vi "myRIO_BRig_RT_v0,62__PortC.vi"() -> ()   [LabVIEW 2014]
uses:
  myRIO_BRig_RT__Case_Exp_stateList.ctl
  myRIO_BRig_RT__Case_NonExp_stateList.ctl
  <vilib>/Platform/TimedLoop/XDataNode/timing_clust.ctl
  <vilib>/Platform/TimedLoop/XDataNode/nitl_modes.ctl
  <vilib>/Platform/TimedLoop/XDataNode/wakeup.ctl
  <vilib>/WebDAVClient/Advanced/SessionHandle.ctl
  <vilib>/myRIO/Common/Instrument Driver Framework/myRIO v1.0/UART/vis/myRIO v1.0 Close UART.vi
  <vilib>/FPGAPlugInAG/myRIO-1900/niLvFpga_Open_myRIO-1900.vi
  <vilib>/rvi/interface/common/dynamic/niFpgaDynamicAddResources.vi
  <vilib>/Utility/error.llb/Error Cluster From Error Code.vi
  <vilib>/rvi/errors/niLvFpgaAdjustHostInterfaceError.vi
  <vilib>/FPGAPlugInAG/Dynamic/niLvFpga_Close_Dynamic.vi
  <vilib>/myRIO/Common/Instrument Driver Framework/Utilities/vis/FPGA Ref Manager.vi
  <vilib>/myRIO/Common/Instrument Driver Framework/myRIO v1.0/myRIO v1.0 Reset FPGA.vi
  <vilib>/myRIO/Common/Instrument Driver Framework/myRIO v1.0/IRQ/vis/myRIO v1.0 IRQ Info FGV.vi
  <vilib>/myRIO/Common/Instrument Driver Framework/myRIO v1.0/IRQ/vis/myRIO v1.0 Timer IRQ Info FGV.vi
  <vilib>/myRIO/Common/Instrument Driver Framework/myRIO v1.0/IRQ/vis/myRIO v1.0 ISR Agent.vi
  <vilib>/rvi/interface/nirviOpenFPGA/nirviOpenFPGA.xnode
  myRIO_BRig_FPGA_v3,52__PortC__build.lvbitx
  myRIO_BRig_FPGA_v3,52__PortC.vi
  <vilib>/rvi/interface/nirviReadWriteControl/nirviReadWriteControl.xnode
  <vilib>/Platform/TimedLoop/XDataNode/XDataNode.xnode
  <vilib>/rvi/interface/nirviCloseFPGA/nirviCloseFPGA.xnode
  <vilib>/Platform/TimedLoop/XDataNode/XDNodeRunTimeDep.lvlib
  <vilib>/rvi/interface/Simulation/niFpgaSimulationCallBeginRW.vi
  <vilib>/myRIO/Instrument Drivers/Utilities/Utilities.lvlib
  <vilib>/WebDAVClient/NI_WebDAV.lvlib
  NiFpgaLv.dll
panel:
  out "error out 5":errorcluster
  in  "get_countPerMS":bool
  in  "count_warmup_R_reset":bool
  in  "count_warmup_L_reset":bool
  out "count_warmup_R":u16
  out "count_warmup_L":u16
  out "SolenoidReward":bool
  in  "SolenoidProbability_L":u16=50 caption="Reward Time [ms]" min=1 max=1000 step=1
  in  "SolenoidProbability_R":u16=50 caption="Reward Time [ms]" min=1 max=1000 step=1
  out "output_PortA":dbl
  out "error out 4":errorcluster
  in  "laser_power_step":dbl
  in  "laser_power_max":dbl
  in  "Recording_p2":bool
  in  "Recording":bool
  out "error out 3":errorcluster
  out "error out 2":errorcluster
  in  "laser_power_min":dbl
  in  "f_millisec2count":dbl=159.0
  in  "laser_Tshutter":dbl=2.0
  in  "laser_Freq":dbl=10.0
  in  "laser_Tpeak":dbl=2.0
  in  "laser_duration":u16
  out "error out":errorcluster
  in  "LC_Cue1_All_Count":u16
  in  "LC_Cue1_First_Count":u16
  in  "LC_Cue1_All_delayOpt":bool
  in  "LC_ENL1_All_delayOpt":bool
  in  "LC_ENL1_All_Count":u16
  in  "LC_ENL1_First_Count":u16
  in  "LC_Cue1_First_delayOpt":bool
  in  "LC_ENL1_First_delayOpt":bool
  in  "Tcycle_Cue_max":u16=1000 caption="Max" min=5 max=5000 step=5
  in  "Tcycle_Cue_min":u16=1000 caption="Min" min=5 max=5000 step=5
  in  "SendData":bool
  out "cSpout":enum16{"Left", "Right"}(ring) caption="Left or Right Spout"
  out "A4":u32 caption="LickCounter_Right"
  out "A2":u32 caption="LickCounter_Left"
  in  "laserResponse_wrong_LED":bool
  out "error_initTrial":errorcluster
  out "error_Selection_pre":errorcluster
  out "error_Selection":errorcluster
  out "SelectWrong":bool
  out "SelectReward":bool
  in  "Left(F)_or_Right(T)":bool
  in  "ignoreWrong":bool
  in  "SelectionState":bool
  in  "laserResponse_wrong":bool
  in  "laserResponse_reward":bool
  in  "laserResponse_reward_LED":bool
  out "nRewards_Right":u16 caption="# Rewards Total (Right)"
  out "nRewards_Left":u16 caption="# Rewards Total (Left)"
  out "nRewards_cur":u16 caption="# Rewards in Current Block"
  out "TpB_target":u16 caption="Target Trials Per Block"
  out "cState_NonExp":T1 caption="WarmUp State"
  out "iBlock":u16 caption="Current Block"
  out "cState":T2 caption="Experimental State"
  out "iTrial":u16 caption="Current Trial"
  in  "warmupType":u8(slide) max=2 step=1 scale=0.0..2.0
  in  "TestConnection":bool
  in  "warmup":bool caption="WarmUp"
  in  "Data Set Prefix":string="Exp1_TM2"
  out "Connected To Host?":bool
  in  "Host Password":string="sabalab"
  in  "Host UserName":string="Test2"
  in  "sp_RightSpout":u16(slide)=2 max=2 step=1 scale=0.0..2.0
  in  "sp_LeftSpout":u16(slide)=2 max=2 step=1 scale=0.0..2.0
  in  "BUR_max":u16 caption="Count Reward Structure  (0 = off)"
  in  "LC_Wrong_Probability":u16
  in  "LC_Wrong_Trial":u16(slide) max=2 step=1 scale=0.0..2.0
  in  "LC_Wrong_Block":u16(slide) max=2 step=1 scale=0.0..2.0
  in  "LC_Wrong_OnOff":bool
  in  "LC_Reward_Probability":u16
  in  "LC_Reward_Trial":u16(slide) max=2 step=1 scale=0.0..2.0
  in  "LC_Reward_Block":u16(slide) max=2 step=1 scale=0.0..2.0
  in  "LC_Reward_OnOff":bool
  in  "LC_Cue1_All_Probability":u16
  in  "LC_Cue1_All_Block":u16(slide) max=2 step=1 scale=0.0..2.0
  in  "LC_Cue1_All_OnOff":bool
  in  "LC_Cue1_First_Probability":u16
  in  "LC_Cue1_First_Block":u16(slide) max=2 step=1 scale=0.0..2.0
  in  "LC_Cue1_First_OnOff":bool
  in  "LC_ENL1_All_Probability":u16 max=100 step=1
  in  "LC_ENL1_All_Block":u16(slide) max=2 step=1 scale=0.0..2.0
  in  "LC_ENL1_All_OnOff":bool
  in  "LC_ENL1_First_Probability":u16 max=100 step=1
  in  "LC_ENL1_First_Block":u16(slide) max=2 step=1 scale=0.0..2.0
  in  "Tcycle_Timeout":u16=1000 caption="Timeout Time [ms]" min=10 max=10000 step=1
  in  "Tcycle_Wrong":u16=1000 caption="Wrong Time [ms]" min=10 max=10000 step=1
  in  "Tcycle_Selection":u16=1000 caption="Answer Time [ms]" min=1 max=10000 step=1
  in  "Tcycle_RewardPost":u16=1000 caption="Consumption Time [ms]" min=250 max=10000 step=250
  in  "Tcycle_Reward_L":u16=500 caption="Reward Time [ms]" min=1 max=1000 step=1
  in  "Tcycle_Reward_R":u16=500 caption="Reward Time [ms]" min=1 max=1000 step=1
  in  "TpB_Max_R":u16=4 caption="Max TrialsPerBlock" min=1 max=12 step=1
  in  "TpB_Min_R":u16=4 caption="Min TrialsPerBlock" min=1 max=12 step=1
  in  "TpB_Max_L":u16=4 caption="Max TrialsPerBlock" min=1 max=12 step=1
  in  "TpB_Min_L":u16=4 caption="Min TrialsPerBlock" min=1 max=12 step=1
  in  "BUR_min":u16 caption="Count Reward Structure  (0 = off)"
  in  "TrialUntilReward":bool caption="Ignore Wrong Selection"
  in  "CueCycles":u16=1 caption="Cue Structure" min=1 max=1 step=1
  in  "MTrig_Laser_Tcycle":u16=10 caption="Time [ms]"
  in  "MTrig_Laser_trig":bool
  in  "MTrig_Audio_trig__R":bool caption="Trigger Audio"
  in  "MTrig_Audio_trig__L":bool caption="Trigger Audio"
  in  "RewCalib_Trig_R":bool caption="Calibrate_R"
  in  "RewCalib_Trig_L":bool caption="Calibrate_L"
  in  "MTrig_Solenoid_Tcycle__R":u16=300 caption="Time [ms]"
  in  "MTrig_Solenoid_Tcycle__L":u16=300 caption="Time [ms]"
  in  "MTrig_Solenoid_trig__R":bool caption="Solenoid"
  in  "MTrig_Solenoid_trig__L":bool caption="Solenoid"
  in  "STOP_abort":bool caption="Stop LabView\n(Stops myRio and FPGA)"
  in  "STOP_endBlock":bool caption="Stop Experiment\n@ End of Block"
  in  "STOP_endTrial":bool caption="Stop Experiment\n@ End of Trial"
  in  "START":bool caption="Start Experiment"
  in  "Tcycle_CuePenalty":u16=1000 caption="Penalty" min=1 max=10000 step=1
  in  "Audio_Amp__R":u16=100 caption="Amp"
  in  "Audio_Freq__R":u8=5 caption="Freq [kHz]" max=14 step=1
  in  "Audio_Amp__L":u16=100 caption="Amp"
  in  "Audio_Freq__L":u8=5 caption="Freq [kHz]" max=14 step=1
  in  "LC_Wrong_Tdelay":u16
  in  "LC_Cue1_All_Tdelay":u16
  in  "LC_ENL1_All_Tdelay":u16
  in  "LC_Reward_Tdelay":u16
  in  "LC_Cue1_First_Tdelay":u16
  in  "LC_ENL1_First_Tdelay":u16
  in  "LC_ENL1_First_OnOff":bool
  in  "Tcycle_ENLPenalty":u16=100 caption="Penalty" min=10 max=10000 step=10
  in  "Tcycle_ENL_max":u16=1000 caption="Max" min=250 max=10000 step=250
  in  "Tcycle_ENL_min":u16=1000 caption="Min" min=250 max=10000 step=250
  # "Communication (Host PC)"
  # "WarmUp"
  # "Experimental Run"
  # "Current State"
  # "Laser Control\n\n                               On/Off      Block        Probability [%]   Delay [ms]                              Count"
  # "Cue then reward (no lick)\n \nLeft                    Right"
  # "Recording Rig"
  # "FPGA Conv."
  # "Enforced\nNonLick\n      1"
  # "from end"
  # "Switch\nTrial"
  # "FPGA count per ms"
  # "from start"
  # "from end"
  # "NonSwitch\nTrials"
  # "from start"
  # "Manual Control"
  # "Cue 1"
  # "Solenoid\n \nLeft                    Right"
  # "Speaker\n \nLeft                    Right"
  # "Laser"
  # "from end"
  # "Switch\nTrial"
  # "from start"
  # "from end"
  # "NonSwitch\nTrials"
  # "from start"
  # "Time = Cue Min"
  # "Selection Reward"
  # "Power = Min"
  # "Task Timing [ms]"
  # "Speaker Settings"
  # "Laser Settings"
  # "Selection Wrong"
  # "Left                  Right"
  # "Enforced NonLick"
  # "Frequency\n[kHz]"
  # "Duration         Frequency       Peak Width           Shutter\n    [ms]                   [Hz]                    [ms]                    [ms]"
  # "Task Structure"
  # "Spout Selection Control"
  # "Amp\n(0 - 32,000)"
  # "Master Structure"
  # "Cue"
  # "Answer Time\n         [ms]\n\n  \nWrong Choice Penalty\n         [ms]\n \n \nChoice Timeout Penalty\n         [ms]"
  # "Min\n \n  \nMax"
  # "Laser Power [V]\n      Min                   Max                   Step                 Current"
  # "Speaker\nPattern\nDuring Cue"
  # "(1) = Switching\n(2) = Two Choice"
  # "Reward Control\n                 Left              Right"
  # "Min"
  # "Max"
  # "Trial Per Block Structure\n       Left                    Right"
  # "Reward Time\n         [ms]\n\nWater Prob"
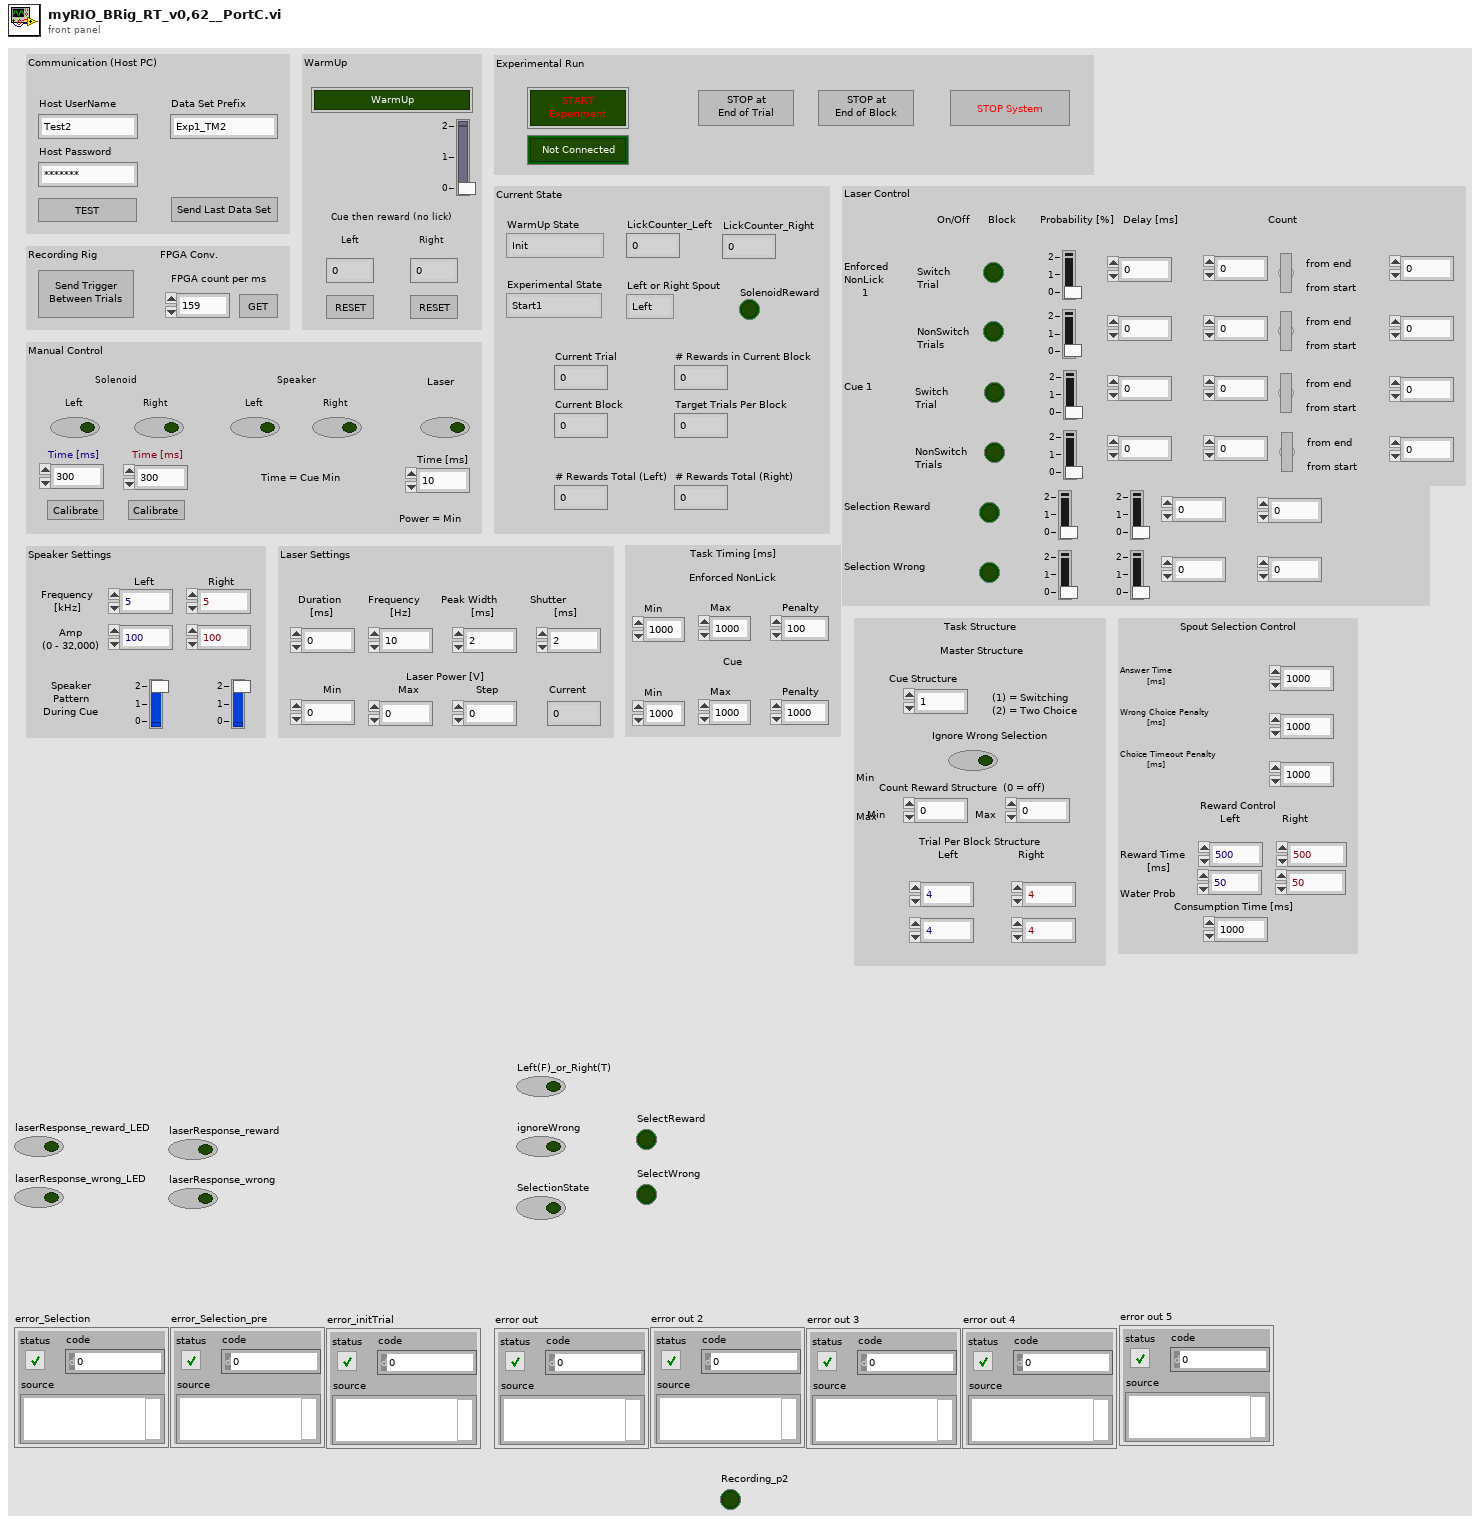
[diagram p1: front panel]
types:
  T1 = typedef "myRIO_BRig_RT__Case_NonExp_stateList.ctl" = enum16{"Init", "UploadSettings_pre", "UploadSettings_Read_dataExp", "UploadSettings_dataExp_1", "UploadSettings_Read_dataLC", "UploadSettings_dataLC_1", "UploadSettings_dataLC_2", "UploadSettings_Read_dataMTrig", "UploadSettings_dataMTrig_1", "UploadSettings_post", "Idle_pre", "IdleEmpty", "IdleEmpty2", "IdleEmpty3", "IdleEmpty4", "Idle", "Idle_2", "Idle_3", "Idle_4", "Idle_post", "Cue_pre__pre", "Cue_pre", "Cue", "Cue_post", "RewardCalibration_pre", "DispenseWater_pre__pre", "DispenseWater_pre", "DispenseWater", "DispenseWater_post", "TestConnection", "SendData", "Get_FPGA_count_per_ms", "End"}
  T2 = typedef "myRIO_BRig_RT__Case_Exp_stateList.ctl" = enum16{"Start1", "Start2", "Start3", "saveSettings1", "saveSettings2", "saveSettings3", "saveSettings4_LC_ENL", "saveSettings5_LC_Cue", "saveSettings6_LC_Other", "setSettings_Audio", "setSettings_Laser", "initBlock_pre", "initBlock", "initBlock2", "initBlock_post", "initTrial_pre", "initTrial", "initTrial2", "initTrial3", "initTrial4", "initTrial_LC_ENL1", "initTrial_LC_Cue1", "initTrial_post", "ENL1_pre", "ENL1", "ENL1_post", "ENL1Penalty_pre", "ENL1Penalty", "ENL2_pre", "ENL2", "ENL2Penalty_pre", "ENL2Penalty", "Cue1_pre", "Cue1", "Cue1_post", "Cue1Penalty_pre", "Cue1Penalty", "Cue2_pre", "Cue2", "Cue2Penalty_pre", "Cue2Penalty", "Selection_pre", "Selection", "Select_post", "SelectReward_pre", "SelectReward", "SelectRewardPost_pre", "SelectRewardPost", "SelectWrong_pre", "SelectWrong", "SelectWrong_post", "SelectTimeout_pre", "SelectTimeout", "SelectTimeout_post", "endTrial_pre", "endTrial1", "endTrial2", "endTrial3", "endTrial_post", "endBlock_pre", "endBlock", "endBlock_post", "endExp", "commConnect", "commUpload_pre", "commUpload_dataBlock", "commUpload_dataCurrent", "commUpload_dataExp", "commUpload_dataLC", "commUpload_dataTrial", "commUpload_post", "saveData_pre", "saveData_dataBlock", "saveData_dataCurrent", "saveData_dataExp", "saveData_dataLC", "saveData_dataTrial", "saveData_post", "empty_endBlock1", "empty_endBlock2", "empty_endTrial1", "empty_endTrial2", "empty_endTrial3", "empty_endTrial4", "empty_endTrial5"}
  T3 = typedef "XDNodeRunTimeDep.lvlib/timing_clust.ctl" = cluster{"Expected End [f-1]":u64, "Actual End [f-1]":u64, "Finished Late? [f-1]":bool, "Expected End [i-1]":u64, "Actual End [i-1]":u64, "Finished Late? [i-1]":bool, "Expected Start [i]":u64, "Actual Start [i]":u64, "Expected Start [f]":u64, "Actual Start [f]":u64, "Source Name":string, "Structure Name":string, "Period":i64, "Deadline":i64, "Offset":i64, "Start":i64, "Priority":i32, "Timeout":i32, "Mode":T4, "Wakeup Reason":T5, "Error":errorcluster, "Source Type":string, "Secondary Source Type":string, "Global End Time":u64, "Global Start Time":u64, "Frame Duration":u64, "Iteration Duration":u64, "Assigned CPU":i32, "I/O Scan Engine Mode":u32}
  T4 = typedef "XDNodeRunTimeDep.lvlib/nitl_modes.ctl" = enum32{"No Change", "Process missed periods, maintain original phase", "Discard missed periods, maintain original phase", "Process missed periods, ignore original phase", "Discard missed periods, ignore original phase"}
  T5 = typedef "XDNodeRunTimeDep.lvlib/wakeup.ctl" = enum32{"Normal", "Aborted", "Asynchronous wakeup", "Timing source error", "Timed loop error", "Timeout"}
  T6 = typedef "NI_WebDAV.lvlib/SessionHandle.ctl" = refnum<k1>
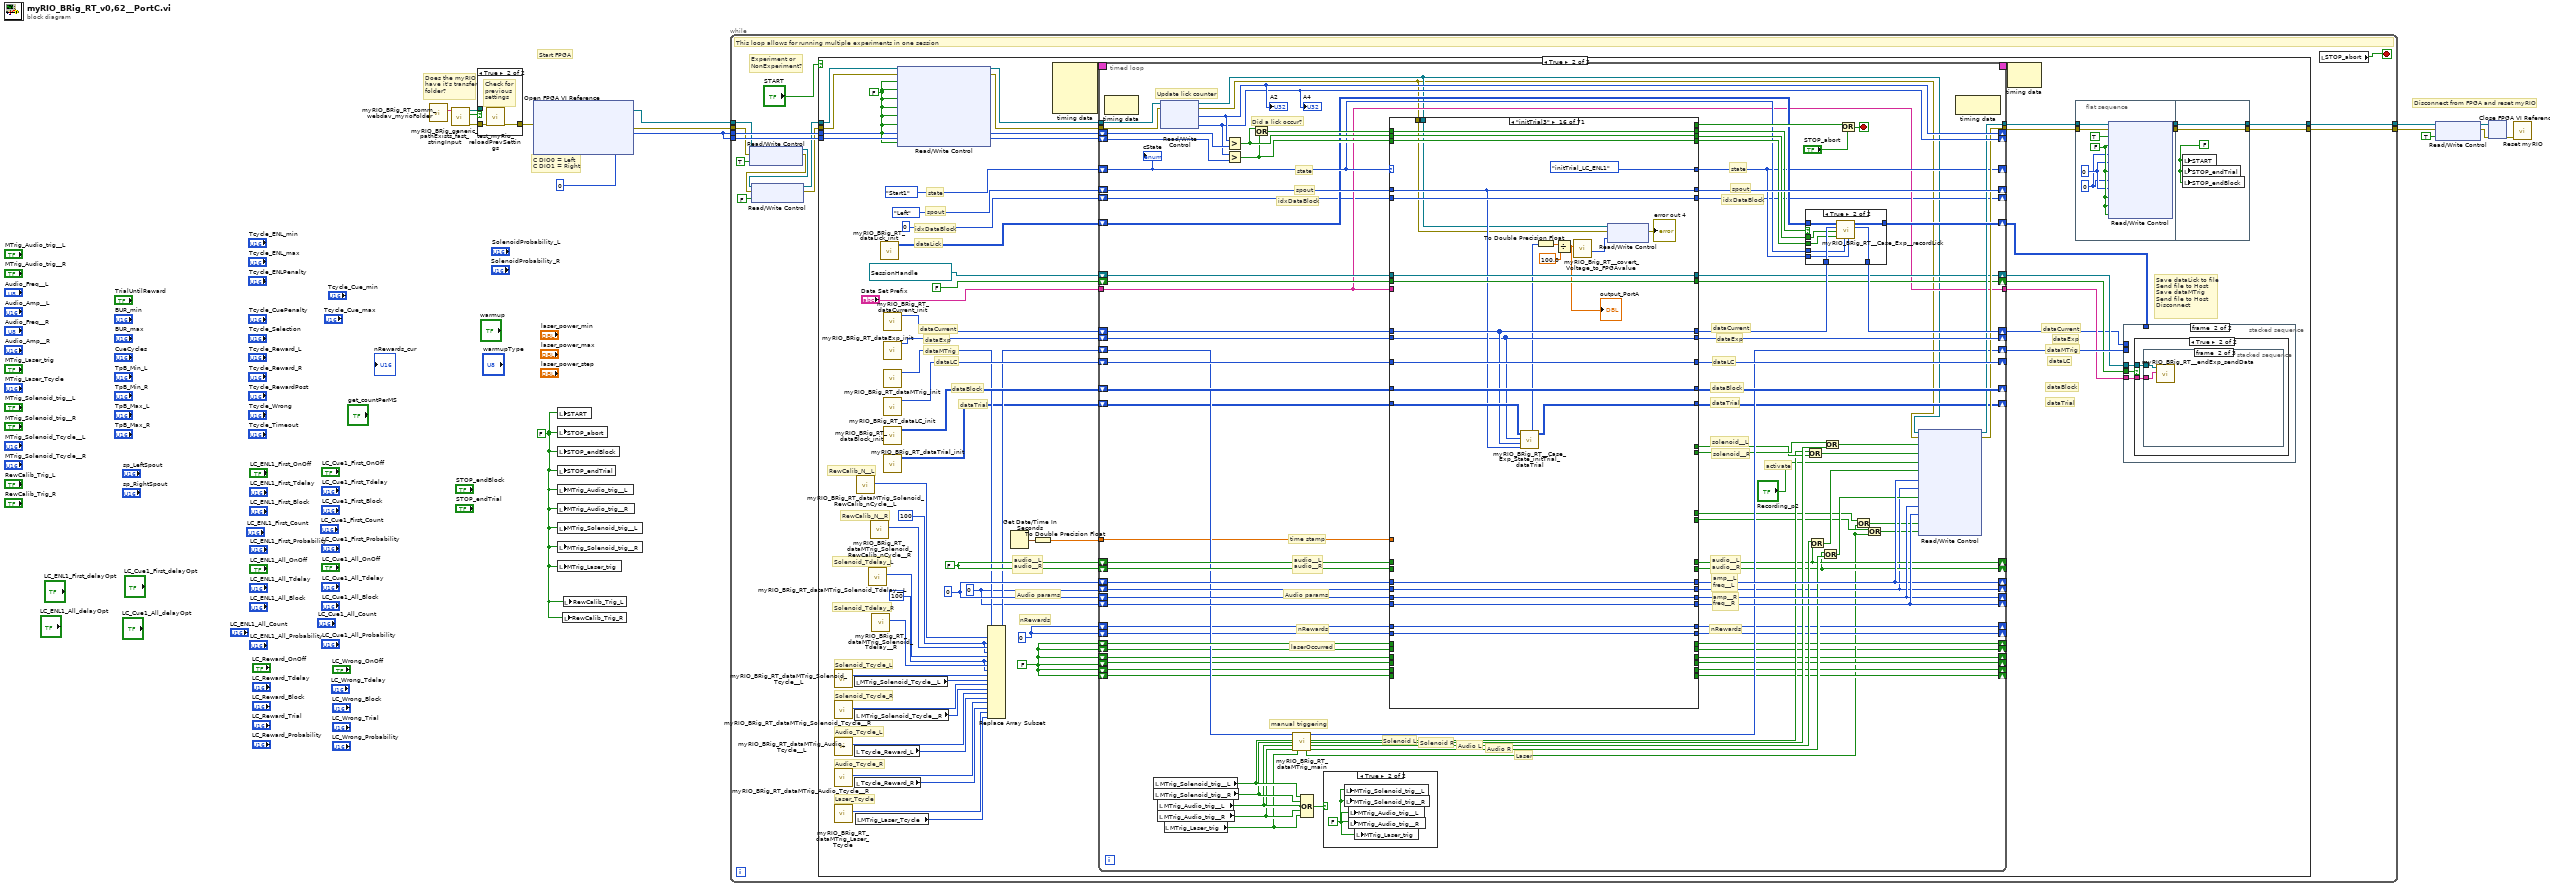
[diagram p0: block diagram]
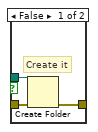
[diagram p2: hidden frame]
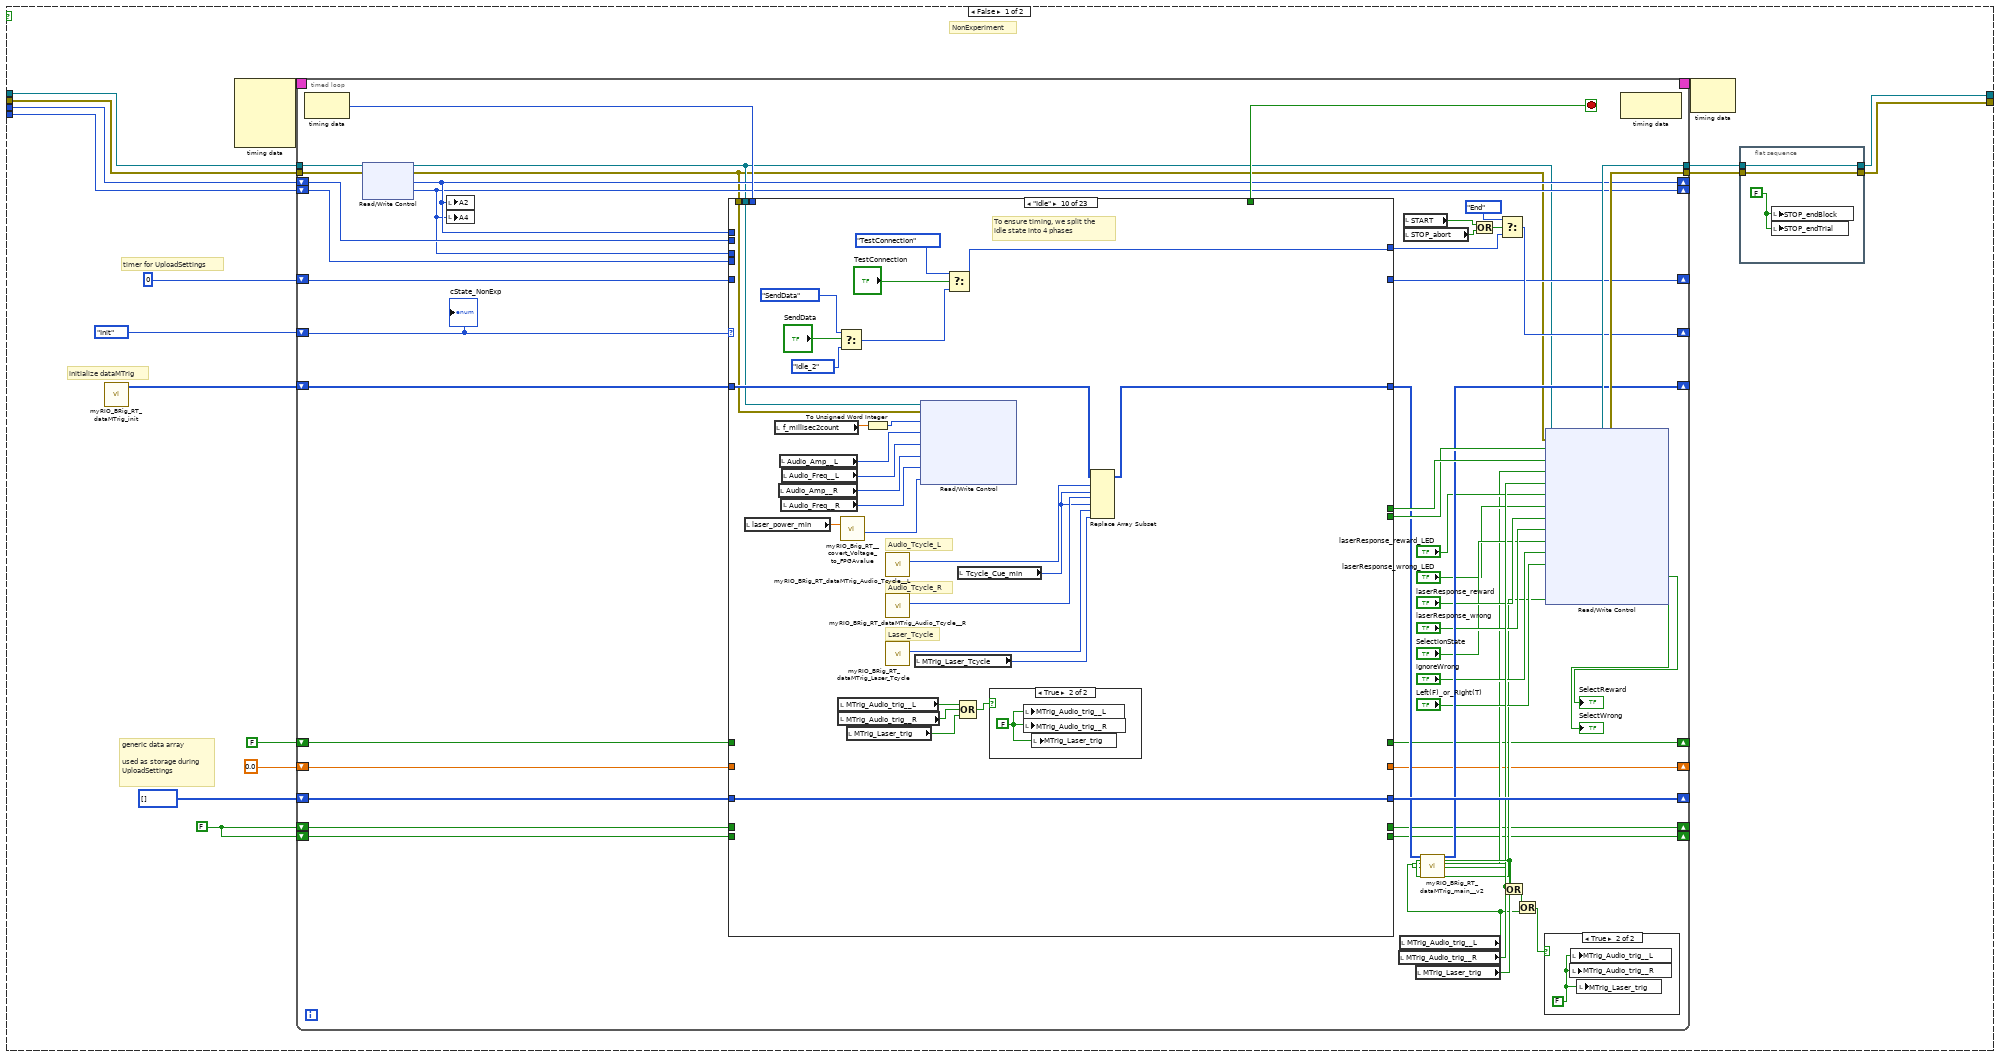
[diagram p3: hidden frame]
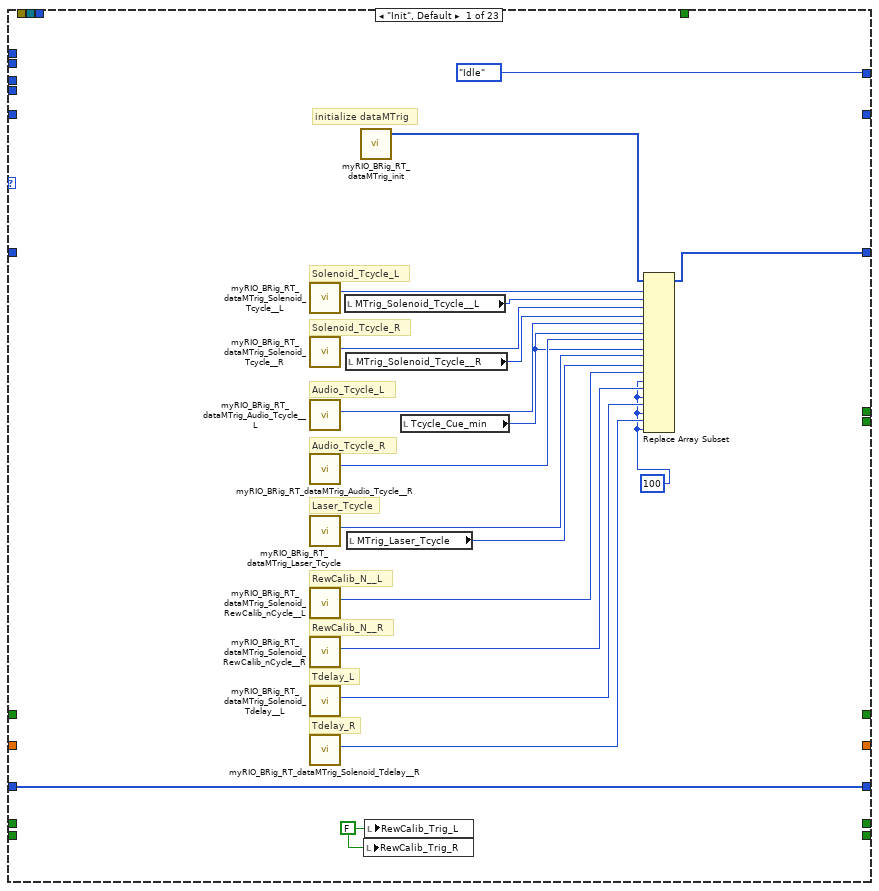
[diagram p5: hidden frame]
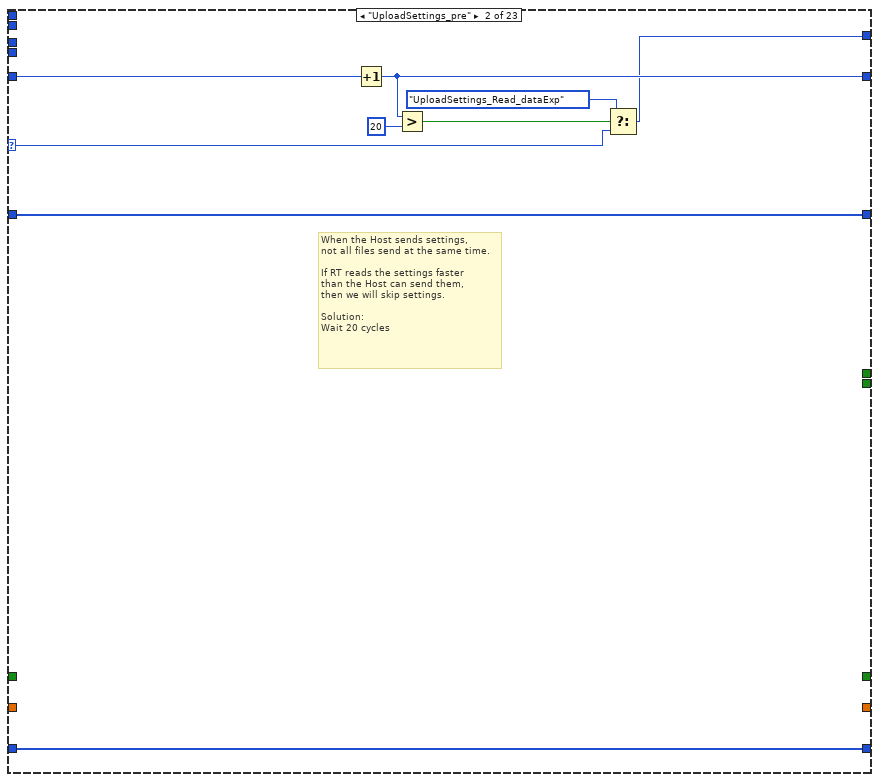
[diagram p6: hidden frame]
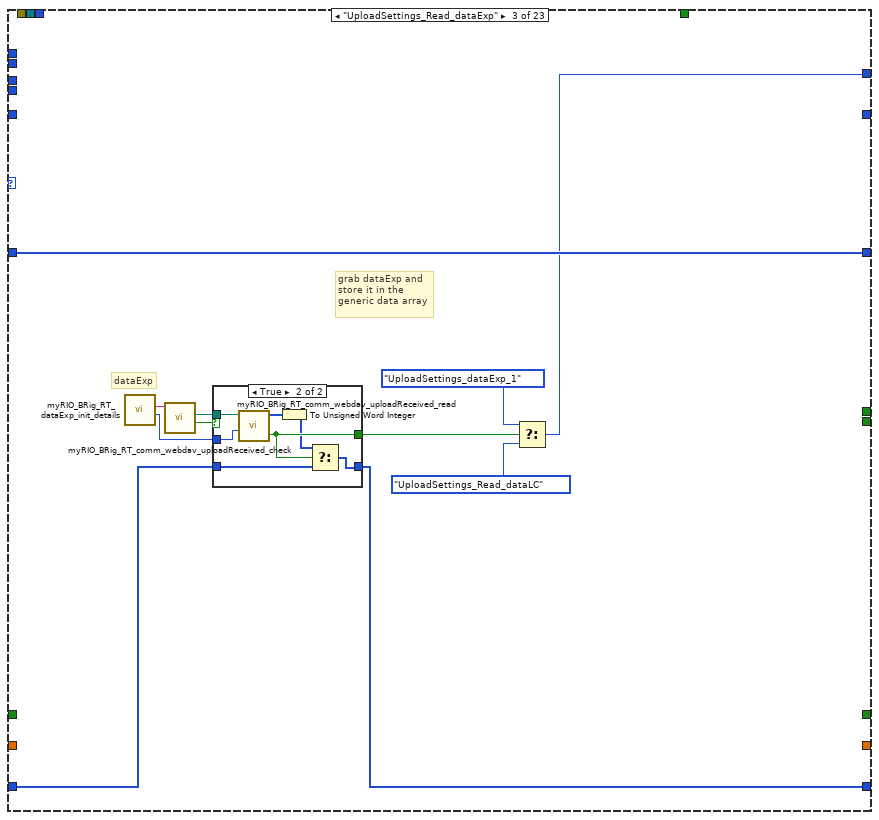
[diagram p7: hidden frame]
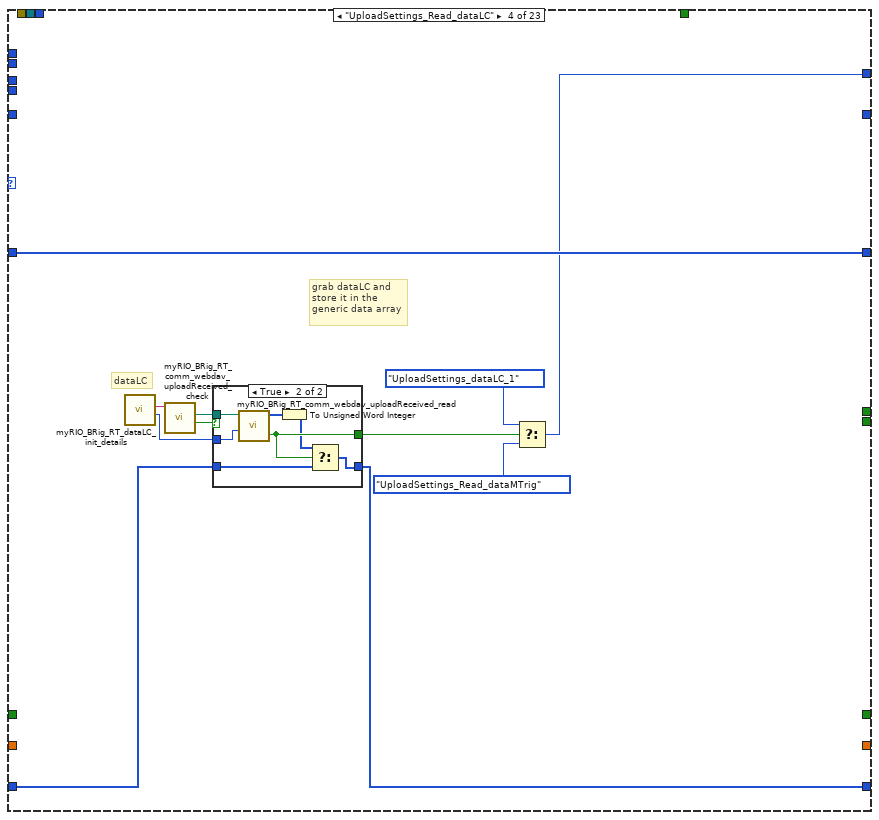
[diagram p9: hidden frame]
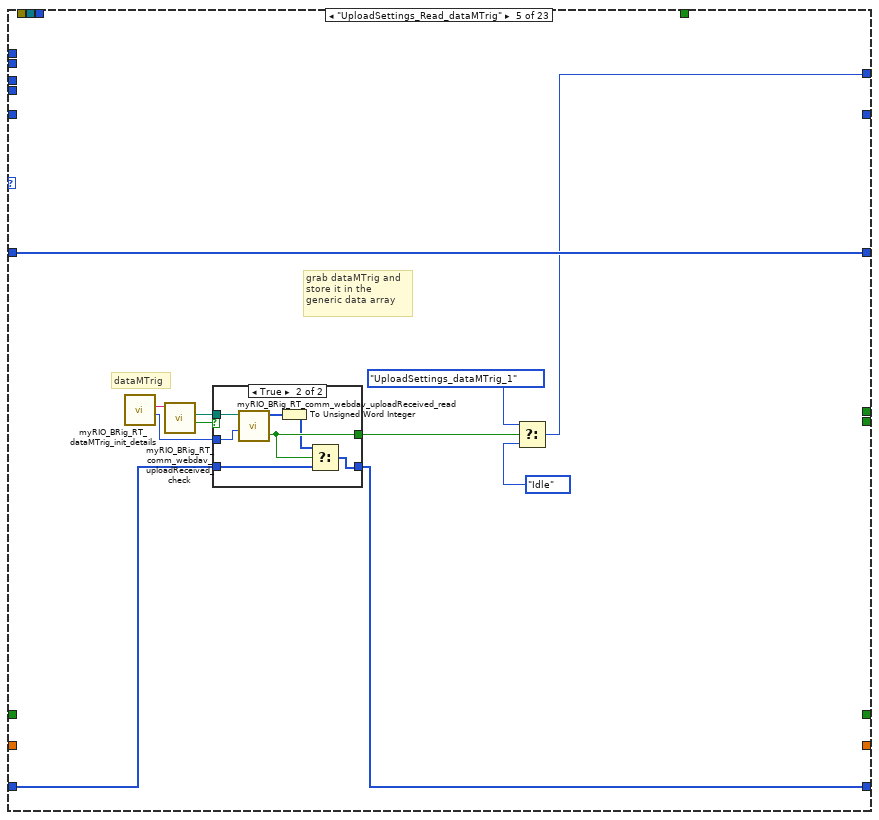
[diagram p11: hidden frame]
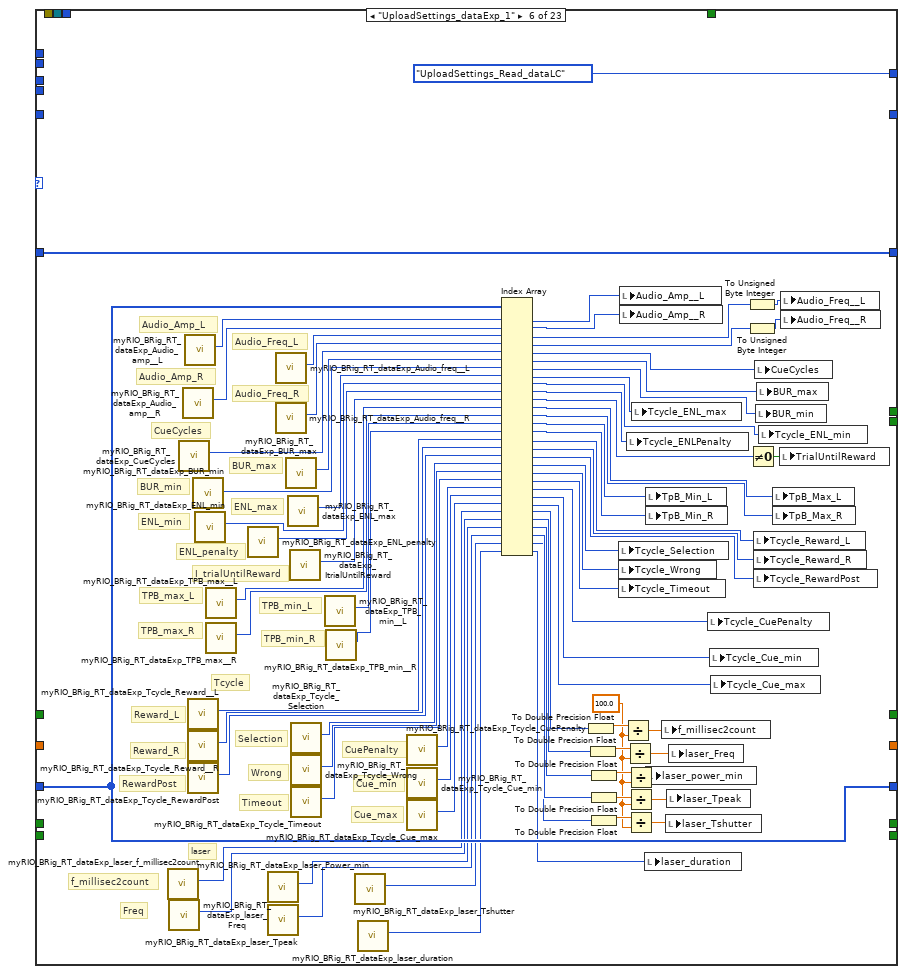
[diagram p13: hidden frame]
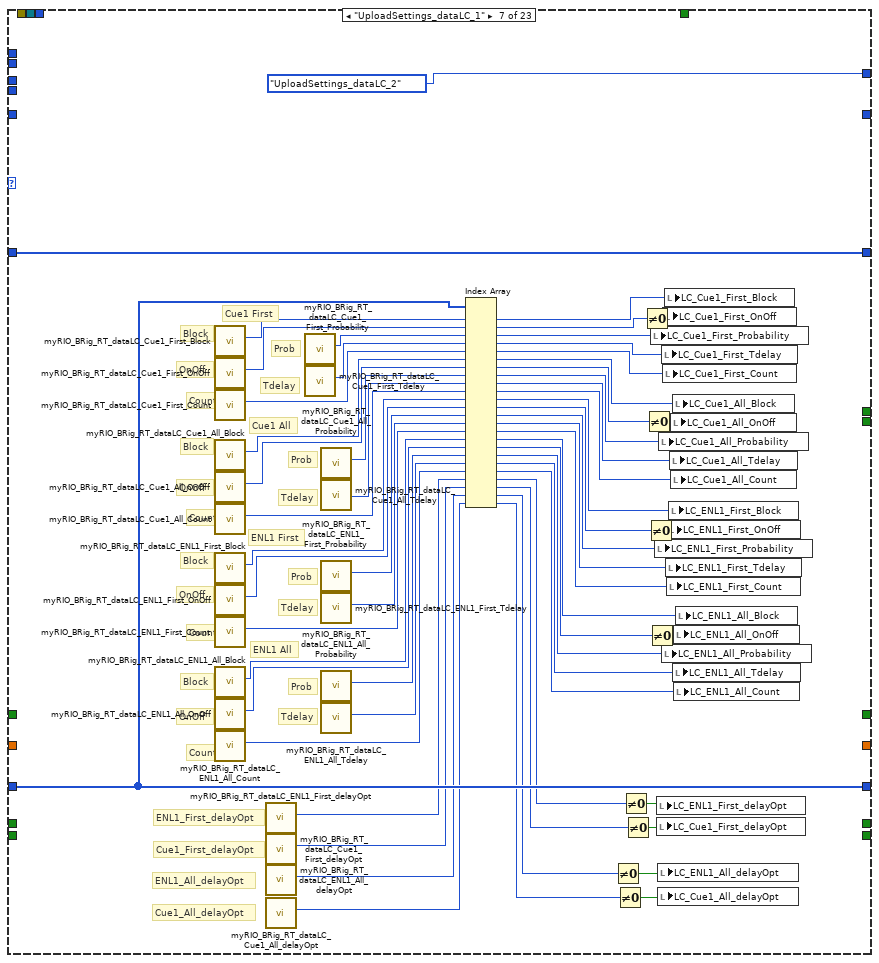
[diagram p14: hidden frame]
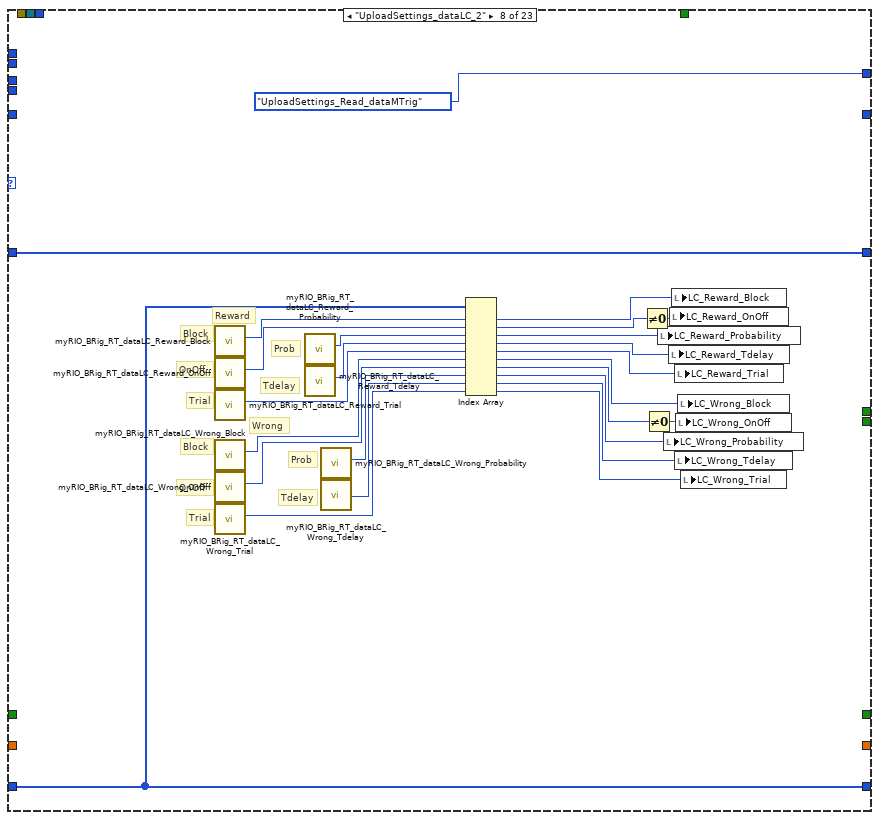
[diagram p15: hidden frame]
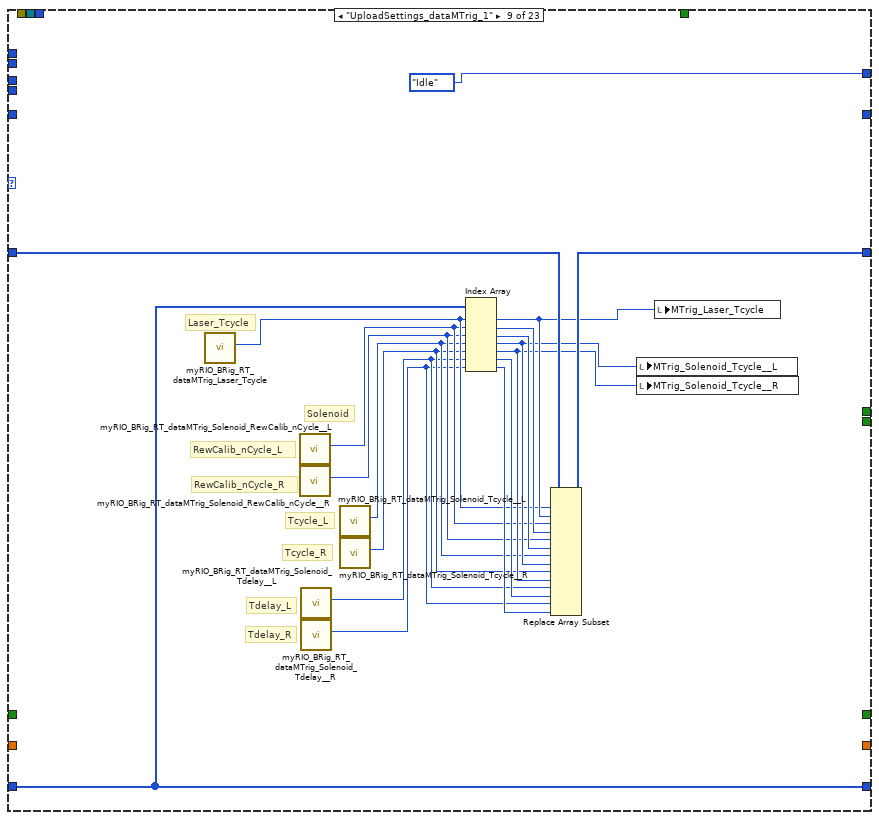
[diagram p16: hidden frame]
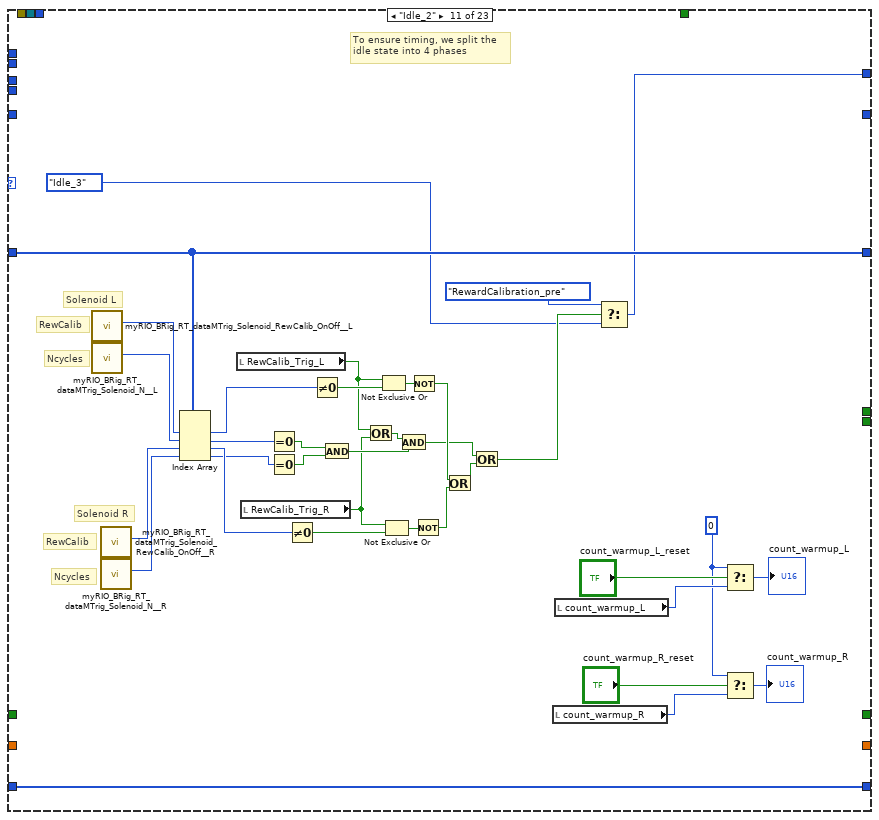
[diagram p18: hidden frame]
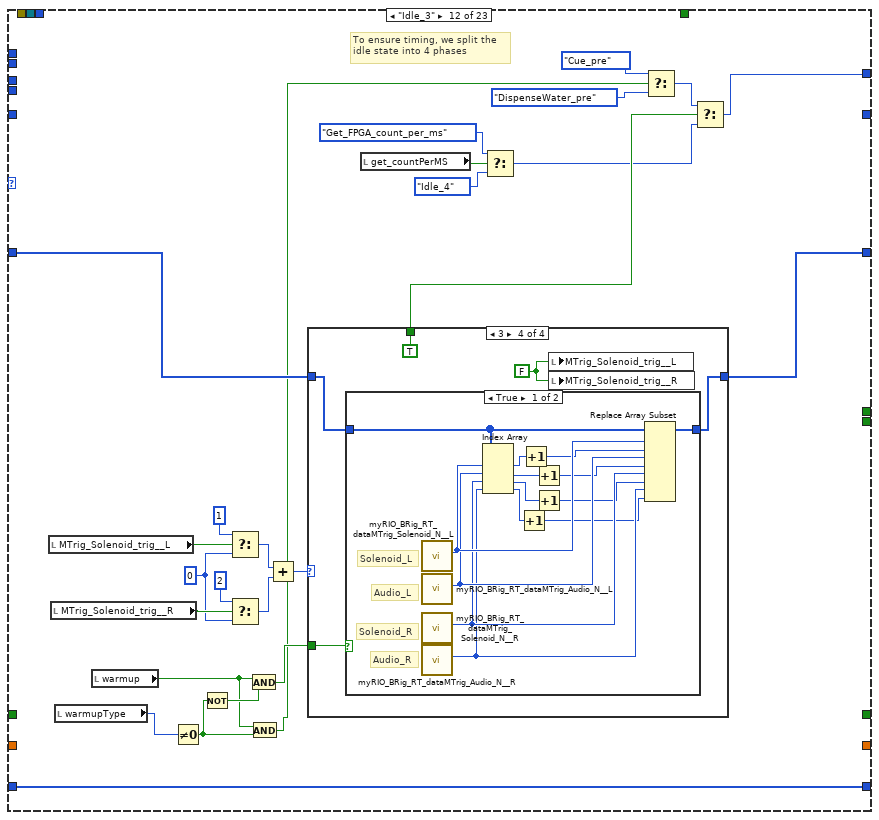
[diagram p19: hidden frame]
diagram:
  w9 = u32 0
  w6 = FALSE
  # "Does the myRIO\nhave it's transfer\nfolder?"
  # "C DIO0 = Left\nC DIO1 = Right"
  # "Start FPGA"
  # "Disconnect from FPGA and reset myRIO"
  n1 = call "myRIO_BRig_RT_comm_webdav_myrioFolder.vi"() -> ("output_myrioFolder"=w4:string)  [unwired: 11 in]
  n2 = call "myRIO_BRig_generic_pathExists_fast_stringInput.vi"("input_filePath"=w4) -> ("output_error"=w3:errorcluster, "output_Iexist"=w2:bool, "output_filePath"=w1:path)  [unwired: 8 in]
  n3 = case shown="True" w2 {
    tunnel: w1 -> [w18 _]
    tunnel: w3 -> [w17 w20]
    tunnel: [w16 w19] -> w5
    frame False {
      # "Create it"
      n4 = Create Folder(path (use dialog)=w18, error in=w17) -> (error out=w16:errorcluster)  [unwired: 1 in, 2 out]
    }
    frame True {
      # "Check for\nprevious\nsettings"
      n5 = call "test_myRio_reloadPrevSettings.vi"("input_error"=w20) -> ("output_error"=w19:errorcluster)  [unwired: 10 in]
    }
  }
  n6 = xnode "Open FPGA VI Reference"("error in"=w5) -> ("FPGA VI Reference Out"=w11:refnum<k20>, "error out"=w10:errorcluster)  [unwired: 1 in]
  n7 = local write "START"(w6) -> ()
  n8 = local write "STOP_abort"(w6) -> ()
  n9 = local write "STOP_endBlock"(w6) -> ()
  n10 = local write "STOP_endTrial"(w6) -> ()
  n11 = local write "MTrig_Audio_trig__L"(w6) -> ()
  n12 = local write "MTrig_Audio_trig__R"(w6) -> ()
  n13 = local write "MTrig_Solenoid_trig__L"(w6) -> ()
  n14 = local write "MTrig_Solenoid_trig__R"(w6) -> ()
  n15 = local write "MTrig_Laser_trig"(w6) -> ()
  n16 = local write "RewCalib_Trig_R"(w6) -> ()
  n17 = local write "RewCalib_Trig_L"(w6) -> ()
  n18 = while {
    tunnel: w11 -> [w24]
    tunnel: w10 -> [w29]
    tunnel: w9 -> [w32]
    tunnel: w9 -> [w31]
    tunnel: [w22] -> w8
    tunnel: [w21] -> w7
    stop <- w30 stop-if-true
    # "Experiment or\nNonExperiment?"
    # "This loop allows for running multiple experiments in one session"
    n19 = xnode "Read/Write Control"("FPGA VI Reference In"=w24, "error in"=w29, "Counts_Reset"=TRUE) -> ("FPGA VI Reference Out"=w26:refnum<k20>, "error out"=w27:errorcluster)
    n20 = xnode "Read/Write Control"("FPGA VI Reference In"=w26, "error in"=w27, "Counts_Reset"=FALSE) -> ("FPGA VI Reference Out"=w23:refnum<k20>, "error out"=w25:errorcluster)
    n21 = case shown="True" "START" {
      tunnel: w32 -> [w47 w950]
      tunnel: w31 -> [w46 w949]
      tunnel: w25 -> [w44 w900]
      tunnel: w23 -> [w45 w899]
      tunnel: [w42 w946] -> w22
      tunnel: [w40 w941] -> w21
      frame False {
        w37 = FALSE
        # "generic data array\n\nused as storage during\nUploadSettings"
        # "timer for UploadSettings"
        # "initialize dataMTrig"
        # "NonExperiment"
        n22 = call "myRIO_BRig_RT_dataMTrig_init.vi"() -> ("output_dataMTrig"=w48:u16[])  [unwired: 5 in]
        n23 = node-c288() -> (w51:T3)  [unwired: 4 in]
        n24 = timed-loop {
          timing: w51 -> [_]
          timing-out: [_] -> w50
          shift-right: [w94] -> _
          shift-left: w48 -> [w106]
          shift-right: [w83] -> _
          shift-left: myRIO_BRig_RT__Case_NonExp_stateList."Init" ("Enum") -> [w100]
          shift-right: [w67] -> _
          shift-left: w47 -> [w68]
          shift-right: [w65] -> _
          shift-left: w46 -> [w66]
          tunnel: [w102] -> w43
          tunnel: [w101] -> w41
          tunnel: w44 -> [w104]
          tunnel: w45 -> [w103]
          shift-right: [w99] -> _
          shift-left: u16[] [] ("output_data") -> [w98]
          shift-right: [w69] -> _
          shift-left: u16 0 ("Audio_Amp__L") -> [w70]
          shift-right: [w62] -> _
          shift-left: w37 -> [w64]
          shift-right: [w61] -> _
          shift-left: w37 -> [w63]
          shift-right: [w57] -> _
          shift-left: FALSE -> [w58]
          shift-right: [w55] -> _
          shift-left: 0.0 -> [w56]
          stop <- w107 stop-if-true
          n25 = node-c288() -> (w105:i64)  [unwired: 1 in]
          n26 = xnode "Read/Write Control"("FPGA VI Reference In"=w103, "error in"=w104) -> ("FPGA VI Reference Out"=w60:refnum<k20>, "error out"=w59:errorcluster, "A2_LickL"=w67:u32, "A4_LickR"=w65:u32)
          n27 = local write "A2"(w67) -> ()
          n28 = local write "A4"(w65) -> ()
          n29 = case shown="\"Idle\"" w100 {
            selector: w100 -> [_ w132 _ _ _ _ _ _ _ _ _ _ _ _ w563 _ _ w771 _ _ _ w846 w890]
            tunnel: [myRIO_BRig_RT__Case_NonExp_stateList."Idle" ("Enum") w130 w137 w156 w175 myRIO_BRig_RT__Case_NonExp_stateList."UploadSettings_Read_dataLC" ("Enum") myRIO_BRig_RT__Case_NonExp_stateList."UploadSettings_dataLC_2" ("Enum") myRIO_BRig_RT__Case_NonExp_stateList."UploadSettings_Read_dataMTrig" ("f") myRIO_BRig_RT__Case_NonExp_stateList."Idle" ("Enum") w394 w411 w450 w531 myRIO_BRig_RT__Case_NonExp_stateList."Cue" ("t") w558 myRIO_BRig_RT__Case_NonExp_stateList."DispenseWater_pre" ("Enum") w716 w769 w792 myRIO_BRig_RT__Case_NonExp_stateList."Idle" ("Enum") myRIO_BRig_RT__Case_NonExp_stateList."Idle" ("Enum") w845 w890] -> w84
            tunnel: [w119 w129 w147 w166 w185 w270 w329 w354 w370 w398 w426 w455 w529 w547 w564 w626 w753 w776 w803 w838 w844 w857 w888] -> w95
            tunnel: [_ _ _ _ _ _ _ _ _ _ _ _ _ _ _ _ _ _ _ _ _ _ TRUE] -> w107
            tunnel: w106 -> [_ w129 w147 w166 w185 w270 w329 w354 w371 w397 w426 w456 w529 w548 w565 w612 w749 w777 w804 w838 w844 w857 w888]
            tunnel: w105 -> [_ _ _ _ _ _ _ _ _ _ _ _ _ _ _ _ _ w781 _ _ _ _ _]
            tunnel: [w112 w128 w138 w157 w176 w219 w285 w330 w355 w389 w410 w444 w528 w537 w572 w607 w701 w754 w785 w830 w842 w856 w887] -> w99
            tunnel: w98 -> [w112 w128 w139 w158 w177 w219 w285 w330 w355 w389 w410 w444 w528 w537 w572 w607 w701 w754 w785 w830 w842 w856 w887]
            tunnel: [_ _ _ _ _ _ _ _ _ _ _ _ _ _ _ _ _ w778 _ _ _ _ _] -> w97
            tunnel: [_ _ _ _ _ _ _ _ _ _ _ _ _ _ _ _ _ w760 _ _ _ _ _] -> w96
            tunnel: w70 -> [_ w136 _ _ _ _ _ _ _ _ _ _ _ _ _ _ _ _ _ _ _ _ _]
            tunnel: [_ w135 _ _ _ _ _ _ _ _ _ _ _ _ _ _ _ _ _ _ _ _ _] -> w69
            tunnel: w68 -> [_ _ _ _ _ _ _ _ _ _ _ _ _ _ w569 _ _ _ _ _ _ _ _]
            tunnel: w67 -> [_ _ _ _ _ _ _ _ _ _ _ _ _ _ w570 _ _ _ _ _ _ _ _]
            tunnel: w66 -> [_ _ _ _ _ _ _ _ _ _ _ _ _ _ w567 _ _ _ _ _ _ _ _]
            tunnel: w65 -> [_ _ _ _ _ _ _ _ _ _ _ _ _ _ w568 _ _ _ _ _ _ _ _]
            tunnel: w64 -> [_ _ _ _ _ _ _ _ _ _ _ _ _ _ w555 _ _ _ _ _ _ _ _]
            tunnel: w63 -> [_ _ _ _ _ _ _ _ _ _ _ _ _ _ w554 _ _ _ _ _ _ _ _]
            tunnel: [_ _ _ _ _ _ _ _ _ _ _ _ _ w536 w555 _ _ _ _ _ _ _ _] -> w62
            tunnel: [_ _ _ _ _ _ _ _ _ _ _ _ _ w535 w554 _ _ _ _ _ _ _ _] -> w61
            tunnel: w60 -> [_ _ _ _ _ _ _ _ _ w380 _ _ _ _ _ _ _ _ _ _ _ w851 _]
            tunnel: w59 -> [_ _ _ _ _ _ _ _ _ w379 _ _ _ _ _ _ _ _ _ _ _ w850 _]
            tunnel: w58 -> [_ _ _ _ _ _ _ _ _ _ _ _ _ _ _ _ _ _ _ _ _ w855 _]
            tunnel: [_ _ _ _ _ _ _ _ _ _ _ _ _ _ _ _ _ _ _ _ _ TRUE _] -> w57
            tunnel: w56 -> [_ _ _ _ _ _ _ _ _ _ _ _ _ _ _ _ _ _ _ _ _ w853 _]
            tunnel: [_ _ _ _ _ _ _ _ _ _ _ _ _ _ _ _ _ _ _ _ _ w852 _] -> w55
            frame "Init", Default {
              w113 = FALSE ("RewCalib_Trig_L")
              w109 = u16 100 ("new element/subarray")
              # "Tdelay_R"
              # "Tdelay_L"
              # "RewCalib_N__R"
              # "RewCalib_N__L"
              # "Solenoid_Tcycle_R"
              # "Solenoid_Tcycle_L"
              # "Laser_Tcycle"
              # "Audio_Tcycle_R"
              # "Audio_Tcycle_L"
              # "initialize dataMTrig"
              n30 = call "myRIO_BRig_RT_dataMTrig_Solenoid_Tcycle__L.vi"() -> ("output_Solenoid_Tcycle__L"=w121:i32)  [unwired: 11 in]
              n31 = call "myRIO_BRig_RT_dataMTrig_Solenoid_Tcycle__R.vi"() -> ("output_Solenoid_Tcycle__R"=w122:i32)  [unwired: 11 in]
              n32 = call "myRIO_BRig_RT_dataMTrig_Audio_Tcycle__L.vi"() -> ("output_Audio_Tcycle__L"=w123:i32)  [unwired: 11 in]
              n33 = call "myRIO_BRig_RT_dataMTrig_Audio_Tcycle__R.vi"() -> ("output_Audio_Tcycle__R"=w124:i32)  [unwired: 11 in]
              n34 = call "myRIO_BRig_RT_dataMTrig_Laser_Tcycle.vi"() -> ("output_Laser_Tcycle"=w125:i32)  [unwired: 11 in]
              n35 = call "myRIO_BRig_RT_dataMTrig_Solenoid_RewCalib_nCycle__L.vi"() -> ("output_Solenoid_RewCalib_nCycle__L"=w117:i32)  [unwired: 11 in]
              n36 = call "myRIO_BRig_RT_dataMTrig_Solenoid_RewCalib_nCycle__R.vi"() -> ("output_Solenoid_RewCalib_nCycle__R"=w116:i32)  [unwired: 11 in]
              n37 = call "myRIO_BRig_RT_dataMTrig_Solenoid_Tdelay__L.vi"() -> ("output_Solenoid_Tdelay__L"=w115:i32)  [unwired: 11 in]
              n38 = call "myRIO_BRig_RT_dataMTrig_Solenoid_Tdelay__R.vi"() -> ("output_Solenoid_Tdelay__R"=w114:i32)  [unwired: 11 in]
              n39 = local read "MTrig_Solenoid_Tcycle__L"() -> (w126:u16)
              n40 = local read "MTrig_Solenoid_Tcycle__R"() -> (w127:u16)
              n41 = local read "MTrig_Laser_Tcycle"() -> (w110:u16)
              n42 = call "myRIO_BRig_RT_dataMTrig_init.vi"() -> ("output_dataMTrig"=w120:u16[])  [unwired: 5 in]
              n43 = local write "RewCalib_Trig_R"(w113) -> ()
              n44 = local write "RewCalib_Trig_L"(w113) -> ()
              n45 = local read "Tcycle_Cue_min"() -> (w111:u16)
              n46 = Replace Array Subset(array=w120, new element #1=w126, index #1=w121, new element #2=w127, index #2=w122, new element #3=w111, index #3=w123, new element #4=w111, index #4=w124, new element #5=w110, index #5=w125, new element #6=w109, index #6=w117, new element #7=w109, index #7=w116, new element #8=w109, index #8=w115, new element #9=w109, index #9=w114) -> (w119:u16[])
            }
            frame "UploadSettings_pre" {
              # "When the Host sends settings,\nnot all files send at the same time.\n\nIf RT reads the settings faster\nthan the Host can send them,\nthen we will skip settings.\n\nSolution:\nWait 20 cycles"
              n47 = Increment(x=w136) -> (x+1=w135:u16)
              n48 = Greater?(x=w135, y=u16 20) -> (0:w133:bool)
              n49 = Select(t=myRIO_BRig_RT__Case_NonExp_stateList."UploadSettings_Read_dataExp", s=w133, f=w132) -> (s? t:f=w130:T1)
            }
            frame "UploadSettings_Read_dataExp" {
              # "grab dataExp and\nstore it in the\ngeneric data array"
              # "dataExp"
              n50 = call "myRIO_BRig_RT_dataExp_init_details.vi"() -> ("output_dataSize"=w143:i32, "output_dataName"=w146:string)  [unwired: 10 in]
              n51 = call "myRIO_BRig_RT_comm_webdav_uploadReceived_check.vi"("input_dataName"=w146) -> ("output_Iexist"=w145:bool, "output_dataPath"=w144:path)  [unwired: 9 in]
              n52 = case shown="True" w145 {
                tunnel: w144 -> [_ w155]
                tunnel: w143 -> [_ w154]
                tunnel: [_ w153] -> w142
                tunnel: w139 -> [w148 w152]
                tunnel: [w148 w149] -> w138
                frame False {
                }
                frame True {
                  n53 = call "myRIO_BRig_RT_comm_webdav_uploadReceived_read.vi"("input_dataSize"=w154, "input_filePath"=w155) -> ("output_Ivalid"=w153:bool, "output_data"=w151:i64[])  [unwired: 8 in]
                  n54 = To Unsigned Word Integer(number=w151) -> (unsigned 16bit integer=w150:u16[])
                  n55 = Select(t=w150, s=w153, f=w152) -> (s? t:f=w149:u16[])
                }
              }
              n56 = Select(t=myRIO_BRig_RT__Case_NonExp_stateList."UploadSettings_dataExp_1", s=w142, f=myRIO_BRig_RT__Case_NonExp_stateList."UploadSettings_Read_dataLC" ("t")) -> (s? t:f=w137:T1)
            }
            frame "UploadSettings_Read_dataLC" {
              # "grab dataLC and\nstore it in the\ngeneric data array"
              # "dataLC"
              n57 = call "myRIO_BRig_RT_dataLC_init_details.vi"() -> ("output_dataSize"=w162:i32, "output_dataName"=w165:string)  [unwired: 10 in]
              n58 = call "myRIO_BRig_RT_comm_webdav_uploadReceived_check.vi"("input_dataName"=w165) -> ("output_Iexist"=w164:bool, "output_dataPath"=w163:path)  [unwired: 9 in]
              n59 = case shown="True" w164 {
                tunnel: w163 -> [_ w174]
                tunnel: w162 -> [_ w173]
                tunnel: [_ w172] -> w161
                tunnel: w158 -> [w167 w171]
                tunnel: [w167 w168] -> w157
                frame False {
                }
                frame True {
                  n60 = call "myRIO_BRig_RT_comm_webdav_uploadReceived_read.vi"("input_dataSize"=w173, "input_filePath"=w174) -> ("output_Ivalid"=w172:bool, "output_data"=w170:i64[])  [unwired: 8 in]
                  n61 = To Unsigned Word Integer(number=w170) -> (unsigned 16bit integer=w169:u16[])
                  n62 = Select(t=w169, s=w172, f=w171) -> (s? t:f=w168:u16[])
                }
              }
              n63 = Select(t=myRIO_BRig_RT__Case_NonExp_stateList."UploadSettings_dataLC_1", s=w161, f=myRIO_BRig_RT__Case_NonExp_stateList."UploadSettings_Read_dataMTrig" ("t")) -> (s? t:f=w156:T1)
            }
            frame "UploadSettings_Read_dataMTrig" {
              # "grab dataMTrig and\nstore it in the\ngeneric data array"
              # "dataMTrig"
              n64 = call "myRIO_BRig_RT_dataMTrig_init_details.vi"() -> ("output_dataSize"=w181:i32, "output_dataName"=w184:string)  [unwired: 10 in]
              n65 = call "myRIO_BRig_RT_comm_webdav_uploadReceived_check.vi"("input_dataName"=w184) -> ("output_Iexist"=w183:bool, "output_dataPath"=w182:path)  [unwired: 9 in]
              n66 = case shown="True" w183 {
                tunnel: w182 -> [_ w193]
                tunnel: w181 -> [_ w192]
                tunnel: [_ w191] -> w180
                tunnel: w177 -> [w186 w190]
                tunnel: [w186 w187] -> w176
                frame False {
                }
                frame True {
                  n67 = call "myRIO_BRig_RT_comm_webdav_uploadReceived_read.vi"("input_dataSize"=w192, "input_filePath"=w193) -> ("output_Ivalid"=w191:bool, "output_data"=w189:i64[])  [unwired: 8 in]
                  n68 = To Unsigned Word Integer(number=w189) -> (unsigned 16bit integer=w188:u16[])
                  n69 = Select(t=w188, s=w191, f=w190) -> (s? t:f=w187:u16[])
                }
              }
              n70 = Select(t=myRIO_BRig_RT__Case_NonExp_stateList."UploadSettings_dataMTrig_1", s=w180, f=myRIO_BRig_RT__Case_NonExp_stateList."Idle" ("t")) -> (s? t:f=w175:T1)
            }
            frame "UploadSettings_dataExp_1" {
              w202 = 100.0 ("y")
              # "Freq"
              # "f_millisec2count"
              # "laser"
              # "Cue_max"
              # "Cue_min"
              # "CuePenalty"
              # "Timeout"
              # "Wrong"
              # "Selection"
              # "RewardPost"
              # "Reward_R"
              # "Reward_L"
              # "Tcycle"
              # "TPB_min_R"
              # "TPB_min_L"
              # "TPB_max_R"
              # "TPB_max_L"
              # "I_trialUntilReward"
              # "ENL_penalty"
              # "ENL_min"
              # "ENL_max"
              # "BUR_max"
              # "BUR_min"
              # "CueCycles"
              # "Audio_Freq_R"
              # "Audio_Freq_L"
              # "Audio_Amp_R"
              # "Audio_Amp_L"
              n71 = call "myRIO_BRig_RT_dataExp_laser_f_millisec2count.vi"() -> ("output_laser_f_millisec2count"=w216:i32)  [unwired: 11 in]
              n72 = call "myRIO_BRig_RT_dataExp_laser_Freq.vi"() -> ("output_laser_Freq"=w215:i32)  [unwired: 11 in]
              n73 = call "myRIO_BRig_RT_dataExp_CueCycles.vi"() -> ("output_CueCycles"=w262:i32)  [unwired: 11 in]
              n74 = call "myRIO_BRig_RT_dataExp_Audio_amp__R.vi"() -> ("output_Audio_amp__R"=w266:i32)  [unwired: 11 in]
              n75 = call "myRIO_BRig_RT_dataExp_Audio_amp__L.vi"() -> ("output_Audio_amp__L"=w268:i32)  [unwired: 11 in]
              n76 = call "myRIO_BRig_RT_dataExp_Tcycle_Reward__L.vi"() -> ("output_Tcycle_Reward__L"=w239:i32)  [unwired: 11 in]
              n77 = call "myRIO_BRig_RT_dataExp_Tcycle_Reward__R.vi"() -> ("output_Tcycle_Reward__R"=w238:i32)  [unwired: 11 in]
              n78 = call "myRIO_BRig_RT_dataExp_Tcycle_RewardPost.vi"() -> ("output_Tcycle_RewardPost"=w237:i32)  [unwired: 11 in]
              n79 = call "myRIO_BRig_RT_dataExp_BUR_min.vi"() -> ("output_BUR_min"=w259:i32)  [unwired: 11 in]
              n80 = call "myRIO_BRig_RT_dataExp_ENL_min.vi"() -> ("output_ENL_min"=w255:i32)  [unwired: 11 in]
              n81 = call "myRIO_BRig_RT_dataExp_TPB_max__L.vi"() -> ("output_TPB_max__L"=w247:i32)  [unwired: 11 in]
              n82 = call "myRIO_BRig_RT_dataExp_TPB_max__R.vi"() -> ("output_TPB_max__R"=w246:i32)  [unwired: 11 in]
              n83 = call "myRIO_BRig_RT_dataExp_ENL_penalty.vi"() -> ("output_ENL_penalty"=w254:i32)  [unwired: 11 in]
              n84 = call "myRIO_BRig_RT_dataExp_laser_Power_min.vi"() -> ("output_laser_Power_min"=w214:i32)  [unwired: 11 in]
              n85 = call "myRIO_BRig_RT_dataExp_laser_Tpeak.vi"() -> ("output_laser_Tpeak"=w213:i32)  [unwired: 11 in]
              n86 = call "myRIO_BRig_RT_dataExp_Audio_freq__L.vi"() -> ("output_Audio_freq__L"=w264:i32)  [unwired: 11 in]
              n87 = call "myRIO_BRig_RT_dataExp_Audio_freq__R.vi"() -> ("output_Audio_freq__R"=w263:i32)  [unwired: 11 in]
              n88 = call "myRIO_BRig_RT_dataExp_BUR_max.vi"() -> ("output_BUR_max"=w260:i32)  [unwired: 11 in]
              n89 = call "myRIO_BRig_RT_dataExp_ENL_max.vi"() -> ("output_ENL_max"=w256:i32)  [unwired: 11 in]
              n90 = call "myRIO_BRig_RT_dataExp_ItrialUntilReward.vi"() -> ("output_I_trialUntilReward"=w250:i32)  [unwired: 11 in]
              n91 = call "myRIO_BRig_RT_dataExp_Tcycle_Selection.vi"() -> ("output_Tcycle_Selection"=w236:i32)  [unwired: 11 in]
              n92 = call "myRIO_BRig_RT_dataExp_Tcycle_Wrong.vi"() -> ("output_Tcycle_Wrong"=w235:i32)  [unwired: 11 in]
              n93 = call "myRIO_BRig_RT_dataExp_Tcycle_Timeout.vi"() -> ("output_Tcycle_Timeout"=w234:i32)  [unwired: 11 in]
              n94 = call "myRIO_BRig_RT_dataExp_TPB_min__L.vi"() -> ("output_TPB_min__L"=w245:i32)  [unwired: 11 in]
              n95 = call "myRIO_BRig_RT_dataExp_TPB_min__R.vi"() -> ("output_TPB_min__R"=w244:i32)  [unwired: 11 in]
              n96 = call "myRIO_BRig_RT_dataExp_laser_Tshutter.vi"() -> ("output_laser_Tshutter"=w212:i32)  [unwired: 11 in]
              n97 = call "myRIO_BRig_RT_dataExp_laser_duration.vi"() -> ("output_laser_duration"=w211:i32)  [unwired: 11 in]
              n98 = call "myRIO_BRig_RT_dataExp_Tcycle_CuePenalty.vi"() -> ("output_Tcycle_CuePenalty"=w227:i32)  [unwired: 11 in]
              n99 = call "myRIO_BRig_RT_dataExp_Tcycle_Cue_min.vi"() -> ("output_Tcycle_Cue_min"=w226:i32)  [unwired: 11 in]
              n100 = call "myRIO_BRig_RT_dataExp_Tcycle_Cue_max.vi"() -> ("output_Tcycle_Cue_max"=w225:i32)  [unwired: 11 in]
              n101 = Index Array(array=w219, index #1=w268, index #2=w266, index #3=w264, index #4=w263, index #5=w262, index #6=w260, index #7=w259, index #8=w256, index #9=w255, index #10=w254, index #11=w250, index #12=w247, index #13=w246, index #14=w245, index #15=w244, index #16=w239, index #17=w238, index #18=w237, index #19=w236, index #20=w235, index #21=w234, index #22=w227, index #23=w226, index #24=w225, index #25=w216, index #26=w215, index #27=w214, index #28=w213, index #29=w212, index #30=w211) -> (element #1=w267:u16, element #2=w265:u16, element #3=w222:u16, element #4=w221:u16, element #5=w261:u16, element #6=w258:u16, element #7=w257:u16, element #8=w253:u16, element #9=w252:u16, element #10=w251:u16, element #11=w248:u16, element #12=w243:u16, element #13=w242:u16, element #14=w241:u16, element #15=w240:u16, element #16=w233:u16, element #17=w232:u16, element #18=w231:u16, element #19=w230:u16, element #20=w229:u16, element #21=w228:u16, element #22=w224:u16, element #23=w218:u16, element #24=w217:u16, element #25=w210:u16, element #26=w201:u16, element #27=w200:u16, element #28=w199:u16, element #29=w198:u16, element #30=w194:u16)
              n102 = To Double Precision Float(number=w210) -> (double precision float=w209:dbl)
              n103 = To Double Precision Float(number=w201) -> (double precision float=w207:dbl)
              n104 = To Double Precision Float(number=w200) -> (double precision float=w205:dbl)
              n105 = To Double Precision Float(number=w199) -> (double precision float=w204:dbl)
              n106 = To Double Precision Float(number=w198) -> (double precision float=w203:dbl)
              n107 = local write "Tcycle_Selection"(w230) -> ()
              n108 = local write "Tcycle_Wrong"(w229) -> ()
              n109 = local write "Tcycle_Timeout"(w228) -> ()
              n110 = local write "Audio_Amp__L"(w267) -> ()
              n111 = local write "Audio_Amp__R"(w265) -> ()
              n112 = Divide(x=w209, y=w202) -> (x/y=w208:dbl)
              n113 = Divide(x=w207, y=w202) -> (x/y=w206:dbl)
              n114 = Divide(x=w205, y=w202) -> (x/y=w197:dbl)
              n115 = Divide(x=w204, y=w202) -> (x/y=w196:dbl)
              n116 = Divide(x=w203, y=w202) -> (x/y=w195:dbl)
              n117 = local write "Tcycle_ENLPenalty"(w251) -> ()
              n118 = local write "Tcycle_ENL_max"(w253) -> ()
              n119 = local write "laser_duration"(w194) -> ()
              n120 = local write "TpB_Min_L"(w241) -> ()
              n121 = local write "TpB_Min_R"(w240) -> ()
              n122 = local write "laser_power_min"(w197) -> ()
              n123 = local write "f_millisec2count"(w208) -> ()
              n124 = local write "laser_Tshutter"(w195) -> ()
              n125 = local write "laser_Tpeak"(w196) -> ()
              n126 = local write "laser_Freq"(w206) -> ()
              n127 = local write "Tcycle_CuePenalty"(w224) -> ()
              n128 = local write "Tcycle_Cue_min"(w218) -> ()
              n129 = local write "Tcycle_Cue_max"(w217) -> ()
              n130 = To Unsigned Byte Integer(number=w222) -> (unsigned 8bit integer=w223:u8)
              n131 = To Unsigned Byte Integer(number=w221) -> (unsigned 8bit integer=w220:u8)
              n132 = Not Equal To 0?(x=w248) -> (x != 0?=w249:bool)
              n133 = local write "Tcycle_Reward_L"(w233) -> ()
              n134 = local write "Tcycle_Reward_R"(w232) -> ()
              n135 = local write "Tcycle_RewardPost"(w231) -> ()
              n136 = local write "CueCycles"(w261) -> ()
              n137 = local write "BUR_min"(w257) -> ()
              n138 = local write "BUR_max"(w258) -> ()
              n139 = local write "Tcycle_ENL_min"(w252) -> ()
              n140 = local write "TpB_Max_L"(w243) -> ()
              n141 = local write "TpB_Max_R"(w242) -> ()
              n142 = local write "TrialUntilReward"(w249) -> ()
              n143 = local write "Audio_Freq__L"(w223) -> ()
              n144 = local write "Audio_Freq__R"(w220) -> ()
            }
            frame "UploadSettings_dataLC_1" {
              # "Cue1_All_delayOpt"
              # "ENL1_All_delayOpt"
              # "Cue1_First_delayOpt"
              # "ENL1_First_delayOpt"
              # "ENL1 First"
              # "Cue1 All"
              # "Cue1 First"
              # "Count"
              # "Tdelay"
              # "Prob"
              # "OnOff"
              # "Block"
              # "ENL1 All"
              # "Count"
              # "Tdelay"
              # "Prob"
              # "OnOff"
              # "Block"
              # "Count"
              # "Tdelay"
              # "Prob"
              # "Block"
              # "OnOff"
              # "Count"
              # "Tdelay"
              # "Prob"
              # "OnOff"
              # "Block"
              n145 = call "myRIO_BRig_RT_dataLC_Cue1_First_Block.vi"() -> ("output_Cue1_First_Block"=w327:i32)  [unwired: 11 in]
              n146 = call "myRIO_BRig_RT_dataLC_Cue1_First_OnOff.vi"() -> ("output_Cue1_First_OnOff"=w325:i32)  [unwired: 11 in]
              n147 = call "myRIO_BRig_RT_dataLC_Cue1_First_Count.vi"() -> ("output_Cue1_First_Count"=w322:i32)  [unwired: 11 in]
              n148 = call "myRIO_BRig_RT_dataLC_Cue1_All_Block.vi"() -> ("output_Cue1_All_Block"=w309:i32)  [unwired: 11 in]
              n149 = call "myRIO_BRig_RT_dataLC_Cue1_All_OnOff.vi"() -> ("output_Cue1_All_OnOff"=w308:i32)  [unwired: 11 in]
              n150 = call "myRIO_BRig_RT_dataLC_Cue1_All_Count.vi"() -> ("output_Cue1_All_Count"=w319:i32)  [unwired: 11 in]
              n151 = call "myRIO_BRig_RT_dataLC_ENL1_First_Block.vi"() -> ("output_ENL1_First_Block"=w307:i32)  [unwired: 11 in]
              n152 = call "myRIO_BRig_RT_dataLC_ENL1_First_OnOff.vi"() -> ("output_ENL1_First_OnOff"=w318:i32)  [unwired: 11 in]
              n153 = call "myRIO_BRig_RT_dataLC_ENL1_First_Count.vi"() -> ("output_ENL1_First_Count"=w315:i32)  [unwired: 11 in]
              n154 = call "myRIO_BRig_RT_dataLC_ENL1_All_Block.vi"() -> ("output_ENL1_All_Block"=w314:i32)  [unwired: 11 in]
              n155 = call "myRIO_BRig_RT_dataLC_ENL1_All_OnOff.vi"() -> ("output_ENL1_All_OnOff"=w313:i32)  [unwired: 11 in]
              n156 = call "myRIO_BRig_RT_dataLC_ENL1_All_Count.vi"() -> ("output_ENL1_All_Count"=w310:i32)  [unwired: 11 in]
              n157 = call "myRIO_BRig_RT_dataLC_ENL1_First_delayOpt.vi"() -> ("output_ENL1_First_delayOpt"=w284:i32)  [unwired: 11 in]
              n158 = call "myRIO_BRig_RT_dataLC_Cue1_First_delayOpt.vi"() -> ("output_Cue1_First_delayOpt"=w283:i32)  [unwired: 11 in]
              n159 = call "myRIO_BRig_RT_dataLC_ENL1_All_delayOpt.vi"() -> ("output_ENL1_All_delayOpt"=w276:i32)  [unwired: 11 in]
              n160 = call "myRIO_BRig_RT_dataLC_Cue1_All_delayOpt.vi"() -> ("output_Cue1_All_delayOpt"=w275:i32)  [unwired: 11 in]
              n161 = call "myRIO_BRig_RT_dataLC_Cue1_First_Probability.vi"() -> ("output_Cue1_First_Probability"=w324:i32)  [unwired: 11 in]
              n162 = call "myRIO_BRig_RT_dataLC_Cue1_First_Tdelay.vi"() -> ("output_Cue1_First_Tdelay"=w323:i32)  [unwired: 11 in]
              n163 = call "myRIO_BRig_RT_dataLC_Cue1_All_Probability.vi"() -> ("output_Cue1_All_Probability"=w321:i32)  [unwired: 11 in]
              n164 = call "myRIO_BRig_RT_dataLC_Cue1_All_Tdelay.vi"() -> ("output_Cue1_All_Tdelay"=w320:i32)  [unwired: 11 in]
              n165 = call "myRIO_BRig_RT_dataLC_ENL1_First_Probability.vi"() -> ("output_ENL1_First_Probability"=w317:i32)  [unwired: 11 in]
              n166 = call "myRIO_BRig_RT_dataLC_ENL1_First_Tdelay.vi"() -> ("output_ENL1_First_Tdelay"=w316:i32)  [unwired: 11 in]
              n167 = call "myRIO_BRig_RT_dataLC_ENL1_All_Probability.vi"() -> ("output_ENL1_All_Probability"=w312:i32)  [unwired: 11 in]
              n168 = call "myRIO_BRig_RT_dataLC_ENL1_All_Tdelay.vi"() -> ("output_ENL1_All_Tdelay"=w311:i32)  [unwired: 11 in]
              n169 = Index Array(array=w285, index #1=w327, index #2=w325, index #3=w324, index #4=w323, index #5=w322, index #6=w309, index #7=w308, index #8=w321, index #9=w320, index #10=w319, index #11=w307, index #12=w318, index #13=w317, index #14=w316, index #15=w315, index #16=w314, index #17=w313, index #18=w312, index #19=w311, index #20=w310, index #21=w284, index #22=w283, index #23=w276, index #24=w275) -> (element #1=w326:u16, element #2=w305:u16, element #3=w304:u16, element #4=w303:u16, element #5=w302:u16, element #6=w298:u16, element #7=w297:u16, element #8=w296:u16, element #9=w295:u16, element #10=w294:u16, element #11=w293:u16, element #12=w292:u16, element #13=w291:u16, element #14=w290:u16, element #15=w277:u16, element #16=w289:u16, element #17=w288:u16, element #18=w287:u16, element #19=w286:u16, element #20=w278:u16, element #21=w281:u16, element #22=w279:u16, element #23=w272:u16, element #24=w271:u16)
              n170 = Not Equal To 0?(x=w272) -> (x != 0?=w274:bool)
              n171 = Not Equal To 0?(x=w271) -> (x != 0?=w273:bool)
              n172 = Not Equal To 0?(x=w281) -> (x != 0?=w282:bool)
              n173 = Not Equal To 0?(x=w279) -> (x != 0?=w280:bool)
              n174 = Not Equal To 0?(x=w305) -> (x != 0?=w306:bool)
              n175 = Not Equal To 0?(x=w297) -> (x != 0?=w301:bool)
              n176 = Not Equal To 0?(x=w292) -> (x != 0?=w300:bool)
              n177 = Not Equal To 0?(x=w288) -> (x != 0?=w299:bool)
              n178 = local write "LC_Cue1_First_Probability"(w304) -> ()
              n179 = local write "LC_ENL1_First_Probability"(w291) -> ()
              n180 = local write "LC_ENL1_First_delayOpt"(w282) -> ()
              n181 = local write "LC_Cue1_First_delayOpt"(w280) -> ()
              n182 = local write "LC_ENL1_All_delayOpt"(w274) -> ()
              n183 = local write "LC_Cue1_All_delayOpt"(w273) -> ()
              n184 = local write "LC_Cue1_All_Probability"(w296) -> ()
              n185 = local write "LC_Cue1_First_Tdelay"(w303) -> ()
              n186 = local write "LC_ENL1_All_Probability"(w287) -> ()
              n187 = local write "LC_Cue1_First_OnOff"(w306) -> ()
              n188 = local write "LC_Cue1_First_Count"(w302) -> ()
              n189 = local write "LC_Cue1_First_Block"(w326) -> ()
              n190 = local write "LC_ENL1_First_Tdelay"(w290) -> ()
              n191 = local write "LC_ENL1_First_OnOff"(w300) -> ()
              n192 = local write "LC_ENL1_First_Count"(w277) -> ()
              n193 = local write "LC_ENL1_First_Block"(w293) -> ()
              n194 = local write "LC_Cue1_All_Tdelay"(w295) -> ()
              n195 = local write "LC_Cue1_All_OnOff"(w301) -> ()
              n196 = local write "LC_Cue1_All_Count"(w294) -> ()
              n197 = local write "LC_Cue1_All_Block"(w298) -> ()
              n198 = local write "LC_ENL1_All_Tdelay"(w286) -> ()
              n199 = local write "LC_ENL1_All_OnOff"(w299) -> ()
              n200 = local write "LC_ENL1_All_Count"(w278) -> ()
              n201 = local write "LC_ENL1_All_Block"(w289) -> ()
            }
            frame "UploadSettings_dataLC_2" {
              # "Wrong"
              # "Reward"
              # "Trial"
              # "Tdelay"
              # "Prob"
              # "Block"
              # "OnOff"
              # "Trial"
              # "Tdelay"
              # "Prob"
              # "OnOff"
              # "Block"
              n202 = call "myRIO_BRig_RT_dataLC_Reward_Block.vi"() -> ("output_Reward_Block"=w352:i32)  [unwired: 11 in]
              n203 = call "myRIO_BRig_RT_dataLC_Reward_OnOff.vi"() -> ("output_Reward_OnOff"=w350:i32)  [unwired: 11 in]
              n204 = call "myRIO_BRig_RT_dataLC_Reward_Trial.vi"() -> ("output_Reward_Trial"=w347:i32)  [unwired: 11 in]
              n205 = call "myRIO_BRig_RT_dataLC_Wrong_Block.vi"() -> ("output_Wrong_Block"=w343:i32)  [unwired: 11 in]
              n206 = call "myRIO_BRig_RT_dataLC_Wrong_OnOff.vi"() -> ("output_Wrong_OnOff"=w342:i32)  [unwired: 11 in]
              n207 = call "myRIO_BRig_RT_dataLC_Wrong_Trial.vi"() -> ("output_Wrong_Trial"=w344:i32)  [unwired: 11 in]
              n208 = call "myRIO_BRig_RT_dataLC_Reward_Probability.vi"() -> ("output_Reward_Probability"=w349:i32)  [unwired: 11 in]
              n209 = call "myRIO_BRig_RT_dataLC_Reward_Tdelay.vi"() -> ("output_Reward_Tdelay"=w348:i32)  [unwired: 11 in]
              n210 = call "myRIO_BRig_RT_dataLC_Wrong_Probability.vi"() -> ("output_Wrong_Probability"=w346:i32)  [unwired: 11 in]
              n211 = call "myRIO_BRig_RT_dataLC_Wrong_Tdelay.vi"() -> ("output_Wrong_Tdelay"=w345:i32)  [unwired: 11 in]
              n212 = Index Array(array=w330, index #1=w352, index #2=w350, index #3=w349, index #4=w348, index #5=w347, index #6=w343, index #7=w342, index #8=w346, index #9=w345, index #10=w344) -> (element #1=w351:u16, element #2=w340:u16, element #3=w339:u16, element #4=w338:u16, element #5=w337:u16, element #6=w335:u16, element #7=w334:u16, element #8=w333:u16, element #9=w332:u16, element #10=w331:u16)
              n213 = Not Equal To 0?(x=w340) -> (x != 0?=w341:bool)
              n214 = Not Equal To 0?(x=w334) -> (x != 0?=w336:bool)
              n215 = local write "LC_Reward_Probability"(w339) -> ()
              n216 = local write "LC_Wrong_Probability"(w333) -> ()
              n217 = local write "LC_Reward_Tdelay"(w338) -> ()
              n218 = local write "LC_Reward_OnOff"(w341) -> ()
              n219 = local write "LC_Reward_Block"(w351) -> ()
              n220 = local write "LC_Reward_Trial"(w337) -> ()
              n221 = local write "LC_Wrong_Tdelay"(w332) -> ()
              n222 = local write "LC_Wrong_OnOff"(w336) -> ()
              n223 = local write "LC_Wrong_Block"(w335) -> ()
              n224 = local write "LC_Wrong_Trial"(w331) -> ()
            }
            frame "UploadSettings_dataMTrig_1" {
              # "Tdelay_R"
              # "Tdelay_L"
              # "Tcycle_R"
              # "Tcycle_L"
              # "RewCalib_nCycle_R"
              # "RewCalib_nCycle_L"
              # "Solenoid"
              # "Laser_Tcycle"
              n225 = call "myRIO_BRig_RT_dataMTrig_Laser_Tcycle.vi"() -> ("output_Laser_Tcycle"=w362:i32)  [unwired: 11 in]
              n226 = call "myRIO_BRig_RT_dataMTrig_Solenoid_RewCalib_nCycle__L.vi"() -> ("output_Solenoid_RewCalib_nCycle__L"=w361:i32)  [unwired: 11 in]
              n227 = call "myRIO_BRig_RT_dataMTrig_Solenoid_RewCalib_nCycle__R.vi"() -> ("output_Solenoid_RewCalib_nCycle__R"=w360:i32)  [unwired: 11 in]
              n228 = call "myRIO_BRig_RT_dataMTrig_Solenoid_Tdelay__L.vi"() -> ("output_Solenoid_Tdelay__L"=w357:i32)  [unwired: 11 in]
              n229 = call "myRIO_BRig_RT_dataMTrig_Solenoid_Tdelay__R.vi"() -> ("output_Solenoid_Tdelay__R"=w356:i32)  [unwired: 11 in]
              n230 = call "myRIO_BRig_RT_dataMTrig_Solenoid_Tcycle__L.vi"() -> ("output_Solenoid_Tcycle__L"=w359:i32)  [unwired: 11 in]
              n231 = call "myRIO_BRig_RT_dataMTrig_Solenoid_Tcycle__R.vi"() -> ("output_Solenoid_Tcycle__R"=w358:i32)  [unwired: 11 in]
              n232 = Index Array(array=w355, index #1=w362, index #2=w361, index #3=w360, index #4=w359, index #5=w358, index #6=w357, index #7=w356) -> (element #1=w369:u16, element #2=w368:u16, element #3=w367:u16, element #4=w366:u16, element #5=w365:u16, element #6=w364:u16, element #7=w363:u16)
              n233 = Replace Array Subset(array=w371, new element #1=w369, index #1=w362, new element #2=w368, index #2=w361, new element #3=w367, index #3=w360, new element #4=w366, index #4=w359, new element #5=w365, index #5=w358, new element #6=w364, index #6=w357, new element #7=w363, index #7=w356) -> (w370:u16[])
              n234 = local write "MTrig_Solenoid_Tcycle__L"(w366) -> ()
              n235 = local write "MTrig_Solenoid_Tcycle__R"(w365) -> ()
              n236 = local write "MTrig_Laser_Tcycle"(w369) -> ()
            }
            frame "Idle" {
              # "To ensure timing, we split the\nidle state into 4 phases"
              # "Laser_Tcycle"
              # "Audio_Tcycle_R"
              # "Audio_Tcycle_L"
              n237 = local read "laser_power_min"() -> (w374:dbl)
              n238 = local read "f_millisec2count"() -> (w382:dbl)
              n239 = local read "Audio_Amp__R"() -> (w376:u16)
              n240 = local read "Audio_Amp__L"() -> (w378:u16)
              n241 = local read "Audio_Freq__R"() -> (w375:u8)
              n242 = local read "Audio_Freq__L"() -> (w377:u8)
              n243 = local read "MTrig_Audio_trig__L"() -> (w390:bool)
              n244 = local read "MTrig_Audio_trig__R"() -> (w392:bool)
              n245 = Select(t=myRIO_BRig_RT__Case_NonExp_stateList."SendData" ("Enum"), s="SendData", f=myRIO_BRig_RT__Case_NonExp_stateList."Idle_2" ("Enum")) -> (s? t:f=w385:T1)
              n246 = call "myRIO_Brig_RT__covert_Voltage_to_FPGAvalue.vi"("input_voltage"=w374) -> ("output_PortC"=w373:i16)  [unwired: 9 in, 1 out]
              n247 = local read "MTrig_Laser_trig"() -> (w391:bool)
              n248 = To Unsigned Word Integer(number=w382) -> (unsigned 16bit integer=w381:u16)
              n249 = call "myRIO_BRig_RT_dataMTrig_Audio_Tcycle__L.vi"() -> ("output_Audio_Tcycle__L"=w401:i32)  [unwired: 11 in]
              n250 = call "myRIO_BRig_RT_dataMTrig_Audio_Tcycle__R.vi"() -> ("output_Audio_Tcycle__R"=w400:i32)  [unwired: 11 in]
              n251 = call "myRIO_BRig_RT_dataMTrig_Laser_Tcycle.vi"() -> ("output_Laser_Tcycle"=w399:i32)  [unwired: 11 in]
              n252 = local read "MTrig_Laser_Tcycle"() -> (w383:u16)
              n253 = xnode "Read/Write Control"("FPGA VI Reference In"=w380, "error in"=w379, "k1__counter_per_ms"=w381, "audioAmp_L"=w378, "audioFreq_L_kHz"=w377, "audioAmp_R"=w376, "audioFreq_R_kHz"=w375, "AnaOut_0"=w373) -> ()  [unwired: 2 out]
              n254 = Select(t=myRIO_BRig_RT__Case_NonExp_stateList."TestConnection" ("Enum"), s="TestConnection", f=w385) -> (s? t:f=w394:T1)
              n255 = local read "Tcycle_Cue_min"() -> (w384:u16)
              n256 = Compound Arithmetic op=OR(w390, w392, w391) -> (w393:bool)
              n257 = case shown="True" w393 {
                frame False {
                }
                frame True {
                  w402 = FALSE
                  n258 = local write "MTrig_Audio_trig__L"(w402) -> ()
                  n259 = local write "MTrig_Audio_trig__R"(w402) -> ()
                  n260 = local write "MTrig_Laser_trig"(w402) -> ()
                }
              }
              n261 = Replace Array Subset(array=w397, new element #1=w384, index #1=w401, new element #2=w384, index #2=w400, new element #3=w383, index #3=w399) -> (w398:u16[])
            }
            frame "Idle_2" {
              w404 = u16 0 ("t")
              # "To ensure timing, we split the\nidle state into 4 phases"
              # "Ncycles"
              # "Ncycles"
              # "RewCalib"
              # "RewCalib"
              # "Solenoid R"
              # "Solenoid L"
              n262 = call "myRIO_BRig_RT_dataMTrig_Solenoid_RewCalib_OnOff__L.vi"() -> ("output_Solenoid_RewCalib_OnOff__L"=w435:i32)  [unwired: 11 in]
              n263 = call "myRIO_BRig_RT_dataMTrig_Solenoid_N__L.vi"() -> ("output_Solenoid_N__L"=w423:i32)  [unwired: 11 in]
              n264 = call "myRIO_BRig_RT_dataMTrig_Solenoid_RewCalib_OnOff__R.vi"() -> ("output_Solenoid_RewCalib_OnOff__R"=w420:i32)  [unwired: 11 in]
              n265 = call "myRIO_BRig_RT_dataMTrig_Solenoid_N__R.vi"() -> ("output_Solenoid_N__R"=w419:i32)  [unwired: 11 in]
              n266 = Index Array(array=w426, index #1=w435, index #2=w423, index #3=w420, index #4=w419) -> (element #1=w422:u16, element #2=w417:u16, element #3=w418:u16, element #4=w416:u16)
              n267 = local read "RewCalib_Trig_L"() -> (w415:bool)
              n268 = local read "RewCalib_Trig_R"() -> (w414:bool)
              n269 = Equal To 0?(x=w417) -> (x = 0?=w425:bool)
              n270 = Equal To 0?(x=w416) -> (x = 0?=w424:bool)
              n271 = Not Equal To 0?(x=w418) -> (x != 0?=w436:bool)
              n272 = Not Equal To 0?(x=w422) -> (x != 0?=w437:bool)
              n273 = And(x=w425, y=w424) -> (x .and. y?=w429:bool)
              n274 = Or(x=w415, y=w414) -> (x .or. y?=w430:bool)
              n275 = Not Exclusive Or(1:w437, 2:w415) -> (0:w432:bool)
              n276 = Not Exclusive Or(1:w436, 2:w414) -> (0:w434:bool)
              n277 = And(x=w430, y=w429) -> (x .and. y?=w412:bool)
              n278 = Not(x=w432) -> (.not. x?=w431:bool)
              n279 = Not(x=w434) -> (.not. x?=w433:bool)
              n280 = Or(x=w431, y=w433) -> (x .or. y?=w413:bool)
              n281 = Or(x=w412, y=w413) -> (x .or. y?=w428:bool)
              n282 = local read "count_warmup_R"() -> (w403:u16)
              n283 = local read "count_warmup_L"() -> (w408:u16)
              n284 = Select(t=myRIO_BRig_RT__Case_NonExp_stateList."RewardCalibration_pre" ("Enum"), s=w428, f=myRIO_BRig_RT__Case_NonExp_stateList."Idle_3" ("Enum")) -> (s? t:f=w411:T1)
              n285 = Select(t=w404, s="count_warmup_L_reset", f=w408) -> (s? t:f=→"count_warmup_L":u16)
              n286 = Select(t=w404, s="count_warmup_R_reset", f=w403) -> (s? t:f=→"count_warmup_R":u16)
            }
            frame "Idle_3" {
              w460 = u8 0 ("f")
              # "To ensure timing, we split the\nidle state into 4 phases"
              n287 = local read "MTrig_Solenoid_trig__L"() -> (w451:bool)
              n288 = local read "MTrig_Solenoid_trig__R"() -> (w461:bool)
              n289 = local read "warmupType"() -> (w443:u8)
              n290 = local read "warmup"() -> (w453:bool)
              n291 = Not Equal To 0?(x=w443) -> (x != 0?=w442:bool)
              n292 = Not(x=w442) -> (.not. x?=w454:bool)
              n293 = Select(t=u8 1, s=w451, f=w460) -> (s? t:f=w459:u8)
              n294 = Select(t=u8 2, s=w461, f=w460) -> (s? t:f=w458:u8)
              n295 = And(x=w453, y=w454) -> (x .and. y?=w452:bool)
              n296 = And(x=w453, y=w442) -> (x .and. y?=w447:bool)
              n297 = Add(x=w459, y=w458) -> (x+y=w457:u8)
              n298 = case shown="3" w457 {
                tunnel: w456 -> [w464 w468 w486 w504]
                tunnel: [w464 w467 w485 w503] -> w455
                tunnel: w452 -> [_ w466 w484 w502]
                tunnel: [_ TRUE TRUE TRUE] -> w449
                frame 0, Default {
                }
                frame 1 {
                  n299 = case shown="True" w466 {
                    tunnel: w468 -> [w477 w482]
                    tunnel: [w476 w481] -> w467
                    frame True {
                      # "Audio_L"
                      # "Solenoid_L"
                      n300 = call "myRIO_BRig_RT_dataMTrig_Solenoid_N__L.vi"() -> ("output_Solenoid_N__L"=w473:i32)  [unwired: 11 in]
                      n301 = call "myRIO_BRig_RT_dataMTrig_Audio_N__L.vi"() -> ("output_Audio_N__L"=w471:i32)  [unwired: 11 in]
                      n302 = Index Array(array=w477, index #1=w473, index #2=w471) -> (element #1=w475:u16, element #2=w474:u16)
                      n303 = Increment(x=w475) -> (x+1=w472:u16)
                      n304 = Increment(x=w474) -> (x+1=w470:u16)
                      n305 = Replace Array Subset(array=w477, new element #1=w472, index #1=w473, new element #2=w470, index #2=w471) -> (w476:u16[])
                    }
                    frame False {
                      # "Solenoid_L"
                      n306 = call "myRIO_BRig_RT_dataMTrig_Solenoid_N__L.vi"() -> ("output_Solenoid_N__L"=w479:i32)  [unwired: 11 in]
                      n307 = Index Array(array=w482, index=w479) -> (element=w480:u16)
                      n308 = Increment(x=w480) -> (x+1=w478:u16)
                      n309 = Replace Array Subset(array=w482, new element=w478, index=w479) -> (w481:u16[])
                    }
                  }
                  n310 = local write "MTrig_Solenoid_trig__L"(FALSE) -> ()
                }
                frame 2 {
                  n311 = case shown="True" w484 {
                    tunnel: w486 -> [w495 w500]
                    tunnel: [w494 w499] -> w485
                    frame True {
                      # "Audio_R"
                      # "Solenoid_R"
                      n312 = call "myRIO_BRig_RT_dataMTrig_Solenoid_N__R.vi"() -> ("output_Solenoid_N__R"=w491:i32)  [unwired: 11 in]
                      n313 = call "myRIO_BRig_RT_dataMTrig_Audio_N__R.vi"() -> ("output_Audio_N__R"=w490:i32)  [unwired: 11 in]
                      n314 = Index Array(array=w495, index #1=w491, index #2=w490) -> (element #1=w493:u16, element #2=w492:u16)
                      n315 = Increment(x=w492) -> (x+1=w488:u16)
                      n316 = Increment(x=w493) -> (x+1=w489:u16)
                      n317 = Replace Array Subset(array=w495, new element #1=w489, index #1=w491, new element #2=w488, index #2=w490) -> (w494:u16[])
                    }
                    frame False {
                      # "Solenoid_R"
                      n318 = call "myRIO_BRig_RT_dataMTrig_Solenoid_N__R.vi"() -> ("output_Solenoid_N__R"=w496:i32)  [unwired: 11 in]
                      n319 = Index Array(array=w500, index=w496) -> (element=w498:u16)
                      n320 = Increment(x=w498) -> (x+1=w497:u16)
                      n321 = Replace Array Subset(array=w500, new element=w497, index=w496) -> (w499:u16[])
                    }
                  }
                  n322 = local write "MTrig_Solenoid_trig__R"(FALSE) -> ()
                }
                frame 3 {
                  w505 = FALSE
                  n323 = case shown="True" w502 {
                    tunnel: w504 -> [w519 w527]
                    tunnel: [w518 w526] -> w503
                    frame True {
                      # "Audio_R"
                      # "Solenoid_R"
                      # "Audio_L"
                      # "Solenoid_L"
                      n324 = call "myRIO_BRig_RT_dataMTrig_Solenoid_N__L.vi"() -> ("output_Solenoid_N__L"=w513:i32)  [unwired: 11 in]
                      n325 = call "myRIO_BRig_RT_dataMTrig_Audio_N__L.vi"() -> ("output_Audio_N__L"=w511:i32)  [unwired: 11 in]
                      n326 = call "myRIO_BRig_RT_dataMTrig_Solenoid_N__R.vi"() -> ("output_Solenoid_N__R"=w509:i32)  [unwired: 11 in]
                      n327 = call "myRIO_BRig_RT_dataMTrig_Audio_N__R.vi"() -> ("output_Audio_N__R"=w508:i32)  [unwired: 11 in]
                      n328 = Index Array(array=w519, index #1=w513, index #2=w511, index #3=w509, index #4=w508) -> (element #1=w517:u16, element #2=w516:u16, element #3=w515:u16, element #4=w514:u16)
                      n329 = Increment(x=w514) -> (x+1=w506:u16)
                      n330 = Increment(x=w517) -> (x+1=w512:u16)
                      n331 = Increment(x=w516) -> (x+1=w510:u16)
                      n332 = Increment(x=w515) -> (x+1=w507:u16)
                      n333 = Replace Array Subset(array=w519, new element #1=w512, index #1=w513, new element #2=w510, index #2=w511, new element #3=w507, index #3=w509, new element #4=w506, index #4=w508) -> (w518:u16[])
                    }
                    frame False {
                      # "Solenoid_R"
                      # "Solenoid_L"
                      n334 = call "myRIO_BRig_RT_dataMTrig_Solenoid_N__L.vi"() -> ("output_Solenoid_N__L"=w523:i32)  [unwired: 11 in]
                      n335 = call "myRIO_BRig_RT_dataMTrig_Solenoid_N__R.vi"() -> ("output_Solenoid_N__R"=w520:i32)  [unwired: 11 in]
                      n336 = Index Array(array=w527, index #1=w523, index #2=w520) -> (element #1=w525:u16, element #2=w524:u16)
                      n337 = Increment(x=w525) -> (x+1=w522:u16)
                      n338 = Increment(x=w524) -> (x+1=w521:u16)
                      n339 = Replace Array Subset(array=w527, new element #1=w522, index #1=w523, new element #2=w521, index #2=w520) -> (w526:u16[])
                    }
                  }
                  n340 = local write "MTrig_Solenoid_trig__L"(w505) -> ()
                  n341 = local write "MTrig_Solenoid_trig__R"(w505) -> ()
                }
              }
              n342 = local read "get_countPerMS"() -> (w441:bool)
              n343 = Select(t=myRIO_BRig_RT__Case_NonExp_stateList."Get_FPGA_count_per_ms" ("Enum"), s=w441, f=myRIO_BRig_RT__Case_NonExp_stateList."Idle_4" ("Enum")) -> (s? t:f=w439:T1)
              n344 = Select(t=myRIO_BRig_RT__Case_NonExp_stateList."Cue_pre", s=w447, f=myRIO_BRig_RT__Case_NonExp_stateList."DispenseWater_pre" ("Enum")) -> (s? t:f=w445:T1)
              n345 = Select(t=w445, s=w449, f=w439) -> (s? t:f=w450:T1)
            }
            frame "Idle_4" {
              # "use dataMTrig as it is one of the last to transfer"
              # "To ensure timing, we split the\nidle state into 4 phases"
              n346 = call "myRIO_BRig_RT_comm_webdav_uploadReceived_check_v2,0.vi"("input_dataName"="dataMTrig") -> ("output_Iexist"=w533:bool)  [unwired: 9 in, 1 out]
              n347 = Select(t=myRIO_BRig_RT__Case_NonExp_stateList."UploadSettings_pre" ("Enum"), s=w533, f=myRIO_BRig_RT__Case_NonExp_stateList."Idle") -> (s? t:f=w531:T1)
            }
            frame "Cue_pre" {
              w543 = u16 1 ("t")
              w542 = u16 0 ("new element/subarray")
              w539 = u16 0 ("new element/subarray")
              # "Ncycle"
              # "count"
              # "Audio_R"
              # "Solenoid_R"
              # "Solenoid_L"
              # "Ncycle"
              # "count"
              # "Audio_L"
              n348 = call "myRIO_BRig_RT_dataMTrig_Solenoid_N__L.vi"() -> ("output_Solenoid_N__L"=w552:i32)  [unwired: 11 in]
              n349 = call "myRIO_BRig_RT_dataMTrig_Solenoid_N__R.vi"() -> ("output_Solenoid_N__R"=w551:i32)  [unwired: 11 in]
              n350 = Index Array(array=w548, index #1=w552, index #2=w551) -> (element #1=w550:u16, element #2=w549:u16)
              n351 = Not Equal To 0?(x=w549) -> (x != 0?=w535:bool)
              n352 = Not Equal To 0?(x=w550) -> (x != 0?=w536:bool)
              n353 = Select(t=w543, s=w536, f=w542) -> (s? t:f=w544:u16)
              n354 = Select(t=w543, s=w535, f=w542) -> (s? t:f=w538:u16)
              n355 = call "myRIO_BRig_RT_dataMTrig_Audio_c__L.vi"() -> ("output_Audio_c__L"=w546:i32)  [unwired: 11 in]
              n356 = call "myRIO_BRig_RT_dataMTrig_Audio_N__L.vi"() -> ("output_Audio_N__L"=w545:i32)  [unwired: 11 in]
              n357 = call "myRIO_BRig_RT_dataMTrig_Audio_c__R.vi"() -> ("output_Audio_c__R"=w541:i32)  [unwired: 11 in]
              n358 = call "myRIO_BRig_RT_dataMTrig_Audio_N__R.vi"() -> ("output_Audio_N__R"=w540:i32)  [unwired: 11 in]
              n359 = Replace Array Subset(array=w548, new element #1=w539, index #1=w546, new element #2=w544, index #2=w545, new element #3=w539, index #3=w541, new element #4=w538, index #4=w540) -> (w547:u16[])
            }
            frame "Cue" {
              # "lick did not occur or warmupType==1"
              # "lick occurred?"
              # "Ncycle"
              # "Audio_R"
              # "Ncycle"
              # "Audio_L"
              n360 = local read "warmupType"() -> (w562:u8)
              n361 = Greater?(x=w568, y=w567) -> (0:w571:bool)
              n362 = Greater?(x=w570, y=w569) -> (0:w566:bool)
              n363 = Or(x=w566, y=w571) -> (x .or. y?=w560:bool)
              n364 = Equal?(x=w562, y=u8 1) -> (x = y?=w556:bool)
              n365 = Not(x=w560) -> (.not. x?=w559:bool)
              n366 = call "myRIO_BRig_RT_dataMTrig_Audio_N__L.vi"() -> ("output_Audio_N__L"=w574:i32)  [unwired: 11 in]
              n367 = call "myRIO_BRig_RT_dataMTrig_Audio_N__R.vi"() -> ("output_Audio_N__R"=w573:i32)  [unwired: 11 in]
              n368 = Or(x=w559, y=w556) -> (x .or. y?=w557:bool)
              n369 = case shown="True" w557 {
                tunnel: w574 -> [w580 w598]
                tunnel: w573 -> [w579 w597]
                tunnel: w565 -> [w582 w592]
                tunnel: [w581 w592] -> w564
                tunnel: w563 -> [_ w590]
                tunnel: [myRIO_BRig_RT__Case_NonExp_stateList."Idle" ("t") w589] -> w558
                tunnel: w556 -> [_ w588]
                tunnel: w555 -> [_ w584]
                tunnel: w554 -> [_ w583]
                frame False {
                  w575 = u16 0 ("new element/subarray")
                  # "lick occurred and warmupType==2"
                  n370 = call "myRIO_BRig_RT_dataMTrig_Solenoid_N__R.vi"() -> ("output_Solenoid_N__R"=w576:i32)  [unwired: 11 in]
                  n371 = call "myRIO_BRig_RT_dataMTrig_Solenoid_N__L.vi"() -> ("output_Solenoid_N__L"=w577:i32)  [unwired: 11 in]
                  n372 = Replace Array Subset(array=w582, new element #1=w575, index #1=w580, new element #2=w575, index #2=w579, new element #3=w575, index #3=w577, new element #4=w575, index #4=w576) -> (w581:u16[])
                }
                frame True {
                  n373 = Not(x=w588) -> (.not. x?=w587:bool)
                  n374 = Index Array(array=w592, index #1=w598, index #2=w597) -> (element #1=w596:u16, element #2=w595:u16)
                  n375 = Equal To 0?(x=w596) -> (x = 0?=w594:bool)
                  n376 = Equal To 0?(x=w595) -> (x = 0?=w593:bool)
                  n377 = And(x=w594, y=w593) -> (x .and. y?=w586:bool)
                  n378 = And(x=w586, y=w587) -> (x .and. y?=w585:bool)
                  n379 = case shown="True" w585 {
                    tunnel: w584 -> [_ w606]
                    tunnel: w583 -> [_ w601]
                    frame False {
                    }
                    frame True {
                      n380 = local read "count_warmup_R"() -> (w599:u16)
                      n381 = local read "count_warmup_L"() -> (w604:u16)
                      n382 = Increment(x=w599) -> (x+1=w602:u16)
                      n383 = Increment(x=w604) -> (x+1=w605:u16)
                      n384 = Select(t=w602, s=w601, f=w599) -> (s? t:f=w600:u16)
                      n385 = Select(t=w605, s=w606, f=w604) -> (s? t:f=w603:u16)
                      n386 = local write "count_warmup_R"(w600) -> ()
                      n387 = local write "count_warmup_L"(w603) -> ()
                    }
                  }
                  n388 = Select(t=myRIO_BRig_RT__Case_NonExp_stateList."DispenseWater_pre", s=w586, f=w590) -> (s? t:f=w589:T1)
                }
              }
            }
            frame "RewardCalibration_pre" {
              (unwired) FALSE
              w608 = FALSE
              w619 = u8 0
              w635 = u8 0
              # "Are we starting a RewardCalibration?\nOr are we stopping a RewardCalibration?\nOr is a RewardCalibration over?"
              # "RewCalib\nOnOff"
              # "N"
              # "Solenoid R"
              # "RewCalib\nOnOff"
              # "N"
              # "Solenoid L"
              n389 = local read "RewCalib_Trig_L"() -> (w642:bool)
              n390 = local read "RewCalib_Trig_R"() -> (w611:bool)
              n391 = call "myRIO_BRig_RT_dataMTrig_Solenoid_N__R.vi"() -> ("output_Solenoid_N__R"=w613:i32)  [unwired: 11 in]
              n392 = call "myRIO_BRig_RT_dataMTrig_Solenoid_RewCalib_OnOff__R.vi"() -> ("output_Solenoid_RewCalib_OnOff__R"=w610:i32)  [unwired: 11 in]
              n393 = call "myRIO_BRig_RT_dataMTrig_Solenoid_N__L.vi"() -> ("output_Solenoid_N__L"=w628:i32)  [unwired: 11 in]
              n394 = call "myRIO_BRig_RT_dataMTrig_Solenoid_RewCalib_OnOff__L.vi"() -> ("output_Solenoid_RewCalib_OnOff__L"=w629:i32)  [unwired: 11 in]
              n395 = Index Array(array=w612, index #1=w613, index #2=w610) -> (element #1=w623:u16, element #2=w618:u16)
              n396 = Index Array(array=w612, index #1=w628, index #2=w629) -> (element #1=w639:u16, element #2=w634:u16)
              n397 = Equal To 0?(x=w623) -> (x = 0?=w624:bool)
              n398 = Not Equal To 0?(x=w618) -> (x != 0?=w621:bool)
              n399 = Equal To 0?(x=w639) -> (x = 0?=w640:bool)
              n400 = Not Equal To 0?(x=w634) -> (x != 0?=w637:bool)
              n401 = local write "MTrig_Solenoid_trig__L"(w608) -> ()
              n402 = local write "MTrig_Solenoid_trig__R"(w608) -> ()
              n403 = Select(t=u8 1, s=w611, f=w619) -> (s? t:f=w615:u8)
              n404 = Select(t=u8 1, s=w642, f=w635) -> (s? t:f=w631:u8)
              n405 = Select(t=u8 2, s=w624, f=w619) -> (s? t:f=w616:u8)
              n406 = Select(t=u8 4, s=w621, f=w619) -> (s? t:f=w617:u8)
              n407 = Select(t=u8 2, s=w640, f=w635) -> (s? t:f=w632:u8)
              n408 = Select(t=u8 4, s=w637, f=w635) -> (s? t:f=w633:u8)
              n409 = Compound Arithmetic op=ADD(w615, w616, w617) -> (w614:u8)
              n410 = Compound Arithmetic op=ADD(w631, w632, w633) -> (w630:u8)
              n411 = case shown="7" w630 {
                tunnel: w612 -> [w672 w677 w679 w684 w689 w691 w694 w699]
                tunnel: [w672 w678 w679 w685 w690 w691 w695 w700] -> w627
                tunnel: w629 -> [_ w675 _ w682 w687 _ w693 w698]
                tunnel: w628 -> [_ w676 _ w683 w688 _ _ _]
                frame 0, Default {
                }
                frame 1 {
                  n412 = Replace Array Subset(array=w677, new element #1=u16 100 ("new element/subarray"), index #1=w676, new element #2=u16 1 ("new element/subarray"), index #2=w675) -> (w678:u16[])
                }
                frame 2 {
                }
                frame 3 {
                  n413 = Replace Array Subset(array=w684, new element #1=u16 100 ("new element/subarray"), index #1=w683, new element #2=u16 1 ("new element/subarray"), index #2=w682) -> (w685:u16[])
                }
                frame 4 {
                  w686 = u16 0 ("new element/subarray")
                  n414 = Replace Array Subset(array=w689, new element #1=w686, index #1=w688, new element #2=w686, index #2=w687) -> (w690:u16[])
                }
                frame 5 {
                }
                frame 6 {
                  n415 = Replace Array Subset(array=w694, new element=u16 0 ("new element/subarray"), index=w693) -> (w695:u16[])
                }
                frame 7 {
                  n416 = local write "RewCalib_Trig_L"(FALSE ("RewCalib_Trig_L")) -> ()
                  n417 = Replace Array Subset(array=w699, new element=u16 0 ("new element/subarray"), index=w698) -> (w700:u16[])
                }
              }
              n418 = case shown="7" w614 {
                tunnel: w627 -> [w643 w648 w650 w655 w660 w662 w665 w670]
                tunnel: [w643 w649 w650 w656 w661 w662 w666 w671] -> w626
                tunnel: w610 -> [_ w646 _ w653 w658 _ w664 w669]
                tunnel: w613 -> [_ w647 _ w654 w659 _ _ _]
                frame 0, Default {
                }
                frame 1 {
                  n419 = Replace Array Subset(array=w648, new element #1=u16 100 ("new element/subarray"), index #1=w647, new element #2=u16 1 ("new element/subarray"), index #2=w646) -> (w649:u16[])
                }
                frame 2 {
                }
                frame 3 {
                  n420 = Replace Array Subset(array=w655, new element #1=u16 100 ("new element/subarray"), index #1=w654, new element #2=u16 1 ("new element/subarray"), index #2=w653) -> (w656:u16[])
                }
                frame 4 {
                  w657 = u16 0 ("new element/subarray")
                  n421 = Replace Array Subset(array=w660, new element #1=w657, index #1=w659, new element #2=w657, index #2=w658) -> (w661:u16[])
                }
                frame 5 {
                }
                frame 6 {
                  n422 = Replace Array Subset(array=w665, new element=u16 0 ("new element/subarray"), index=w664) -> (w666:u16[])
                }
                frame 7 {
                  n423 = local write "RewCalib_Trig_R"(FALSE ("RewCalib_Trig_L")) -> ()
                  n424 = Replace Array Subset(array=w670, new element=u16 0 ("new element/subarray"), index=w669) -> (w671:u16[])
                }
              }
            }
            frame "DispenseWater_pre" {
              w707 = u16 0 ("t")
              w750 = u16 0 ("new element/subarray")
              # "just trust me on this one"
              # "RewCalib\nOnOff"
              # "RewCalib\nOnOff"
              # "nCycle"
              # "Solenoid__R"
              # "Tdelay"
              # "delay"
              # "nCycle"
              # "Solenoid__L"
              # "Tdelay"
              # "delay"
              # "Solenoid__R"
              # "count"
              # "Solenoid_Tcycle_R"
              # "Solenoid_Tcycle_L"
              # "Solenoid__L"
              # "count"
              n425 = call "myRIO_BRig_RT_dataMTrig_Solenoid_RewCalib_OnOff__L.vi"() -> ("output_Solenoid_RewCalib_OnOff__L"=w714:i32)  [unwired: 11 in]
              n426 = call "myRIO_BRig_RT_dataMTrig_Solenoid_N__L.vi"() -> ("output_Solenoid_N__L"=w705:i32)  [unwired: 11 in]
              n427 = call "myRIO_BRig_RT_dataMTrig_Solenoid_delay__L.vi"() -> ("output_Solenoid_delay__L"=w748:i32)  [unwired: 11 in]
              n428 = call "myRIO_BRig_RT_dataMTrig_Solenoid_Tdelay__L.vi"() -> ("output_Solenoid_Tdelay__L"=w747:i32)  [unwired: 11 in]
              n429 = call "myRIO_BRig_RT_dataMTrig_Solenoid_N__R.vi"() -> ("output_Solenoid_N__R"=w703:i32)  [unwired: 11 in]
              n430 = call "myRIO_BRig_RT_dataMTrig_Solenoid_delay__R.vi"() -> ("output_Solenoid_delay__R"=w737:i32)  [unwired: 11 in]
              n431 = call "myRIO_BRig_RT_dataMTrig_Solenoid_Tdelay__R.vi"() -> ("output_Solenoid_Tdelay__R"=w736:i32)  [unwired: 11 in]
              n432 = call "myRIO_BRig_RT_dataMTrig_Solenoid_RewCalib_OnOff__R.vi"() -> ("output_Solenoid_RewCalib_OnOff__R"=w710:i32)  [unwired: 11 in]
              n433 = Index Array(array=w749, index #1=w705, index #2=w748, index #3=w747, index #4=w703, index #5=w737, index #6=w736, index #7=w714, index #8=w710) -> (element #1=w706:u16, element #2=w746:u16, element #3=w741:u16, element #4=w709:u16, element #5=w731:u16, element #6=w730:u16, element #7=w715:u16, element #8=w712:u16)
              n434 = Equal To 0?(x=w746) -> (x = 0?=w745:bool)
              n435 = Equal To 0?(x=w731) -> (x = 0?=w735:bool)
              n436 = local read "RewCalib_Trig_L"() -> (w726:bool)
              n437 = local read "RewCalib_Trig_R"() -> (w721:bool)
              n438 = Not Equal To 0?(x=w706) -> (x != 0?=w744:bool)
              n439 = Not Equal To 0?(x=w709) -> (x != 0?=w734:bool)
              n440 = local read "MTrig_Solenoid_Tcycle__L"() -> (w743:u16)
              n441 = local read "MTrig_Solenoid_Tcycle__R"() -> (w729:u16)
              n442 = Not Equal To 0?(x=w715) -> (x != 0?=w725:bool)
              n443 = Not Equal To 0?(x=w712) -> (x != 0?=w723:bool)
              n444 = Not(x=w726) -> (.not. x?=w724:bool)
              n445 = Not(x=w721) -> (.not. x?=w722:bool)
              n446 = And(x=w725, y=w724) -> (x .and. y?=w720:bool)
              n447 = And(x=w723, y=w722) -> (x .and. y?=w719:bool)
              n448 = call "myRIO_BRig_RT_dataMTrig_Solenoid_c__L.vi"() -> ("output_Solenoid_c__L"=w752:i32)  [unwired: 11 in]
              n449 = call "myRIO_BRig_RT_dataMTrig_Solenoid_c__R.vi"() -> ("output_Solenoid_c__R"=w751:i32)  [unwired: 11 in]
              n450 = Select(t=w743, s=w744, f=u16 0) -> (s? t:f=w740:u16)
              n451 = Or(x=w720, y=w719) -> (x .or. y?=w708:bool)
              n452 = Select(t=w729, s=w734, f=u16 0) -> (s? t:f=w732:u16)
              n453 = Select(t=w740, s=w745, f=w741) -> (s? t:f=w738:u16)
              n454 = Select(t=w732, s=w735, f=w730) -> (s? t:f=w727:u16)
              n455 = call "myRIO_BRig_RT_dataMTrig_Solenoid_Tcycle__L.vi"() -> ("output_Solenoid_Tcycle__L"=w739:i32)  [unwired: 11 in]
              n456 = call "myRIO_BRig_RT_dataMTrig_Solenoid_Tcycle__R.vi"() -> ("output_Solenoid_Tcycle__R"=w728:i32)  [unwired: 11 in]
              n457 = Select(t=w707, s=w708, f=w706) -> (s? t:f=w704:u16)
              n458 = Select(t=w707, s=w708, f=w709) -> (s? t:f=w702:u16)
              n459 = Select(t=myRIO_BRig_RT__Case_NonExp_stateList."Idle" ("Enum"), s=w708, f=myRIO_BRig_RT__Case_NonExp_stateList."DispenseWater" ("Enum")) -> (s? t:f=w716:T1)
              n460 = Select(t=w707, s=w708, f=w715) -> (s? t:f=w713:u16)
              n461 = Select(t=w707, s=w708, f=w712) -> (s? t:f=w711:u16)
              n462 = Replace Array Subset(array=w749, new element #1=w750, index #1=w752, new element #2=w750, index #2=w751, new element #3=w738, index #3=w739, new element #4=w727, index #4=w728, new element #5=w713, index #5=w714, new element #6=w711, index #6=w710, new element #7=w704, index #7=w705, new element #8=w702, index #8=w703) -> (w753:u16[])
            }
            frame "DispenseWater" {
              # "D"
              # "C"
              # "B"
              # "A"
              # "(A) Add COUNT and INCREMENT\n(B) Is (A) smaller than Tcycle?\n(C) Are we dispensing water or in the delay phase?\n(D) If (A) is smaller than Tcycle   AND   if we are dispensing water\n      then send TRUE to solenoid"
              # "delay"
              # "Tcycle"
              # "Solenoid__R"
              # "count"
              # "delay"
              # "Tcycle"
              # "Solenoid__L"
              # "count"
              n463 = To Unsigned Word Integer(number=w781) -> (unsigned 16bit integer=w763:u16)
              n464 = call "myRIO_BRig_RT_dataMTrig_Solenoid_delay__R.vi"() -> ("output_Solenoid_delay__R"=w767:i32)  [unwired: 11 in]
              n465 = call "myRIO_BRig_RT_dataMTrig_Solenoid_c__R.vi"() -> ("output_Solenoid_c__R"=w766:i32)  [unwired: 11 in]
              n466 = call "myRIO_BRig_RT_dataMTrig_Solenoid_Tcycle__R.vi"() -> ("output_Solenoid_Tcycle__R"=w768:i32)  [unwired: 11 in]
              n467 = call "myRIO_BRig_RT_dataMTrig_Solenoid_delay__L.vi"() -> ("output_Solenoid_delay__L"=w783:i32)  [unwired: 11 in]
              n468 = call "myRIO_BRig_RT_dataMTrig_Solenoid_c__L.vi"() -> ("output_Solenoid_c__L"=w775:i32)  [unwired: 11 in]
              n469 = call "myRIO_BRig_RT_dataMTrig_Solenoid_Tcycle__L.vi"() -> ("output_Solenoid_Tcycle__L"=w784:i32)  [unwired: 11 in]
              n470 = Index Array(array=w777, index #1=w775, index #2=w784, index #3=w783, index #4=w766, index #5=w768, index #6=w767) -> (element #1=w782:u16, element #2=w772:u16, element #3=w780:u16, element #4=w762:u16, element #5=w759:u16, element #6=w758:u16)
              n471 = Add(x=w782, y=w763) -> (x+y=w773:u16)
              n472 = Add(x=w762, y=w763) -> (x+y=w764:u16)
              n473 = Less?(x=w773, y=w772) -> (x < y?=w756:bool)
              n474 = Equal To 0?(x=w780) -> (x = 0?=w779:bool)
              n475 = Less?(x=w764, y=w759) -> (x < y?=w757:bool)
              n476 = Equal To 0?(x=w758) -> (x = 0?=w765:bool)
              n477 = And(x=w756, y=w779) -> (x .and. y?=w778:bool)
              n478 = Or(x=w756, y=w757) -> (x .or. y?=w755:bool)
              n479 = And(x=w757, y=w765) -> (x .and. y?=w760:bool)
              n480 = Select(t=w773, s=w756, f=w772) -> (s? t:f=w774:u16)
              n481 = Select(t=w764, s=w757, f=w759) -> (s? t:f=w761:u16)
              n482 = Replace Array Subset(array=w777, new element #1=w774, index #1=w775, new element #2=w761, index #2=w766) -> (w776:u16[])
              n483 = Select(t=w771, s=w755, f=myRIO_BRig_RT__Case_NonExp_stateList."DispenseWater_post" ("Enum")) -> (s? t:f=w769:T1)
            }
            frame "DispenseWater_post" {
              # "nCycle"
              # "delay"
              # "Solenoid__R"
              # "nCycle"
              # "delay"
              # "Solenoid__L"
              n484 = call "myRIO_BRig_RT_dataMTrig_Solenoid_N__L.vi"() -> ("output_Solenoid_N__L"=w802:i32)  [unwired: 11 in]
              n485 = call "myRIO_BRig_RT_dataMTrig_Solenoid_delay__L.vi"() -> ("output_Solenoid_delay__L"=w801:i32)  [unwired: 11 in]
              n486 = call "myRIO_BRig_RT_dataMTrig_Solenoid_N__R.vi"() -> ("output_Solenoid_N__R"=w798:i32)  [unwired: 11 in]
              n487 = call "myRIO_BRig_RT_dataMTrig_Solenoid_delay__R.vi"() -> ("output_Solenoid_delay__R"=w797:i32)  [unwired: 11 in]
              n488 = Index Array(array=w804, index #1=w802, index #2=w801, index #3=w798, index #4=w797) -> (element #1=w806:u16, element #2=w805:u16, element #3=w789:u16, element #4=w791:u16)
              n489 = Not Equal To 0?(x=w806) -> (x != 0?=w807:bool)
              n490 = Not Equal To 0?(x=w789) -> (x != 0?=w790:bool)
              n491 = case shown="True" w790 {
                selector: w790 -> [_ w811]
                tunnel: w789 -> [w809 w817]
                tunnel: w791 -> [_ w818]
                tunnel: [w809 w815] -> w788
                tunnel: [u16 0 w814] -> w787
                tunnel: [_ w811] -> w786
                frame False {
                }
                frame True {
                  n492 = Equal To 0?(x=w818) -> (x = 0?=w810:bool)
                  n493 = Decrement(x=w817) -> (x-1=w816:u16)
                  n494 = Select(t=w816, s=w810, f=w817) -> (s? t:f=w815:u16)
                  n495 = Select(t=u16 1, s=w810, f=u16 0) -> (s? t:f=w814:u16)
                }
              }
              n496 = case shown="True" w807 {
                selector: w807 -> [_ w822]
                tunnel: w806 -> [w820 w828]
                tunnel: w805 -> [_ w829]
                tunnel: [w820 w826] -> w800
                tunnel: [u16 0 w825] -> w799
                tunnel: [_ w822] -> w796
                frame False {
                }
                frame True {
                  n497 = Equal To 0?(x=w829) -> (x = 0?=w821:bool)
                  n498 = Decrement(x=w828) -> (x-1=w827:u16)
                  n499 = Select(t=w827, s=w821, f=w828) -> (s? t:f=w826:u16)
                  n500 = Select(t=u16 1, s=w821, f=u16 0) -> (s? t:f=w825:u16)
                }
              }
              n501 = Or(x=w796, y=w786) -> (x .or. y?=w795:bool)
              n502 = Replace Array Subset(array=w804, new element #1=w800, index #1=w802, new element #2=w799, index #2=w801, new element #3=w788, index #3=w798, new element #4=w787, index #4=w797) -> (w803:u16[])
              n503 = Select(t=myRIO_BRig_RT__Case_NonExp_stateList."DispenseWater_pre" ("Enum"), s=w795, f=myRIO_BRig_RT__Case_NonExp_stateList."Idle" ("Enum")) -> (s? t:f=w792:T1)
            }
            frame "TestConnection" {
              n504 = local read "Host Password"() -> (w836:string)
              n505 = local read "Host UserName"() -> (w837:string)
              n506 = call "myRIO_BRig_RT_comm_webdav_testConnect.vi"("input_password"=w836, "input_username"=w837) -> ("output_Iconnected"=w834:bool)  [unwired: 9 in]
              n507 = Select(t="Connection accepted!" ("message"), s=w834, f="Error!") -> (s? t:f=w832:string)
              n508 = One Button Dialog(message=w832) -> ()  [unwired: 1 in, 1 out]
            }
            frame "SendData" {
              n509 = local read "Data Set Prefix"() -> (w839:string)
              n510 = local read "Host Password"() -> (w840:string)
              n511 = local read "Host UserName"() -> (w841:string)
              n512 = call "myRIO_BRig_RT_comm_webdav_sendData_all.vi"("Host Filename Prefix"=w839, "Host Password"=w840, "Host UserName"=w841) -> ()  [unwired: 9 in]
            }
            frame "Get_FPGA_count_per_ms" {
              n513 = case shown="False" w855 {
                selector: w855 -> [w858 _]
                tunnel: w853 -> [_ w871]
                tunnel: [w862 w871] -> w852
                tunnel: w851 -> [w861 w869]
                tunnel: w850 -> [w860 w868]
                tunnel: [w859 w866] -> w849
                tunnel: [w858 w865] -> w848
                frame False {
                  n514 = Get Date/Time In Seconds() -> (seconds since 1Jan1904=w863:timestamp)
                  n515 = xnode "Read/Write Control"("FPGA VI Reference In"=w861, "error in"=w860, "timeTrial"=TRUE) -> ("error out"=w859:errorcluster)  [unwired: 1 out]
                  n516 = To Double Precision Float(number=w863) -> (double precision float=w862:dbl)
                  n517 = local write "get_countPerMS"(w858) -> ()
                }
                frame True {
                  w867 = 1.0
                  n518 = Get Date/Time In Seconds() -> (seconds since 1Jan1904=w872:timestamp)
                  n519 = To Double Precision Float(number=w872) -> (double precision float=w873:dbl)
                  n520 = Subtract(x=w873, y=w871) -> (x-y=w870:dbl)
                  n521 = Less Or Equal?(x=w867, y=w870) -> (x <= y?=w865:bool)
                  n522 = case shown="True" w865 {
                    tunnel: w869 -> [_ w886]
                    tunnel: w868 -> [w874 w885]
                    tunnel: w867 -> [_ w876]
                    tunnel: [w874 w875] -> w866
                    frame False {
                    }
                    frame True {
                      n523 = xnode "Read/Write Control"("FPGA VI Reference In"=w886, "error in"=w885) -> ("FPGA VI Reference Out"=w883:refnum<k20>, "error out"=w882:errorcluster, "count_timeTrial"=w877:u32)
                      n524 = Multiply(x=w876, y=1000.0) -> (x*y=w880:dbl)
                      n525 = To Double Precision Float(number=w877) -> (double precision float=w879:dbl)
                      n526 = Divide(x=w879, y=w880) -> (x/y=w881:dbl)
                      n527 = local write "f_millisec2count"(w881) -> ()
                      n528 = xnode "Read/Write Control"("FPGA VI Reference In"=w883, "error in"=w882, "timeTrial"=FALSE) -> ("error out"=w875:errorcluster)  [unwired: 1 out]
                    }
                  }
                }
              }
              "error out 5" <- w849
              n529 = Select(t=myRIO_BRig_RT__Case_NonExp_stateList."Idle" ("Enum"), s=w848, f=w846) -> (s? t:f=w845:T1)
            }
            frame "End" {
            }
          }
          n530 = local read "MTrig_Audio_trig__R"() -> (w92:bool)
          n531 = local read "MTrig_Audio_trig__L"() -> (w91:bool)
          n532 = local read "START"() -> (w87:bool)
          n533 = local read "STOP_abort"() -> (w86:bool)
          n534 = local read "MTrig_Laser_trig"() -> (w93:bool)
          n535 = call "myRIO_BRig_RT_dataMTrig_main__v2.vi"("input_dataMTrig"=w95, "input_Audio_trig_L"=w91, "input_Audio_trig_R"=w92, "input_Laser_trig"=w93) -> ("output_dataMTrig"=w94:u16[], "output_Audio_L"=w71:bool, "output_Audio_R"=w82:bool, "output_Laser"=w74:bool)  [unwired: 12 in]
          n536 = Or(x=w87, y=w86) -> (x .or. y?=w85:bool)
          n537 = Select(t=myRIO_BRig_RT__Case_NonExp_stateList."End" ("Enum"), s=w85, f=w84) -> (s? t:f=w83:T1)
          n538 = Or(x=w92, y=w93) -> (x .or. y?=w90:bool)
          n539 = Or(x=w90, y=w91) -> (x .or. y?=w89:bool)
          n540 = case shown="True" w89 {
            frame False {
            }
            frame True {
              w108 = FALSE
              n541 = local write "MTrig_Audio_trig__R"(w108) -> ()
              n542 = local write "MTrig_Audio_trig__L"(w108) -> ()
              n543 = local write "MTrig_Laser_trig"(w108) -> ()
            }
          }
          n544 = xnode "Read/Write Control"("FPGA VI Reference In"=w60, "error in"=w59, "A1_SR"=w96, "A3_SL"=w97, "audioTrigger_L"=w71, "audioTrigger_R"=w82, "laserResponse_reward_LED"="laserResponse_reward_LED", "laserResponse_wrong_LED"="laserResponse_wrong_LED", "laserResponse_reward"="laserResponse_reward", "laserResponse_wrong"="laserResponse_wrong", "SelectionState"="SelectionState", "ignoreWrong"="ignoreWrong", "Left(F)_or_Right(T)"="Left(F)_or_Right(T)", "laserMTrig"=w74) -> ("FPGA VI Reference Out"=w102:refnum<k20>, "error out"=w101:errorcluster, "SelectReward"=→"SelectReward":bool, "SelectWrong"=→"SelectWrong":bool)
          n545 = node-c288() -> ()  [unwired: 1 in, 1 out]
          "cState_NonExp" <- w100
        }
        n546 = node-c288(w50) -> ()  [unwired: 1 out]
        n547 = flat-sequence {
          tunnel: w43 -> [w54]
          tunnel: [w54] -> w42
          tunnel: w41 -> [w53]
          tunnel: [w53] -> w40
          frame #0 {
            w52 = FALSE
            n548 = local write "STOP_endBlock"(w52) -> ()
            n549 = local write "STOP_endTrial"(w52) -> ()
          }
        }
      }
      frame True {
        w896 = u8 0
        w898 = FALSE ("SelectionState")
        w903 = u16 0 ("idxDataBlock")
        w905 = u16 100 ("new element/subarray")
        w906 = u16 100 ("new element/subarray")
        w926 = T6 refnum items=["Session NI_WebDAV"] ("output_hSession")
        w935 = FALSE
        w936 = u16 0
        w897 = FALSE
        # "audio__L\naudio__R"
        # "Audio params"
        # "nRewards"
        # "idxDataBlock"
        # "Solenoid_Tdelay_R"
        # "Solenoid_Tdelay_L"
        # "RewCalib_N__R"
        # "RewCalib_N__L"
        # "Save dataLick to file\nSend file to Host\nSave dataMTrig\nSend file to Host\nDisconnect"
        # "dataTrial"
        # "dataTrial"
        # "Solenoid_Tcycle_R"
        # "Solenoid_Tcycle_L"
        # "Laser_Tcycle"
        # "Audio_Tcycle_R"
        # "Audio_Tcycle_L"
        # "dataLick"
        # "dataLC"
        # "dataLC"
        # "dataBlock"
        # "dataBlock"
        # "dataMTrig"
        # "dataMTrig"
        # "dataExp"
        # "dataCurrent"
        # "dataExp"
        # "dataCurrent"
        # "spout"
        # "state"
        n550 = call "myRIO_BRig_RT_dataMTrig_Solenoid_Tcycle__L.vi"() -> ("output_Solenoid_Tcycle__L"=w932:i32)  [unwired: 11 in]
        n551 = call "myRIO_BRig_RT_dataMTrig_Solenoid_Tcycle__R.vi"() -> ("output_Solenoid_Tcycle__R"=w931:i32)  [unwired: 11 in]
        n552 = call "myRIO_BRig_RT_dataMTrig_Audio_Tcycle__L.vi"() -> ("output_Audio_Tcycle__L"=w930:i32)  [unwired: 11 in]
        n553 = call "myRIO_BRig_RT_dataMTrig_Audio_Tcycle__R.vi"() -> ("output_Audio_Tcycle__R"=w929:i32)  [unwired: 11 in]
        n554 = call "myRIO_BRig_RT_dataMTrig_Laser_Tcycle.vi"() -> ("output_Laser_Tcycle"=w928:i32)  [unwired: 11 in]
        n555 = local read "MTrig_Solenoid_Tcycle__L"() -> (w911:u16)
        n556 = local read "MTrig_Solenoid_Tcycle__R"() -> (w910:u16)
        n557 = local read "Tcycle_Reward_L"() -> (w907:u16)
        n558 = local read "Tcycle_Reward_R"() -> (w908:u16)
        n559 = local read "MTrig_Laser_Tcycle"() -> (w909:u16)
        n560 = call "myRIO_BRig_RT_dataMTrig_Solenoid_RewCalib_nCycle__L.vi"() -> ("output_Solenoid_RewCalib_nCycle__L"=w914:i32)  [unwired: 11 in]
        n561 = call "myRIO_BRig_RT_dataMTrig_Solenoid_Tdelay__L.vi"() -> ("output_Solenoid_Tdelay__L"=w916:i32)  [unwired: 11 in]
        n562 = call "myRIO_BRig_RT_dataMTrig_Solenoid_RewCalib_nCycle__R.vi"() -> ("output_Solenoid_RewCalib_nCycle__R"=w915:i32)  [unwired: 11 in]
        n563 = call "myRIO_BRig_RT_dataMTrig_Solenoid_Tdelay__R.vi"() -> ("output_Solenoid_Tdelay__R"=w917:i32)  [unwired: 11 in]
        n564 = call "myRIO_BRig_RT_dataLick_init.vi"() -> ("output_dataLick"=w938:u16[][])  [unwired: 11 in]
        n565 = call "myRIO_BRig_RT_dataCurrent_init.vi"() -> ("output_dataCurrent"=w945:u16[])  [unwired: 11 in]
        n566 = call "myRIO_BRig_RT_dataExp_init.vi"() -> ("output_dataExp"=w944:u16[])  [unwired: 11 in]
        n567 = call "myRIO_BRig_RT_dataMTrig_init.vi"() -> ("output_dataMTrig"=w934:u16[])  [unwired: 5 in]
        n568 = call "myRIO_BRig_RT_dataLC_init.vi"() -> ("output_dataLC"=w942:u16[])  [unwired: 11 in]
        n569 = call "myRIO_BRig_RT_dataBlock_init.vi"() -> ("output_dataBlock"=w943:u16[][])  [unwired: 11 in]
        n570 = call "myRIO_BRig_RT_dataTrial_init.vi"() -> ("output_dataTrial"=w927:u16[][])  [unwired: 11 in]
        n571 = xnode "Read/Write Control"("FPGA VI Reference In"=w899, "error in"=w900, "SelectionState"=w898, "laserResponse_reward"=w898, "laserResponse_wrong"=w898, "laserResponse_reward_LED"=w898, "laserResponse_wrong_LED"=w898, "Left(F)_or_Right(T)"=w898, "ignoreWrong"=w898, "SelectionState"=w898) -> ("FPGA VI Reference Out"=w901:refnum<k20>, "error out"=w902:errorcluster)
        n572 = Replace Array Subset(array=w934, new element #1=w906, index #1=w914, new element #2=w906, index #2=w915, new element #3=w905, index #3=w916, new element #4=w905, index #4=w917, new element #5=w911, index #5=w932, new element #6=w910, index #6=w931, new element #7=w907, index #7=w930, new element #8=w908, index #8=w929, new element #9=w909, index #9=w928) -> (w933:u16[])
        n573 = Get Date/Time In Seconds() -> (seconds since 1Jan1904=w913:timestamp)
        n574 = To Double Precision Float(number=w913) -> (double precision float=w912:dbl)
        n575 = node-c288() -> (w953:T3)  [unwired: 4 in]
        n576 = timed-loop {
          timing: w953 -> [_]
          timing-out: [_] -> w952
          shift-right: [w1032] -> _
          shift-left: myRIO_BRig_RT__Case_Exp_stateList."Start1" ("Enum") -> [w1063]
          shift-right: [w1084] -> _
          shift-left: enum16{"Left", "Right"}."Left" -> [w1086]
          tunnel: w901 -> [w1083]
          tunnel: w902 -> [w1082]
          shift-right: [w1077] -> _
          shift-left: w950 -> [w1081]
          shift-right: [w1076] -> _
          shift-left: w949 -> [w1080]
          tunnel: [w1057] -> w947
          tunnel: [w1058] -> w948
          shift-right: [w1059] -> w918
          shift-left: w945 -> [w1024]
          shift-right: [w1075] -> _
          shift-left: w944 -> [w1019]
          shift-right: [w1046] -> w922
          shift-left: w933 -> [w1047]
          shift-right: [w1073] -> _
          shift-left: w943 -> [w1074]
          shift-right: [w1071] -> _
          shift-left: w942 -> [w1072]
          shift-right: [w1005] -> _
          shift-left: w897 -> [w1070]
          shift-right: [w1061] -> w924
          shift-left: w938 -> [w1062]
          shift-right: [w1048] -> _
          shift-left: w936 -> [w1056]
          shift-right: [w1016] -> _
          shift-left: w896 -> [w1055]
          shift-right: [w1049] -> _
          shift-left: w936 -> [w1054]
          shift-right: [w1050] -> _
          shift-left: w896 -> [w1053]
          shift-right: [w1017] -> _
          shift-left: w935 -> [w1051]
          shift-right: [w1018] -> _
          shift-left: w935 -> [w1052]
          shift-right: [w1030] -> _
          shift-left: w927 -> [w1031]
          shift-right: [w1029] -> w920
          shift-left: w926 -> [w1027]
          shift-right: [w1028] -> w921
          shift-left: FALSE ("output_Iconnected") -> [w1026]
          tunnel: "Data Set Prefix" -> [w1025]
          tunnel: [w1025] -> w919
          shift-right: [w1000] -> _
          shift-left: w897 -> [w1023]
          tunnel: w912 -> [w1020]
          shift-right: [w1014] -> _
          shift-left: 0 ("idxDataBlock") -> [w1015]
          shift-right: [w1011] -> _
          shift-left: w903 -> [w1013]
          shift-right: [w1010] -> _
          shift-left: w903 -> [w1012]
          shift-right: [w999] -> _
          shift-left: w897 -> [w1006]
          shift-right: [w1002] -> _
          shift-left: w897 -> [w1004]
          shift-right: [w1001] -> _
          shift-left: w897 -> [w1003]
          shift-right: [w992] -> _
          shift-left: w897 -> [w993]
          stop <- w1069 stop-if-true
          # "Laser"
          # "Audio R"
          # "Audio L"
          # "Solenoid R"
          # "Solenoid L"
          # "manual triggering"
          # "dataTrial"
          # "dataBlock"
          # "nRewards"
          # "laserOccurred"
          # "dataExp"
          # "dataCurrent"
          # "audio__L\naudio__R"
          # "time stamp"
          # "Audio params"
          # "nRewards"
          # "idxDataBlock"
          # "idxDataBlock"
          # "activate"
          # "audio__L\naudio__R"
          # "amp__R\nfreq__R"
          # "amp__L\nfreq__L"
          # "dataLC"
          # "solenoid__R"
          # "solenoid__L"
          # "Did a lick occur?"
          # "Update lick counter"
          # "spout"
          # "spout"
          # "state"
          # "state"
          n577 = node-c288() -> ()  [unwired: 1 in, 1 out]
          n578 = local read "MTrig_Solenoid_trig__L"() -> (w1044:bool)
          n579 = local read "MTrig_Solenoid_trig__R"() -> (w1043:bool)
          n580 = local read "MTrig_Audio_trig__L"() -> (w1042:bool)
          n581 = local read "MTrig_Audio_trig__R"() -> (w1041:bool)
          n582 = xnode "Read/Write Control"("FPGA VI Reference In"=w1083, "error in"=w1082) -> ("FPGA VI Reference Out"=w1009:refnum<k20>, "error out"=w1008:errorcluster, "A2_LickL"=w1077:u32, "A4_LickR"=w1076:u32)
          "A2" <- w1077
          "A4" <- w1076
          n583 = local read "MTrig_Laser_trig"() -> (w1040:bool)
          n584 = Greater?(x=w1077, y=w1081) -> (0:w1079:bool)
          n585 = Greater?(x=w1076, y=w1080) -> (0:w1078:bool)
          n586 = Or(x=w1079, y=w1078) -> (x .or. y?=w1085:bool)
          n587 = call "myRIO_BRig_RT_dataMTrig_main.vi"("input_dataMTrig"=w1047, "input_Solenoid_trig_L"=w1044, "input_Solenoid_trig_R"=w1043, "input_Audio_trig_L"=w1042, "input_Audio_trig_R"=w1041, "input_Laser_trig"=w1040) -> ("output_Laser"=w997:bool, "output_dataMTrig"=w1046:u16[], "output_Solenoid_L"=w1034:bool, "output_Solenoid_R"=w1036:bool, "output_Audio_L"=w1038:bool, "output_Audio_R"=w1039:bool)  [unwired: 8 in]
          n588 = Compound Arithmetic op=OR(w1044, w1043, w1042, w1041, w1040) -> (w1045:bool)
          n589 = case shown="True" w1045 {
            frame False {
            }
            frame True {
              w1087 = FALSE
              n590 = local write "MTrig_Solenoid_trig__L"(w1087) -> ()
              n591 = local write "MTrig_Solenoid_trig__R"(w1087) -> ()
              n592 = local write "MTrig_Audio_trig__L"(w1087) -> ()
              n593 = local write "MTrig_Audio_trig__R"(w1087) -> ()
              n594 = local write "MTrig_Laser_trig"(w1087) -> ()
            }
          }
          n595 = case shown="\"initTrial3\"" w1063 {
            selector: w1063 -> [_ _ _ _ _ _ _ _ _ _ _ _ _ _ _ _ _ _ _ _ w1824 _ w1889 _ _ _ _ _ w2031 _ w2106 _ _ _ _ _ w2235 _ w2311 _ w2375 _ w2419 _ _ w2489 _ _ _ _ _ w2661 _ _ _ _ _ _ _ _ _ _ _ _ _ _ _ _ _ _ _]
            tunnel: [myRIO_BRig_RT__Case_Exp_stateList."Start2" ("Enum") myRIO_BRig_RT__Case_Exp_stateList."Start3" ("Enum") myRIO_BRig_RT__Case_Exp_stateList."saveSettings1" ("Enum") myRIO_BRig_RT__Case_Exp_stateList."saveSettings2" ("Enum") myRIO_BRig_RT__Case_Exp_stateList."saveSettings3" ("Enum") myRIO_BRig_RT__Case_Exp_stateList."saveSettings4_LC_ENL" ("Enum") myRIO_BRig_RT__Case_Exp_stateList."saveSettings5_LC_Cue" ("Enum") myRIO_BRig_RT__Case_Exp_stateList."saveSettings6_LC_Other" ("Enum") myRIO_BRig_RT__Case_Exp_stateList."setSettings_Audio" ("Enum") myRIO_BRig_RT__Case_Exp_stateList."setSettings_Laser" ("Enum") myRIO_BRig_RT__Case_Exp_stateList."commConnect" ("Enum") w1585 myRIO_BRig_RT__Case_Exp_stateList."initTrial" ("Enum") w1629 myRIO_BRig_RT__Case_Exp_stateList."initTrial3" ("Enum") myRIO_BRig_RT__Case_Exp_stateList."initTrial_LC_ENL1" ("Enum") myRIO_BRig_RT__Case_Exp_stateList."ENL1_pre" ("Enum") myRIO_BRig_RT__Case_Exp_stateList."initTrial_LC_Cue1" ("Enum") myRIO_BRig_RT__Case_Exp_stateList."initTrial4" ("Enum") w1783 w1821 myRIO_BRig_RT__Case_Exp_stateList."ENL1Penalty" ("Enum") w1890 myRIO_BRig_RT__Case_Exp_stateList."endExp" ("Enum") myRIO_BRig_RT__Case_Exp_stateList."endExp" ("Enum") myRIO_BRig_RT__Case_Exp_stateList."endExp" ("Enum") myRIO_BRig_RT__Case_Exp_stateList."endExp" ("Enum") w1985 w2030 myRIO_BRig_RT__Case_Exp_stateList."Cue1Penalty" ("Enum") w2104 myRIO_BRig_RT__Case_Exp_stateList."endExp" ("Enum") myRIO_BRig_RT__Case_Exp_stateList."endExp" ("Enum") myRIO_BRig_RT__Case_Exp_stateList."endExp" ("Enum") myRIO_BRig_RT__Case_Exp_stateList."endExp" ("Enum") w2192 w2243 myRIO_BRig_RT__Case_Exp_stateList."SelectReward" ("Enum") w2312 myRIO_BRig_RT__Case_Exp_stateList."SelectRewardPost" ("Enum") w2376 myRIO_BRig_RT__Case_Exp_stateList."SelectWrong" ("Enum") w2415 myRIO_BRig_RT__Case_Exp_stateList."endTrial1" ("Enum") myRIO_BRig_RT__Case_Exp_stateList."SelectTimeout" ("Enum") w2491 myRIO_BRig_RT__Case_Exp_stateList."endTrial1" ("Enum") myRIO_BRig_RT__Case_Exp_stateList."endTrial2" ("Enum") myRIO_BRig_RT__Case_Exp_stateList."saveData_dataBlock" ("Enum") w2574 w2644 w2661 myRIO_BRig_RT__Case_Exp_stateList."initBlock" ("Enum") w2688 myRIO_BRig_RT__Case_Exp_stateList."commUpload_dataCurrent" ("Enum") myRIO_BRig_RT__Case_Exp_stateList."commUpload_dataExp" ("Enum") myRIO_BRig_RT__Case_Exp_stateList."commUpload_dataLC" ("Enum") myRIO_BRig_RT__Case_Exp_stateList."commUpload_dataTrial" ("Enum") myRIO_BRig_RT__Case_Exp_stateList."endTrial3" ("Enum") myRIO_BRig_RT__Case_Exp_stateList."saveData_dataCurrent" ("Enum") myRIO_BRig_RT__Case_Exp_stateList."saveData_dataExp" ("Enum") myRIO_BRig_RT__Case_Exp_stateList."saveData_dataLC" ("Enum") myRIO_BRig_RT__Case_Exp_stateList."saveData_dataTrial" ("Enum") myRIO_BRig_RT__Case_Exp_stateList."commUpload_pre" ("Enum") myRIO_BRig_RT__Case_Exp_stateList."empty_endBlock2" ("Enum") myRIO_BRig_RT__Case_Exp_stateList."initBlock" ("Enum") myRIO_BRig_RT__Case_Exp_stateList."empty_endTrial2" ("Enum") myRIO_BRig_RT__Case_Exp_stateList."empty_endTrial3" ("Enum") myRIO_BRig_RT__Case_Exp_stateList."empty_endTrial4" ("Enum") myRIO_BRig_RT__Case_Exp_stateList."empty_endTrial5" ("Enum") myRIO_BRig_RT__Case_Exp_stateList."initTrial" ("Enum")] -> w1032
            tunnel: [w1113 w1132 w1154 w1209 w1257 w1324 w1376 w1428 w1472 w1498 w1557 w1561 w1593 w1610 w1645 w1675 w1708 w1732 w1758 w1799 w1837 w1867 w1894 w1910 w1932 w1951 w1970 w2004 w2052 w2077 w2103 w2124 w2145 w2164 w2183 w2203 w2261 w2286 w2309 w2323 w2373 w2397 w2429 w2450 w2470 w2502 w2525 w2537 w2556 w2598 w2617 w2660 w2677 w2691 w2725 w2746 w2767 w2788 w2809 w2837 w2857 w2884 w2904 w2929 w2948 w2967 w2986 w3005 w3024 w3043 w3062] -> w1084
            tunnel: w1086 -> [w1113 w1132 w1154 w1209 w1257 w1324 w1376 w1428 w1472 w1498 w1557 w1584 w1593 w1610 w1645 w1675 w1708 w1732 w1758 w1799 w1837 w1867 w1894 w1910 w1932 w1951 w1970 w2004 w2052 w2077 w2103 w2124 w2145 w2164 w2183 w2203 w2261 w2286 w2309 w2323 w2373 w2397 w2429 w2450 w2470 w2502 w2525 w2537 w2556 w2598 w2617 w2660 w2677 w2691 w2725 w2746 w2767 w2788 w2809 w2837 w2857 w2884 w2904 w2929 w2948 w2967 w2986 w3005 w3024 w3043 w3062]
            tunnel: w1085 -> [w1116 w1135 w1151 w1212 w1260 w1327 w1379 w1431 w1475 w1501 w1560 w1578 w1604 w1630 w1663 w1691 w1722 w1745 w1771 w1786 w1818 w1870 w1897 w1916 w1935 w1954 w1973 w1984 w2029 w2085 w2110 w2129 w2148 w2167 w2186 w2201 w2259 w2296 w2319 w2354 w2381 w2408 w2432 w2449 w2482 w2507 w2522 w2545 w2555 w2609 w2643 w2664 w2674 w2700 w2728 w2749 w2770 w2791 w2812 w2840 w2860 w2887 w2907 w2932 w2951 w2970 w2989 w3008 w3027 w3046 w3065]
            tunnel: w1079 -> [w1115 w1134 w1152 w1211 w1259 w1326 w1378 w1430 w1474 w1500 w1559 w1577 w1603 w1631 w1662 w1692 w1723 w1746 w1772 w1809 w1839 w1869 w1896 w1915 w1934 w1953 w1972 w2018 w2053 w2084 w2109 w2128 w2147 w2166 w2185 w2202 w2258 w2295 w2318 w2353 w2380 w2407 w2431 w2448 w2481 w2506 w2523 w2546 w2554 w2608 w2642 w2663 w2675 w2701 w2727 w2748 w2769 w2790 w2811 w2839 w2859 w2886 w2906 w2931 w2950 w2969 w2988 w3007 w3026 w3045 w3064]
            tunnel: w1078 -> [w1114 w1133 w1153 w1210 w1258 w1325 w1377 w1429 w1473 w1499 w1558 w1576 w1602 w1632 w1661 w1693 w1724 w1747 w1773 w1808 w1838 w1868 w1895 w1914 w1933 w1952 w1971 w2017 w2054 w2083 w2108 w2127 w2146 w2165 w2184 w2221 w2262 w2294 w2317 w2352 w2379 w2406 w2430 w2447 w2480 w2505 w2524 w2547 w2553 w2607 w2641 w2662 w2676 w2702 w2726 w2747 w2768 w2789 w2810 w2838 w2858 w2885 w2905 w2930 w2949 w2968 w2987 w3006 w3025 w3044 w3063]
            tunnel: [w1116 w1135 w1151 w1212 w1260 w1327 w1379 w1431 w1475 w1501 w1560 w1578 w1604 w1630 w1663 w1691 w1722 w1745 w1771 w1786 w1818 w1870 w1897 w1916 w1935 w1954 w1973 w1984 w2029 w2085 w2110 w2129 w2148 w2167 w2186 w2201 w2259 w2296 w2319 w2354 w2381 w2408 w2432 w2449 w2482 w2507 w2522 w2545 w2555 w2609 w2643 w2664 w2674 w2700 w2728 w2749 w2770 w2791 w2812 w2840 w2860 w2887 w2907 w2932 w2951 w2970 w2989 w3008 w3027 w3046 w3065] -> w1066
            tunnel: [w1115 w1134 w1152 w1211 w1259 w1326 w1378 w1430 w1474 w1500 w1559 w1577 w1603 w1631 w1662 w1692 w1723 w1746 w1772 w1809 w1839 w1869 w1896 w1915 w1934 w1953 w1972 w2018 w2053 w2084 w2109 w2128 w2147 w2166 w2185 w2202 w2258 w2295 w2318 w2353 w2380 w2407 w2431 w2448 w2481 w2506 w2523 w2546 w2554 w2608 w2642 w2663 w2675 w2701 w2727 w2748 w2769 w2790 w2811 w2839 w2859 w2886 w2906 w2931 w2950 w2969 w2988 w3007 w3026 w3045 w3064] -> w1065
            tunnel: [w1114 w1133 w1153 w1210 w1258 w1325 w1377 w1429 w1473 w1499 w1558 w1576 w1602 w1632 w1661 w1693 w1724 w1747 w1773 w1808 w1838 w1868 w1895 w1914 w1933 w1952 w1971 w2017 w2054 w2083 w2108 w2127 w2146 w2165 w2184 w2221 w2262 w2294 w2317 w2352 w2379 w2406 w2430 w2447 w2480 w2505 w2524 w2547 w2553 w2607 w2641 w2662 w2676 w2702 w2726 w2747 w2768 w2789 w2810 w2838 w2858 w2885 w2905 w2930 w2949 w2968 w2987 w3006 w3025 w3044 w3063] -> w1064
            tunnel: w1024 -> [w1112 w1131 w1150 w1176 w1233 w1301 w1375 w1427 w1471 w1496 w1517 w1583 w1592 w1628 w1634 w1676 w1703 w1729 w1757 w1798 w1823 w1861 w1893 w1911 w1931 w1950 w1969 w1988 w2049 w2076 w2107 w2125 w2144 w2163 w2182 w2212 w2239 w2278 w2314 w2325 w2378 w2398 w2428 w2446 w2471 w2504 w2521 w2534 w2558 w2578 w2615 w2659 w2678 w2703 w2722 w2743 w2764 w2785 w2796 w2826 w2845 w2869 w2901 w2918 w2938 w2957 w2976 w2995 w3014 w3033 w3052]
            tunnel: w1019 -> [w1111 w1130 w1149 w1207 w1255 w1321 w1373 w1425 w1469 w1489 w1553 w1582 w1601 w1627 w1642 w1674 w1710 w1735 w1761 w1801 w1836 w1860 w1891 w1913 w1930 w1949 w1968 w2006 w2051 w2074 w2102 w2126 w2143 w2162 w2181 w2214 w2260 w2292 w2316 w2346 w2374 w2399 w2426 w2445 w2473 w2501 w2520 w2544 w2561 w2577 w2634 w2658 w2679 w2704 w2721 w2742 w2763 w2784 w2797 w2834 w2854 w2865 w2900 w2926 w2945 w2964 w2983 w3002 w3021 w3040 w3059]
            tunnel: [w1112 w1131 w1150 w1176 w1233 w1300 w1375 w1427 w1471 w1496 w1539 w1567 w1592 w1616 w1634 w1676 w1703 w1728 w1756 w1802 w1822 w1862 w1892 w1911 w1931 w1950 w1969 w2013 w2048 w2075 w2105 w2125 w2144 w2163 w2182 w2215 w2234 w2293 w2313 w2347 w2377 w2400 w2427 w2446 w2474 w2503 w2521 w2533 w2557 w2578 w2613 w2659 w2678 w2703 w2722 w2743 w2764 w2785 w2796 w2826 w2845 w2869 w2901 w2918 w2938 w2957 w2976 w2995 w3014 w3033 w3052] -> w1060
            tunnel: [w1111 w1130 w1149 w1206 w1254 w1316 w1373 w1425 w1469 w1489 w1553 w1581 w1601 w1626 w1642 w1674 w1710 w1735 w1761 w1801 w1836 w1860 w1891 w1913 w1930 w1949 w1968 w2006 w2051 w2074 w2102 w2126 w2143 w2162 w2181 w2214 w2260 w2292 w2316 w2346 w2374 w2399 w2426 w2445 w2473 w2501 w2520 w2544 w2561 w2577 w2634 w2658 w2679 w2704 w2721 w2742 w2763 w2784 w2797 w2834 w2854 w2868 w2900 w2926 w2945 w2964 w2983 w3002 w3021 w3040 w3059] -> w1075
            tunnel: [_ _ _ _ _ _ _ _ _ _ _ _ _ _ _ _ _ _ _ _ _ _ _ _ _ _ _ _ _ _ _ _ _ _ _ _ _ _ w2307 _ _ _ _ _ _ _ _ _ _ _ _ _ _ _ _ _ _ _ _ _ _ _ _ _ _ _ _ _ _ _ _] -> w1035
            tunnel: [_ _ _ _ _ _ _ _ _ _ _ _ _ _ _ _ _ _ _ _ _ _ _ _ _ _ _ _ _ _ _ _ _ _ _ _ _ _ w2308 _ _ _ _ _ _ _ _ _ _ _ _ _ _ _ _ _ _ _ _ _ _ _ _ _ _ _ _ _ _ _ _] -> w1037
            tunnel: w1074 -> [w1109 w1128 w1147 w1178 w1235 w1322 w1374 w1426 w1470 w1494 w1554 w1579 w1594 w1624 w1654 w1689 w1720 w1725 w1753 w1800 w1835 w1857 w1887 w1912 w1928 w1947 w1966 w2012 w2050 w2073 w2100 w2122 w2141 w2160 w2179 w2213 w2256 w2284 w2315 w2327 w2371 w2396 w2424 w2443 w2472 w2500 w2518 w2536 w2563 w2605 w2626 w2656 w2681 w2706 w2719 w2740 w2761 w2782 w2806 w2820 w2847 w2875 w2894 w2920 w2939 w2958 w2977 w2996 w3015 w3034 w3053]
            tunnel: [w1109 w1128 w1147 w1178 w1235 w1322 w1374 w1426 w1470 w1494 w1554 w1579 w1591 w1624 w1654 w1689 w1720 w1725 w1753 w1800 w1835 w1857 w1887 w1912 w1928 w1947 w1966 w2012 w2050 w2073 w2100 w2122 w2141 w2160 w2179 w2213 w2256 w2284 w2315 w2326 w2371 w2396 w2424 w2443 w2472 w2500 w2518 w2535 w2563 w2605 w2626 w2656 w2681 w2706 w2719 w2740 w2761 w2782 w2806 w2820 w2847 w2875 w2894 w2920 w2939 w2958 w2977 w2996 w3015 w3034 w3053] -> w1073
            tunnel: w1072 -> [w1110 w1129 w1148 w1177 w1234 w1323 w1371 w1423 w1467 w1495 w1555 w1580 w1600 w1625 w1633 w1690 w1721 w1733 w1759 w1797 w1817 w1858 w1888 w1909 w1929 w1948 w1967 w2011 w2028 w2072 w2101 w2123 w2142 w2161 w2180 w2211 w2257 w2285 w2310 w2344 w2372 w2395 w2425 w2444 w2469 w2498 w2519 w2543 w2562 w2606 w2633 w2657 w2680 w2705 w2720 w2741 w2762 w2783 w2807 w2833 w2853 w2881 w2892 w2925 w2944 w2963 w2982 w3001 w3020 w3039 w3058]
            tunnel: [w1110 w1129 w1148 w1177 w1234 w1323 w1372 w1424 w1468 w1495 w1555 w1580 w1600 w1625 w1633 w1690 w1721 w1733 w1759 w1797 w1817 w1858 w1888 w1909 w1929 w1948 w1967 w2011 w2028 w2072 w2101 w2123 w2142 w2161 w2180 w2211 w2257 w2285 w2310 w2344 w2372 w2395 w2425 w2444 w2469 w2498 w2519 w2543 w2562 w2606 w2633 w2657 w2680 w2705 w2720 w2741 w2762 w2783 w2807 w2833 w2853 w2881 w2892 w2925 w2944 w2963 w2982 w3001 w3020 w3039 w3058] -> w1071
            tunnel: w1070 -> [_ _ _ _ _ _ _ _ _ _ _ _ _ _ _ _ _ _ _ w1782 w1810 w1843 w1876 _ _ _ _ _ w2022 w2059 _ _ _ _ _ _ _ _ _ _ _ _ _ _ _ w2499 _ _ _ _ _ _ _ _ _ _ _ _ _ _ _ _ _ _ _ _ _ _ _ _ _]
            tunnel: [_ _ _ _ _ _ _ _ _ _ _ _ _ _ _ _ _ _ _ _ _ _ _ _ _ _ _ _ _ _ _ _ _ _ _ _ _ _ _ _ _ _ _ _ _ _ _ _ _ _ _ TRUE _ _ _ _ _ _ _ _ _ _ _ _ _ _ _ _ _ _ _] -> w1067
            tunnel: w1056 -> [w1107 w1126 w1145 w1168 w1228 w1311 w1358 w1410 w1439 _ w1545 w1575 w1599 w1623 w1653 w1688 w1719 w1744 w1770 w1796 w1834 w1855 w1886 w1907 w1926 w1945 w1964 w2010 w2045 w2070 w2099 w2120 w2139 w2158 w2177 w2210 w2255 w2274 w2306 w2342 w2370 w2393 w2423 w2442 w2467 w2497 w2517 w2541 w2567 w2604 w2630 w2654 w2672 w2699 w2717 w2738 w2759 w2780 w2804 w2831 w2851 w2879 w2898 w2924 w2943 w2962 w2981 w3000 w3019 w3038 w3057]
            tunnel: w1055 -> [w1106 w1125 w1144 w1167 w1227 w1310 w1357 w1409 w1440 _ w1544 w1574 w1598 w1622 w1652 w1687 w1718 w1743 w1769 w1795 w1833 w1854 w1885 w1906 w1925 w1944 w1963 w2009 w2044 w2069 w2098 w2119 w2138 w2157 w2176 w2209 w2254 w2273 w2305 w2341 w2369 w2392 w2422 w2441 w2466 w2496 w2516 w2540 w2566 w2603 w2629 w2653 w2671 w2698 w2716 w2737 w2758 w2779 w2803 w2830 w2850 w2878 w2897 w2923 w2942 w2961 w2980 w2999 w3018 w3037 w3056]
            tunnel: w1054 -> [w1105 w1124 w1143 w1166 w1226 w1309 w1356 w1408 w1441 _ w1543 w1573 w1597 w1621 w1651 w1686 w1717 w1742 w1768 w1794 w1832 w1853 w1884 w1905 w1924 w1943 w1962 w2008 w2043 w2068 w2097 w2118 w2137 w2156 w2175 w2208 w2253 w2272 w2304 w2340 w2368 w2391 w2421 w2440 w2465 w2495 w2515 w2539 w2565 w2602 w2628 w2652 w2670 w2697 w2715 w2736 w2757 w2778 w2802 w2829 w2849 w2877 w2896 w2922 w2941 w2960 w2979 w2998 w3017 w3036 w3055]
            tunnel: w1053 -> [w1104 w1123 w1142 w1165 w1225 w1308 w1355 w1407 w1442 _ w1542 w1572 w1596 w1620 w1650 w1685 w1716 w1741 w1767 w1793 w1831 w1852 w1883 w1904 w1923 w1942 w1961 w2007 w2042 w2067 w2096 w2117 w2136 w2155 w2174 w2207 w2252 w2271 w2303 w2339 w2367 w2390 w2420 w2439 w2464 w2494 w2514 w2538 w2564 w2601 w2627 w2651 w2669 w2696 w2714 w2735 w2756 w2777 w2801 w2828 w2848 w2876 w2895 w2921 w2940 w2959 w2978 w2997 w3016 w3035 w3054]
            tunnel: w1052 -> [_ _ _ _ _ _ _ _ _ _ _ _ _ _ _ _ _ _ _ _ _ _ _ _ _ _ _ _ w2047 _ _ _ _ _ _ _ _ _ _ _ _ _ _ _ _ _ _ _ _ _ _ _ _ _ _ _ _ _ _ _ _ _ _ _ _ _ _ _ _ _ _]
            tunnel: w1051 -> [_ _ _ _ _ _ _ _ _ _ _ _ _ _ _ _ _ _ _ _ _ _ _ _ _ _ _ _ w2046 _ _ _ _ _ _ _ _ _ _ _ _ _ _ _ _ _ _ _ _ _ _ _ _ _ _ _ _ _ _ _ _ _ _ _ _ _ _ _ _ _ _]
            tunnel: [w1107 w1126 w1145 w1168 w1228 w1311 w1358 w1410 w1439 w1488 w1545 w1575 w1599 w1623 w1653 w1688 w1719 w1744 w1770 w1796 w1834 w1855 w1886 w1907 w1926 w1945 w1964 w2010 w2045 w2070 w2099 w2120 w2139 w2158 w2177 w2210 w2255 w2274 w2306 w2342 w2370 w2393 w2423 w2442 w2467 w2497 w2517 w2541 w2567 w2604 w2630 w2654 w2672 w2699 w2717 w2738 w2759 w2780 w2804 w2831 w2851 w2879 w2898 w2924 w2943 w2962 w2981 w3000 w3019 w3038 w3057] -> w1048
            tunnel: [w1106 w1125 w1144 w1167 w1227 w1310 w1357 w1409 w1440 w1479 w1544 w1574 w1598 w1622 w1652 w1687 w1718 w1743 w1769 w1795 w1833 w1854 w1885 w1906 w1925 w1944 w1963 w2009 w2044 w2069 w2098 w2119 w2138 w2157 w2176 w2209 w2254 w2273 w2305 w2341 w2369 w2392 w2422 w2441 w2466 w2496 w2516 w2540 w2566 w2603 w2629 w2653 w2671 w2698 w2716 w2737 w2758 w2779 w2803 w2830 w2850 w2878 w2897 w2923 w2942 w2961 w2980 w2999 w3018 w3037 w3056] -> w1016
            tunnel: [w1105 w1124 w1143 w1166 w1226 w1309 w1356 w1408 w1441 w1487 w1543 w1573 w1597 w1621 w1651 w1686 w1717 w1742 w1768 w1794 w1832 w1853 w1884 w1905 w1924 w1943 w1962 w2008 w2043 w2068 w2097 w2118 w2137 w2156 w2175 w2208 w2253 w2272 w2304 w2340 w2368 w2391 w2421 w2440 w2465 w2495 w2515 w2539 w2565 w2602 w2628 w2652 w2670 w2697 w2715 w2736 w2757 w2778 w2802 w2829 w2849 w2877 w2896 w2922 w2941 w2960 w2979 w2998 w3017 w3036 w3055] -> w1049
            tunnel: [w1104 w1123 w1142 w1165 w1225 w1308 w1355 w1407 w1442 w1477 w1542 w1572 w1596 w1620 w1650 w1685 w1716 w1741 w1767 w1793 w1831 w1852 w1883 w1904 w1923 w1942 w1961 w2007 w2042 w2067 w2096 w2117 w2136 w2155 w2174 w2207 w2252 w2271 w2303 w2339 w2367 w2390 w2420 w2439 w2464 w2494 w2514 w2538 w2564 w2601 w2627 w2651 w2669 w2696 w2714 w2735 w2756 w2777 w2801 w2828 w2848 w2876 w2895 w2921 w2940 w2959 w2978 w2997 w3016 w3035 w3054] -> w1050
            tunnel: [_ _ _ _ _ _ _ _ _ _ _ _ _ _ _ _ _ _ _ _ _ _ _ _ _ _ _ w1997 w2047 _ _ _ _ _ _ _ _ _ _ _ _ _ _ _ _ _ _ _ _ _ _ _ _ _ _ _ _ _ _ _ _ _ _ _ _ _ _ _ _ _ _] -> w1018
            tunnel: [_ _ _ _ _ _ _ _ _ _ _ _ _ _ _ _ _ _ _ _ _ _ _ _ _ _ _ w1996 w2046 _ _ _ _ _ _ _ _ _ _ _ _ _ _ _ _ _ _ _ _ _ _ _ _ _ _ _ _ _ _ _ _ _ _ _ _ _ _ _ _ _ _] -> w1017
            tunnel: w1031 -> [w1103 w1122 w1141 w1164 w1224 w1307 w1354 w1406 w1438 w1486 w1552 w1571 w1595 w1619 w1636 w1678 w1702 w1727 w1755 w1792 w1830 w1851 w1882 w1903 w1922 w1941 w1960 w1995 w2041 w2066 w2095 w2116 w2135 w2154 w2173 w2206 w2251 w2268 w2302 w2338 w2366 w2387 w2414 w2438 w2461 w2488 w2513 w2532 w2560 w2594 w2625 w2650 w2682 w2707 w2718 w2739 w2760 w2781 w2805 w2832 w2852 w2880 w2899 w2915 w2937 w2956 w2975 w2994 w3013 w3032 w3051]
            tunnel: [w1103 w1122 w1141 w1164 w1224 w1307 w1354 w1406 w1438 w1486 w1552 w1571 w1595 w1619 w1635 w1677 w1695 w1726 w1754 w1792 w1830 w1851 w1882 w1903 w1922 w1941 w1960 w1995 w2041 w2066 w2095 w2116 w2135 w2154 w2173 w2206 w2251 w2268 w2302 w2338 w2366 w2387 w2414 w2438 w2461 w2488 w2513 w2532 w2559 w2594 w2625 w2650 w2682 w2707 w2718 w2739 w2760 w2781 w2805 w2832 w2852 w2880 w2899 w2915 w2937 w2956 w2975 w2994 w3013 w3032 w3051] -> w1030
            tunnel: [w1102 w1121 w1140 w1163 w1223 w1306 w1353 w1405 w1437 w1485 w1551 w1570 w1606 w1618 w1656 w1684 w1715 w1740 w1766 w1791 w1829 w1850 w1881 w1902 w1921 w1940 w1959 w1994 w2040 w2065 w2094 w2115 w2134 w2153 w2172 w2205 w2250 w2267 w2301 w2337 w2365 w2386 w2413 w2437 w2460 w2487 w2512 w2531 w2552 w2600 w2624 w2648 w2683 w2693 w2713 w2734 w2755 w2776 w2800 w2836 w2856 w2883 w2903 w2928 w2947 w2966 w2985 w3004 w3023 w3042 w3061] -> w1029
            tunnel: [w1101 w1120 w1139 w1162 w1222 w1305 w1352 w1404 w1436 w1484 w1550 w1569 w1605 w1617 w1655 w1683 w1714 w1739 w1765 w1790 w1828 w1849 w1880 w1901 w1920 w1939 w1958 w1993 w2039 w2064 w2093 w2114 w2133 w2152 w2171 w2204 w2249 w2266 w2300 w2336 w2364 w2385 w2412 w2436 w2459 w2486 w2511 w2530 w2551 w2599 w2623 w2649 w2665 w2690 w2723 w2744 w2765 w2786 w2808 w2835 w2855 w2882 w2902 w2927 w2946 w2965 w2984 w3003 w3022 w3041 w3060] -> w1028
            tunnel: w1027 -> [w1102 w1121 w1140 w1163 w1223 w1306 w1353 w1405 w1437 w1485 w1551 w1570 w1606 w1618 w1656 w1684 w1715 w1740 w1766 w1791 w1829 w1850 w1881 w1902 w1921 w1940 w1959 w1994 w2040 w2065 w2094 w2115 w2134 w2153 w2172 w2205 w2250 w2267 w2301 w2337 w2365 w2386 w2413 w2437 w2460 w2487 w2512 w2531 w2552 w2600 w2624 w2648 _ w2693 w2713 w2734 w2755 w2776 w2800 w2836 w2856 w2883 w2903 w2928 w2947 w2966 w2985 w3004 w3023 w3042 w3061]
            tunnel: w1026 -> [w1101 w1120 w1139 w1162 w1222 w1305 w1352 w1404 w1436 w1484 w1550 w1569 w1605 w1617 w1655 w1683 w1714 w1739 w1765 w1790 w1828 w1849 w1880 w1901 w1920 w1939 w1958 w1993 w2039 w2064 w2093 w2114 w2133 w2152 w2171 w2204 w2249 w2266 w2300 w2336 w2364 w2385 w2412 w2436 w2459 w2486 w2511 w2530 w2551 w2599 w2623 w2649 _ w2690 w2723 w2744 w2765 w2786 w2808 w2835 w2855 w2882 w2902 w2927 w2946 w2965 w2984 w3003 w3022 w3041 w3060]
            tunnel: w1025 -> [_ _ _ _ _ _ _ _ _ _ _ _ _ _ _ _ _ _ _ _ _ _ _ _ _ _ _ _ _ _ _ _ _ _ _ _ _ _ _ _ _ _ _ _ _ _ _ _ _ _ _ _ _ _ w2711 w2732 w2753 w2774 w2798 _ _ _ _ _ _ _ _ _ _ _ _]
            tunnel: w1023 -> [_ _ _ _ _ _ _ _ _ _ _ _ _ _ _ _ w1707 _ w1750 w1779 w1815 w1841 w1872 _ _ _ _ w1975 w2020 w2058 w2087 _ _ _ _ _ _ _ _ _ _ _ _ _ _ _ _ _ _ _ _ _ _ _ _ _ _ _ _ _ _ _ _ _ _ _ _ _ _ _ _]
            tunnel: w1020 -> [_ _ _ _ _ _ _ _ _ _ _ _ _ _ _ _ _ _ _ _ _ _ _ _ _ _ _ _ _ _ _ _ _ _ _ _ _ _ _ _ _ _ _ _ _ _ _ _ _ _ _ _ _ _ _ _ _ _ _ _ _ w2870 _ _ _ _ _ _ _ _ _]
            tunnel: [w1100 w1119 w1138 w1161 w1221 w1304 w1351 w1403 w1435 w1483 w1549 w1564 w1589 w1613 w1657 w1682 w1713 w1738 w1764 w1789 w1827 w1848 w1879 w1900 w1919 w1938 w1957 w1992 w2038 w2063 w2092 w2113 w2132 w2151 w2170 w2200 w2248 w2265 w2299 w2321 w2363 w2384 w2411 w2435 w2458 w2485 w2510 w2529 w2550 w2597 w2610 w2647 w2668 w2692 w2710 w2731 w2752 w2773 w2795 w2815 w2844 w2864 w2891 w2911 w2936 w2955 w2974 w2993 w3012 w3031 w3050] -> w1014
            tunnel: w1015 -> [w1100 w1119 w1138 w1161 w1221 w1304 w1351 w1403 w1435 w1483 w1549 w1564 _ w1613 w1657 w1682 w1713 w1738 w1764 w1789 w1827 w1848 w1879 w1900 w1919 w1938 w1957 w1992 w2038 w2063 w2092 w2113 w2132 w2151 w2170 w2200 w2248 w2265 w2299 w2321 w2363 w2384 w2411 w2435 w2458 w2485 w2510 w2529 w2550 w2597 w2611 w2647 w2668 w2692 w2710 w2731 w2752 w2773 w2795 w2815 w2844 w2864 w2891 w2911 w2936 w2955 w2974 w2993 w3012 w3031 w3050]
            tunnel: w1013 -> [w1099 w1118 w1137 w1160 w1220 w1303 w1350 w1402 w1434 w1482 w1548 w1563 w1588 w1612 w1649 w1681 w1712 w1737 w1763 w1788 w1826 w1847 w1878 w1899 w1918 w1937 w1956 w1991 w2037 w2062 w2091 w2112 w2131 w2150 w2169 w2199 w2247 w2264 w2298 w2335 w2362 w2383 w2410 w2434 w2457 w2484 w2509 w2528 w2549 w2596 w2622 w2646 w2667 w2695 w2709 w2730 w2751 w2772 w2794 w2814 w2843 w2863 w2890 w2910 w2935 w2954 w2973 w2992 w3011 w3030 w3049]
            tunnel: w1012 -> [w1098 w1117 w1136 w1159 w1219 w1302 w1349 w1401 w1433 w1481 w1547 w1562 w1587 w1611 w1648 w1680 w1711 w1736 w1762 w1787 w1825 w1846 w1877 w1898 w1917 w1936 w1955 w1990 w2036 w2061 w2090 w2111 w2130 w2149 w2168 w2198 w2246 w2263 w2297 w2332 w2361 w2382 w2409 w2433 w2456 w2483 w2508 w2527 w2548 w2595 w2621 w2645 w2666 w2694 w2708 w2729 w2750 w2771 w2793 w2813 w2842 w2862 w2889 w2909 w2934 w2953 w2972 w2991 w3010 w3029 w3048]
            tunnel: [w1099 w1118 w1137 w1160 w1220 w1303 w1350 w1402 w1434 w1482 w1548 w1563 w1588 w1612 w1649 w1681 w1712 w1737 w1763 w1788 w1826 w1847 w1878 w1899 w1918 w1937 w1956 w1991 w2037 w2062 w2091 w2112 w2131 w2150 w2169 w2199 w2247 w2264 w2298 w2334 w2362 w2383 w2410 w2434 w2457 w2484 w2509 w2528 w2549 w2596 w2622 w2646 w2667 w2695 w2709 w2730 w2751 w2772 w2794 w2814 w2843 w2863 w2890 w2910 w2935 w2954 w2973 w2992 w3011 w3030 w3049] -> w1011
            tunnel: [w1098 w1117 w1136 w1159 w1219 w1302 w1349 w1401 w1433 w1481 w1547 w1562 w1587 w1611 w1648 w1680 w1711 w1736 w1762 w1787 w1825 w1846 w1877 w1898 w1917 w1936 w1955 w1990 w2036 w2061 w2090 w2111 w2130 w2149 w2168 w2198 w2246 w2263 w2297 w2333 w2361 w2382 w2409 w2433 w2456 w2483 w2508 w2527 w2548 w2595 w2621 w2645 w2666 w2694 w2708 w2729 w2750 w2771 w2793 w2813 w2842 w2862 w2889 w2909 w2934 w2953 w2972 w2991 w3010 w3029 w3048] -> w1010
            tunnel: w1009 -> [_ _ _ _ _ _ _ _ _ _ w1540 _ _ _ w1660 w1670 _ _ _ _ _ _ _ _ _ _ _ _ w2033 _ _ _ _ _ _ w2196 w2245 _ _ _ _ _ _ _ w2455 _ _ _ _ w2572 _ _ _ _ _ _ _ _ _ _ _ _ _ _ _ _ _ _ _ _ _]
            tunnel: w1008 -> [_ _ _ _ _ _ _ _ _ _ w1541 _ _ _ w1659 w1669 _ _ _ _ _ _ _ _ _ _ _ _ w2032 _ _ _ _ _ _ w2197 w2244 _ _ _ _ _ _ _ w2454 _ _ _ _ w2571 _ _ _ _ _ _ _ _ _ _ _ _ _ _ _ _ _ _ _ _ _]
            tunnel: w1006 -> [_ _ _ _ _ _ _ _ _ _ _ _ _ _ _ _ w1706 _ w1749 w1778 w1814 w1840 w1873 _ _ _ _ w1974 w2019 w2057 w2086 _ _ _ _ _ _ _ _ _ _ _ _ _ _ _ _ _ _ _ _ _ _ _ _ _ _ _ _ _ _ _ _ _ _ _ _ _ _ _ _]
            tunnel: [_ _ _ _ _ _ _ _ _ _ _ _ _ _ _ _ _ _ _ w1782 w1816 w1843 w1876 _ _ _ _ TRUE w2022 w2059 _ _ _ _ _ _ _ _ _ _ _ _ _ _ _ _ _ _ _ _ _ _ _ _ _ _ _ _ _ _ _ _ _ _ _ _ _ _ _ _ _] -> w1005
            tunnel: w1004 -> [_ _ _ _ _ _ _ _ _ _ _ _ _ _ _ _ w1705 _ _ w1781 w1820 w1845 w1874 _ _ _ _ w1982 w2027 w2056 w2089 _ _ _ _ _ _ _ _ _ _ _ _ _ _ _ _ _ _ _ _ _ _ _ _ _ _ _ _ _ _ _ _ _ _ _ _ _ _ _ _]
            tunnel: w1003 -> [_ _ _ _ _ _ _ _ _ _ _ _ _ _ _ _ w1704 _ _ w1780 w1819 w1844 w1875 _ _ _ _ w1981 w2026 w2055 w2088 _ _ _ _ _ _ _ _ _ _ _ _ _ _ _ _ _ _ _ _ _ _ _ _ _ _ _ _ _ _ _ _ _ _ _ _ _ _ _ _]
            tunnel: [_ _ _ _ _ _ _ _ _ _ _ _ _ _ _ _ w1705 _ w1752 w1781 w1820 w1845 w1874 _ _ _ _ w1982 w2027 w2056 w2089 _ _ _ _ _ _ _ _ _ _ _ _ _ _ _ _ _ _ _ _ _ _ _ _ _ _ _ _ _ _ _ _ _ _ _ _ _ _ _ _] -> w1002
            tunnel: [_ _ _ _ _ _ _ _ _ _ _ _ _ _ _ _ w1704 _ w1751 w1780 w1819 w1844 w1875 _ _ _ _ w1981 w2026 w2055 w2088 _ _ _ _ _ _ _ _ _ _ _ _ _ _ _ _ _ _ _ _ _ _ _ _ _ _ _ _ _ _ _ _ _ _ _ _ _ _ _ _] -> w1001
            tunnel: [_ _ _ _ _ _ _ _ _ _ _ _ _ _ _ _ w1707 w1730 w1750 w1779 w1815 w1841 w1872 _ _ _ _ w1975 w2020 w2058 w2087 _ _ _ _ _ _ _ _ _ _ _ _ _ _ _ _ _ _ _ _ _ _ _ _ _ _ _ _ _ _ _ _ _ _ _ _ _ _ _ _] -> w1000
            tunnel: [_ _ _ _ _ _ _ _ _ _ _ _ _ _ _ _ w1706 w1731 w1749 w1778 w1814 w1840 w1873 _ _ _ _ w1974 w2019 w2057 w2086 _ _ _ _ _ _ _ _ _ _ _ _ _ _ _ _ _ _ _ _ _ _ _ _ _ _ _ _ _ _ _ _ _ _ _ _ _ _ _ _] -> w999
            tunnel: [_ _ _ _ _ _ _ _ _ _ _ _ _ _ _ _ _ _ _ _ w1813 _ _ _ _ _ _ _ w2024 _ _ _ _ _ _ _ _ _ _ _ _ _ _ _ _ _ _ _ _ _ _ _ _ _ _ _ _ _ _ _ _ _ _ _ _ _ _ _ _ _ _] -> w996
            tunnel: [_ _ _ _ _ _ _ _ _ _ _ _ _ _ _ _ _ _ _ _ w1812 _ _ _ _ _ _ _ w2025 _ _ _ _ _ _ _ _ _ _ _ _ _ _ _ _ _ _ _ _ _ _ _ _ _ _ _ _ _ _ _ _ _ _ _ _ _ _ _ _ _ _] -> w998
            tunnel: w993 -> [_ _ _ _ _ _ _ _ _ _ _ _ _ _ _ _ _ _ _ w1777 w1811 w1842 w1871 _ _ _ _ w1977 w2021 w2060 _ _ _ _ _ _ _ _ _ _ _ _ _ _ _ _ _ _ _ _ _ _ _ _ _ _ _ _ _ _ _ _ _ _ _ _ _ _ _ _ _]
            tunnel: [_ _ _ _ _ _ _ _ _ _ _ _ _ _ _ _ _ _ _ w1777 w1811 w1842 w1871 _ _ _ _ w1977 w2023 w2060 _ _ _ _ _ _ _ _ _ _ _ _ _ _ _ _ _ _ _ _ _ _ _ _ _ _ _ _ _ _ _ _ _ _ _ _ _ _ _ _ _] -> w992
            frame "Start1", Default {
            }
            frame "Start2" {
            }
            frame "Start3" {
            }
            frame "saveSettings1" {
              n596 = call "myRIO_BRig_RT_dataExp_Audio_freq__L.vi"() -> ("output_Audio_freq__L"=w1184:i32)  [unwired: 11 in]
              n597 = call "myRIO_BRig_RT_dataExp_Audio_freq__R.vi"() -> ("output_Audio_freq__R"=w1183:i32)  [unwired: 11 in]
              n598 = call "myRIO_BRig_RT_dataExp_Audio_amp__L.vi"() -> ("output_Audio_amp__L"=w1182:i32)  [unwired: 11 in]
              n599 = call "myRIO_BRig_RT_dataExp_Audio_amp__R.vi"() -> ("output_Audio_amp__R"=w1180:i32)  [unwired: 11 in]
              n600 = call "myRIO_BRig_RT_dataExp_TPB_min__L.vi"() -> ("output_TPB_min__L"=w1192:i32)  [unwired: 11 in]
              n601 = call "myRIO_BRig_RT_dataExp_TPB_min__R.vi"() -> ("output_TPB_min__R"=w1190:i32)  [unwired: 11 in]
              n602 = call "myRIO_BRig_RT_dataExp_TPB_max__L.vi"() -> ("output_TPB_max__L"=w1188:i32)  [unwired: 11 in]
              n603 = call "myRIO_BRig_RT_dataExp_TPB_max__R.vi"() -> ("output_TPB_max__R"=w1186:i32)  [unwired: 11 in]
              n604 = call "myRIO_BRig_RT_dataExp_ItrialUntilReward.vi"() -> ("output_I_trialUntilReward"=w1205:i32)  [unwired: 11 in]
              n605 = call "myRIO_BRig_RT_dataExp_IblockUntilReward.vi"() -> ("output_I_blockUntilReward"=w1201:i32)  [unwired: 11 in]
              n606 = call "myRIO_BRig_RT_dataExp_CueCycles.vi"() -> ("output_CueCycles"=w1200:i32)  [unwired: 11 in]
              n607 = call "myRIO_BRig_RT_dataExp_ENL_min.vi"() -> ("output_ENL_min"=w1198:i32)  [unwired: 11 in]
              n608 = call "myRIO_BRig_RT_dataExp_ENL_max.vi"() -> ("output_ENL_max"=w1196:i32)  [unwired: 11 in]
              n609 = call "myRIO_BRig_RT_dataExp_ENL_penalty.vi"() -> ("output_ENL_penalty"=w1194:i32)  [unwired: 11 in]
              n610 = local read "Audio_Freq__L"() -> (w1158:u8)
              n611 = local read "Audio_Freq__R"() -> (w1156:u8)
              n612 = local read "Audio_Amp__L"() -> (w1181:u16)
              n613 = local read "TpB_Min_L"() -> (w1191:u16)
              n614 = local read "TpB_Min_R"() -> (w1189:u16)
              n615 = local read "TpB_Max_L"() -> (w1187:u16)
              n616 = local read "TpB_Max_R"() -> (w1185:u16)
              n617 = local read "Audio_Amp__R"() -> (w1179:u16)
              n618 = local read "TrialUntilReward"() -> (w1204:bool)
              n619 = local read "CueCycles"() -> (w1199:u16)
              n620 = local read "Tcycle_ENL_min"() -> (w1197:u16)
              n621 = local read "Tcycle_ENL_max"() -> (w1195:u16)
              n622 = local read "Tcycle_ENLPenalty"() -> (w1193:u16)
              n623 = To Unsigned Word Integer(number=w1156) -> (unsigned 16bit integer=w1155:u16)
              n624 = To Unsigned Word Integer(number=w1158) -> (unsigned 16bit integer=w1157:u16)
              n625 = Boolean To (0,1)(Boolean=w1204) -> (0, 1=w1203:i16)
              n626 = To Unsigned Word Integer(number=w1203) -> (unsigned 16bit integer=w1202:u16)
              n627 = local read "BUR_min"() -> (w1173:u16)
              n628 = local read "BUR_max"() -> (w1174:u16)
              n629 = Not Equal To 0?(x=w1173) -> (x != 0?=w1172:bool)
              n630 = Not Equal To 0?(x=w1174) -> (x != 0?=w1171:bool)
              n631 = And(x=w1172, y=w1171) -> (x .and. y?=w1170:bool)
              n632 = Boolean To (0,1)(Boolean=w1170) -> (0, 1=w1175:i16)
              n633 = To Unsigned Word Integer(number=w1175) -> (unsigned 16bit integer=w1169:u16)
              n634 = Replace Array Subset(array=w1207, new element #1=w1202, index #1=w1205, new element #2=w1169, index #2=w1201, new element #3=w1199, index #3=w1200, new element #4=w1197, index #4=w1198, new element #5=w1195, index #5=w1196, new element #6=w1193, index #6=w1194, new element #7=w1191, index #7=w1192, new element #8=w1189, index #8=w1190, new element #9=w1187, index #9=w1188, new element #10=w1185, index #10=w1186, new element #11=w1157, index #11=w1184, new element #12=w1155, index #12=w1183, new element #13=w1181, index #13=w1182, new element #14=w1179, index #14=w1180) -> (w1206:u16[])
            }
            frame "saveSettings2" {
              n635 = call "myRIO_BRig_RT_dataExp_Tcycle_RewardPost.vi"() -> ("output_Tcycle_RewardPost"=w1244:i32)  [unwired: 11 in]
              n636 = call "myRIO_BRig_RT_dataExp_Tcycle_Wrong.vi"() -> ("output_Tcycle_Wrong"=w1242:i32)  [unwired: 11 in]
              n637 = call "myRIO_BRig_RT_dataExp_Tcycle_Timeout.vi"() -> ("output_Tcycle_Timeout"=w1240:i32)  [unwired: 11 in]
              n638 = call "myRIO_BRig_RT_dataExp_Tcycle_Cue_min.vi"() -> ("output_Tcycle_Cue_min"=w1238:i32)  [unwired: 11 in]
              n639 = call "myRIO_BRig_RT_dataExp_Tcycle_Cue_max.vi"() -> ("output_Tcycle_Cue_max"=w1237:i32)  [unwired: 11 in]
              n640 = call "myRIO_BRig_RT_dataExp_Tcycle_CuePenalty.vi"() -> ("output_Tcycle_CuePenalty"=w1236:i32)  [unwired: 11 in]
              n641 = call "myRIO_BRig_RT_dataExp_SolenoidProbability_L.vi"() -> ("output_SolenoidProbability_L"=w1216:i32)  [unwired: 11 in]
              n642 = call "myRIO_BRig_RT_dataExp_SolenoidProbability_R.vi"() -> ("output_SolenoidProbability_R"=w1215:i32)  [unwired: 11 in]
              n643 = call "myRIO_BRig_RT_dataExp_nBlock.vi"() -> ("output_nBlock"=w1253:i32)  [unwired: 11 in]
              n644 = call "myRIO_BRig_RT_dataExp_nTrial.vi"() -> ("output_nTrial"=w1252:i32)  [unwired: 11 in]
              n645 = call "myRIO_BRig_RT_dataExp_runTime_seconds.vi"() -> ("output_RunTime_minutes"=w1251:i32)  [unwired: 11 in]
              n646 = call "myRIO_BRig_RT_dataExp_Tcycle_Selection.vi"() -> ("output_Tcycle_Selection"=w1250:i32)  [unwired: 11 in]
              n647 = call "myRIO_BRig_RT_dataExp_Tcycle_Reward__L.vi"() -> ("output_Tcycle_Reward__L"=w1248:i32)  [unwired: 11 in]
              n648 = call "myRIO_BRig_RT_dataExp_Tcycle_Reward__R.vi"() -> ("output_Tcycle_Reward__R"=w1246:i32)  [unwired: 11 in]
              n649 = local read "Tcycle_RewardPost"() -> (w1243:u16)
              n650 = local read "Tcycle_Wrong"() -> (w1241:u16)
              n651 = local read "Tcycle_Timeout"() -> (w1239:u16)
              n652 = local read "Tcycle_CuePenalty"() -> (w1229:u16)
              n653 = local read "Tcycle_Cue_max"() -> (w1217:u16)
              n654 = local read "Tcycle_Cue_min"() -> (w1218:u16)
              n655 = local read "Tcycle_Selection"() -> (w1249:u16)
              n656 = local read "Tcycle_Reward_L"() -> (w1247:u16)
              n657 = local read "Tcycle_Reward_R"() -> (w1245:u16)
              n658 = local read "SolenoidProbability_R"() -> (w1213:u16)
              n659 = local read "SolenoidProbability_L"() -> (w1214:u16)
              n660 = Replace Array Subset(array=w1255, new element #1=u16 0, index #1=w1253, new element #2=u16 0, index #2=w1252, new element #3=u16 0, index #3=w1251, new element #4=w1249, index #4=w1250, new element #5=w1247, index #5=w1248, new element #6=w1245, index #6=w1246, new element #7=w1243, index #7=w1244, new element #8=w1241, index #8=w1242, new element #9=w1239, index #9=w1240, new element #10=w1218, index #10=w1238, new element #11=w1217, index #11=w1237, new element #12=w1229, index #12=w1236, new element #13=w1214, index #13=w1216, new element #14=w1213, index #14=w1215) -> (w1254:u16[])
            }
            frame "saveSettings3" {
              w1265 = 100.0 ("y")
              n661 = call "myRIO_BRig_RT_dataExp_laser_Freq.vi"() -> ("output_laser_Freq"=w1298:i32)  [unwired: 11 in]
              n662 = call "myRIO_BRig_RT_dataExp_laser_Tpeak.vi"() -> ("output_laser_Tpeak"=w1293:i32)  [unwired: 11 in]
              n663 = call "myRIO_BRig_RT_dataExp_laser_Tshutter.vi"() -> ("output_laser_Tshutter"=w1288:i32)  [unwired: 11 in]
              n664 = call "myRIO_BRig_RT_dataExp_laser_f_millisec2count.vi"() -> ("output_laser_f_millisec2count"=w1283:i32)  [unwired: 11 in]
              n665 = call "myRIO_BRig_RT_dataExp_laser_Power_min.vi"() -> ("output_laser_Power_min"=w1278:i32)  [unwired: 11 in]
              n666 = call "myRIO_BRig_RT_dataExp_laser_Power_max.vi"() -> ("output_laser_Power_max"=w1271:i32)  [unwired: 11 in]
              n667 = call "myRIO_BRig_RT_dataExp_laser_Power_step.vi"() -> ("output_laser_Power_step"=w1270:i32)  [unwired: 11 in]
              n668 = call "myRIO_BRig_RT_dataExp_laser_duration.vi"() -> ("output_laser_duration"=w1273:i32)  [unwired: 11 in]
              n669 = call "myRIO_BRig_RT_dataExp_BUR_min.vi"() -> ("output_BUR_min"=w1320:i32)  [unwired: 11 in]
              n670 = call "myRIO_BRig_RT_dataExp_BUR_max.vi"() -> ("output_BUR_max"=w1318:i32)  [unwired: 11 in]
              n671 = call "myRIO_BRig_RT_dataExp_Audio_sp__L.vi"() -> ("output_Audio_sp__L"=w1315:i32)  [unwired: 11 in]
              n672 = call "myRIO_BRig_RT_dataExp_Audio_sp__R.vi"() -> ("output_Audio_sp__R"=w1314:i32)  [unwired: 11 in]
              n673 = local read "laser_Tshutter"() -> (w1285:dbl)
              n674 = local read "f_millisec2count"() -> (w1280:dbl)
              n675 = local read "laser_Tpeak"() -> (w1290:dbl)
              n676 = local read "laser_power_min"() -> (w1275:dbl)
              n677 = local read "laser_power_max"() -> (w1264:dbl)
              n678 = local read "laser_power_step"() -> (w1263:dbl)
              n679 = local read "laser_Freq"() -> (w1297:dbl)
              n680 = local read "sp_LeftSpout"() -> (w1313:u16)
              n681 = local read "BUR_max"() -> (w1317:u16)
              n682 = local read "sp_RightSpout"() -> (w1312:u16)
              n683 = local read "BUR_min"() -> (w1319:u16)
              n684 = Multiply(x=w1297, y=w1265) -> (x*y=w1296:dbl)
              n685 = Multiply(x=w1290, y=w1265) -> (x*y=w1292:dbl)
              n686 = Multiply(x=w1285, y=w1265) -> (x*y=w1287:dbl)
              n687 = Multiply(x=w1280, y=w1265) -> (x*y=w1282:dbl)
              n688 = Multiply(x=w1275, y=w1265) -> (x*y=w1277:dbl)
              n689 = Multiply(x=w1264, y=w1265) -> (x*y=w1269:dbl)
              n690 = Multiply(x=w1263, y=w1265) -> (x*y=w1267:dbl)
              n691 = Round To Nearest(number=w1296) -> (nearest integer value=w1295:dbl)
              n692 = Round To Nearest(number=w1292) -> (nearest integer value=w1291:dbl)
              n693 = Round To Nearest(number=w1287) -> (nearest integer value=w1286:dbl)
              n694 = Round To Nearest(number=w1282) -> (nearest integer value=w1281:dbl)
              n695 = Round To Nearest(number=w1277) -> (nearest integer value=w1276:dbl)
              n696 = Round To Nearest(number=w1269) -> (nearest integer value=w1268:dbl)
              n697 = Round To Nearest(number=w1267) -> (nearest integer value=w1266:dbl)
              n698 = To Unsigned Word Integer(number=w1295) -> (unsigned 16bit integer=w1294:u16)
              n699 = To Unsigned Word Integer(number=w1291) -> (unsigned 16bit integer=w1289:u16)
              n700 = To Unsigned Word Integer(number=w1286) -> (unsigned 16bit integer=w1284:u16)
              n701 = To Unsigned Word Integer(number=w1281) -> (unsigned 16bit integer=w1279:u16)
              n702 = To Unsigned Word Integer(number=w1276) -> (unsigned 16bit integer=w1274:u16)
              n703 = To Unsigned Word Integer(number=w1268) -> (unsigned 16bit integer=w1262:u16)
              n704 = To Unsigned Word Integer(number=w1266) -> (unsigned 16bit integer=w1261:u16)
              n705 = local read "laser_duration"() -> (w1272:u16)
              n706 = call "myRIO_BRig_RT_dataCurrent_LaserPulse_duration.vi"() -> ("output_LaserPulse_duration"=w1299:i32)  [unwired: 11 in]
              n707 = Replace Array Subset(array=w1321, new element #1=w1319, index #1=w1320, new element #2=w1317, index #2=w1318, new element #3=w1313, index #3=w1315, new element #4=w1312, index #4=w1314, new element #5=w1294, index #5=w1298, new element #6=w1289, index #6=w1293, new element #7=w1284, index #7=w1288, new element #8=w1279, index #8=w1283, new element #9=w1274, index #9=w1278, new element #10=w1262, index #10=w1271, new element #11=w1261, index #11=w1270, new element #12=w1272, index #12=w1273) -> (w1316:u16[])
              n708 = Replace Array Subset(array=w1301, new element=w1272, index=w1299) -> (w1300:u16[])
            }
            frame "saveSettings4_LC_ENL" {
              # "delayOpt"
              # "Count"
              # "Tdelay"
              # "Probability"
              # "OnOff"
              # "Block"
              # "ENL1 All"
              # "delayOpt"
              # "Count"
              # "Tdelay"
              # "Probability"
              # "OnOff"
              # "Block"
              # "ENL1 First"
              n709 = call "myRIO_BRig_RT_dataLC_ENL1_All_Block.vi"() -> ("output_ENL1_All_Block"=w1344:i32)  [unwired: 11 in]
              n710 = call "myRIO_BRig_RT_dataLC_ENL1_All_OnOff.vi"() -> ("output_ENL1_All_OnOff"=w1333:i32)  [unwired: 11 in]
              n711 = call "myRIO_BRig_RT_dataLC_ENL1_All_Probability.vi"() -> ("output_ENL1_All_Probability"=w1332:i32)  [unwired: 11 in]
              n712 = call "myRIO_BRig_RT_dataLC_ENL1_All_Tdelay.vi"() -> ("output_ENL1_All_Tdelay"=w1331:i32)  [unwired: 11 in]
              n713 = call "myRIO_BRig_RT_dataLC_ENL1_All_Count.vi"() -> ("output_ENL1_All_Count"=w1330:i32)  [unwired: 11 in]
              n714 = call "myRIO_BRig_RT_dataLC_ENL1_All_delayOpt.vi"() -> ("output_ENL1_All_delayOpt"=w1329:i32)  [unwired: 11 in]
              n715 = call "myRIO_BRig_RT_dataLC_ENL1_First_Block.vi"() -> ("output_ENL1_First_Block"=w1370:i32)  [unwired: 11 in]
              n716 = call "myRIO_BRig_RT_dataLC_ENL1_First_OnOff.vi"() -> ("output_ENL1_First_OnOff"=w1368:i32)  [unwired: 11 in]
              n717 = call "myRIO_BRig_RT_dataLC_ENL1_First_Probability.vi"() -> ("output_ENL1_First_Probability"=w1364:i32)  [unwired: 11 in]
              n718 = call "myRIO_BRig_RT_dataLC_ENL1_First_Tdelay.vi"() -> ("output_ENL1_First_Tdelay"=w1362:i32)  [unwired: 11 in]
              n719 = call "myRIO_BRig_RT_dataLC_ENL1_First_Count.vi"() -> ("output_ENL1_First_Count"=w1360:i32)  [unwired: 11 in]
              n720 = call "myRIO_BRig_RT_dataLC_ENL1_First_delayOpt.vi"() -> ("output_ENL1_First_delayOpt"=w1346:i32)  [unwired: 11 in]
              n721 = local read "LC_ENL1_First_delayOpt"() -> (w1347:bool)
              n722 = local read "LC_ENL1_First_Count"() -> (w1359:u16)
              n723 = local read "LC_ENL1_First_Probability"() -> (w1363:u16)
              n724 = local read "LC_ENL1_First_Block"() -> (w1369:u16)
              n725 = local read "LC_ENL1_First_Tdelay"() -> (w1361:u16)
              n726 = local read "LC_ENL1_First_OnOff"() -> (w1367:bool)
              n727 = local read "LC_ENL1_All_OnOff"() -> (w1340:bool)
              n728 = local read "LC_ENL1_All_Probability"() -> (w1338:u16)
              n729 = local read "LC_ENL1_All_delayOpt"() -> (w1335:bool)
              n730 = local read "LC_ENL1_All_Tdelay"() -> (w1337:u16)
              n731 = local read "LC_ENL1_All_Block"() -> (w1341:u16)
              n732 = local read "LC_ENL1_All_Count"() -> (w1336:u16)
              n733 = Boolean To (0,1)(Boolean=w1347) -> (0, 1=w1348:i16)
              n734 = Boolean To (0,1)(Boolean=w1367) -> (0, 1=w1366:i16)
              n735 = Boolean To (0,1)(Boolean=w1340) -> (0, 1=w1343:i16)
              n736 = To Unsigned Word Integer(number=w1348) -> (unsigned 16bit integer=w1345:u16)
              n737 = To Unsigned Word Integer(number=w1366) -> (unsigned 16bit integer=w1365:u16)
              n738 = Boolean To (0,1)(Boolean=w1335) -> (0, 1=w1342:i16)
              n739 = To Unsigned Word Integer(number=w1343) -> (unsigned 16bit integer=w1339:u16)
              n740 = To Unsigned Word Integer(number=w1342) -> (unsigned 16bit integer=w1334:u16)
              n741 = Replace Array Subset(array=w1371, new element #1=w1369, index #1=w1370, new element #2=w1365, index #2=w1368, new element #3=w1363, index #3=w1364, new element #4=w1361, index #4=w1362, new element #5=w1359, index #5=w1360, new element #6=w1345, index #6=w1346, new element #7=w1341, index #7=w1344, new element #8=w1339, index #8=w1333, new element #9=w1338, index #9=w1332, new element #10=w1337, index #10=w1331, new element #11=w1336, index #11=w1330, new element #12=w1334, index #12=w1329) -> (w1372:u16[])
            }
            frame "saveSettings5_LC_Cue" {
              # "delayOpt"
              # "Count"
              # "Tdelay"
              # "Probability"
              # "OnOff"
              # "Block"
              # "Cue1 All"
              # "delayOpt"
              # "Count"
              # "Tdelay"
              # "Probability"
              # "OnOff"
              # "Block"
              # "Cue1 First"
              n742 = call "myRIO_BRig_RT_dataLC_Cue1_First_delayOpt.vi"() -> ("output_Cue1_First_delayOpt"=w1399:i32)  [unwired: 11 in]
              n743 = call "myRIO_BRig_RT_dataLC_Cue1_First_Block.vi"() -> ("output_Cue1_First_Block"=w1422:i32)  [unwired: 11 in]
              n744 = call "myRIO_BRig_RT_dataLC_Cue1_First_OnOff.vi"() -> ("output_Cue1_First_OnOff"=w1420:i32)  [unwired: 11 in]
              n745 = call "myRIO_BRig_RT_dataLC_Cue1_First_Probability.vi"() -> ("output_Cue1_First_Probability"=w1416:i32)  [unwired: 11 in]
              n746 = call "myRIO_BRig_RT_dataLC_Cue1_First_Tdelay.vi"() -> ("output_Cue1_First_Tdelay"=w1414:i32)  [unwired: 11 in]
              n747 = call "myRIO_BRig_RT_dataLC_Cue1_First_Count.vi"() -> ("output_Cue1_First_Count"=w1412:i32)  [unwired: 11 in]
              n748 = call "myRIO_BRig_RT_dataLC_Cue1_All_Block.vi"() -> ("output_Cue1_All_Block"=w1396:i32)  [unwired: 11 in]
              n749 = call "myRIO_BRig_RT_dataLC_Cue1_All_OnOff.vi"() -> ("output_Cue1_All_OnOff"=w1395:i32)  [unwired: 11 in]
              n750 = call "myRIO_BRig_RT_dataLC_Cue1_All_Probability.vi"() -> ("output_Cue1_All_Probability"=w1394:i32)  [unwired: 11 in]
              n751 = call "myRIO_BRig_RT_dataLC_Cue1_All_Tdelay.vi"() -> ("output_Cue1_All_Tdelay"=w1393:i32)  [unwired: 11 in]
              n752 = call "myRIO_BRig_RT_dataLC_Cue1_All_Count.vi"() -> ("output_Cue1_All_Count"=w1392:i32)  [unwired: 11 in]
              n753 = call "myRIO_BRig_RT_dataLC_Cue1_All_delayOpt.vi"() -> ("output_Cue1_All_delayOpt"=w1391:i32)  [unwired: 11 in]
              n754 = local read "LC_Cue1_First_delayOpt"() -> (w1398:bool)
              n755 = local read "LC_Cue1_First_Count"() -> (w1411:u16)
              n756 = local read "LC_Cue1_First_Probability"() -> (w1415:u16)
              n757 = local read "LC_Cue1_First_Block"() -> (w1421:u16)
              n758 = local read "LC_Cue1_First_Tdelay"() -> (w1413:u16)
              n759 = local read "LC_Cue1_First_OnOff"() -> (w1419:bool)
              n760 = local read "LC_Cue1_All_OnOff"() -> (w1387:bool)
              n761 = local read "LC_Cue1_All_delayOpt"() -> (w1388:bool)
              n762 = local read "LC_Cue1_All_Probability"() -> (w1384:u16)
              n763 = local read "LC_Cue1_All_Tdelay"() -> (w1383:u16)
              n764 = local read "LC_Cue1_All_Count"() -> (w1382:u16)
              n765 = local read "LC_Cue1_All_Block"() -> (w1386:u16)
              n766 = Boolean To (0,1)(Boolean=w1398) -> (0, 1=w1400:i16)
              n767 = Boolean To (0,1)(Boolean=w1419) -> (0, 1=w1418:i16)
              n768 = Boolean To (0,1)(Boolean=w1387) -> (0, 1=w1390:i16)
              n769 = To Unsigned Word Integer(number=w1400) -> (unsigned 16bit integer=w1397:u16)
              n770 = To Unsigned Word Integer(number=w1418) -> (unsigned 16bit integer=w1417:u16)
              n771 = To Unsigned Word Integer(number=w1390) -> (unsigned 16bit integer=w1385:u16)
              n772 = Boolean To (0,1)(Boolean=w1388) -> (0, 1=w1389:i16)
              n773 = To Unsigned Word Integer(number=w1389) -> (unsigned 16bit integer=w1381:u16)
              n774 = Replace Array Subset(array=w1423, new element #1=w1421, index #1=w1422, new element #2=w1417, index #2=w1420, new element #3=w1415, index #3=w1416, new element #4=w1413, index #4=w1414, new element #5=w1411, index #5=w1412, new element #6=w1397, index #6=w1399, new element #7=w1386, index #7=w1396, new element #8=w1385, index #8=w1395, new element #9=w1384, index #9=w1394, new element #10=w1383, index #10=w1393, new element #11=w1382, index #11=w1392, new element #12=w1381, index #12=w1391) -> (w1424:u16[])
            }
            frame "saveSettings6_LC_Other" {
              # "Trial"
              # "Tdelay"
              # "Probability"
              # "OnOff"
              # "Block"
              # "Wrong"
              # "Trial"
              # "Tdelay"
              # "Probability"
              # "OnOff"
              # "Block"
              # "Reward"
              n775 = call "myRIO_BRig_RT_dataLC_Wrong_Block.vi"() -> ("output_Wrong_Block"=w1454:i32)  [unwired: 11 in]
              n776 = call "myRIO_BRig_RT_dataLC_Wrong_OnOff.vi"() -> ("output_Wrong_OnOff"=w1453:i32)  [unwired: 11 in]
              n777 = call "myRIO_BRig_RT_dataLC_Wrong_Probability.vi"() -> ("output_Wrong_Probability"=w1452:i32)  [unwired: 11 in]
              n778 = call "myRIO_BRig_RT_dataLC_Wrong_Tdelay.vi"() -> ("output_Wrong_Tdelay"=w1451:i32)  [unwired: 11 in]
              n779 = call "myRIO_BRig_RT_dataLC_Wrong_Trial.vi"() -> ("output_Wrong_Trial"=w1450:i32)  [unwired: 11 in]
              n780 = call "myRIO_BRig_RT_dataLC_Reward_Block.vi"() -> ("output_Reward_Block"=w1466:i32)  [unwired: 11 in]
              n781 = call "myRIO_BRig_RT_dataLC_Reward_OnOff.vi"() -> ("output_Reward_OnOff"=w1464:i32)  [unwired: 11 in]
              n782 = call "myRIO_BRig_RT_dataLC_Reward_Probability.vi"() -> ("output_Reward_Probability"=w1460:i32)  [unwired: 11 in]
              n783 = call "myRIO_BRig_RT_dataLC_Reward_Tdelay.vi"() -> ("output_Reward_Tdelay"=w1458:i32)  [unwired: 11 in]
              n784 = call "myRIO_BRig_RT_dataLC_Reward_Trial.vi"() -> ("output_Reward_Trial"=w1456:i32)  [unwired: 11 in]
              n785 = local read "LC_Wrong_OnOff"() -> (w1448:bool)
              n786 = local read "LC_Wrong_Probability"() -> (w1445:u16)
              n787 = local read "LC_Wrong_Block"() -> (w1447:u16)
              n788 = local read "LC_Wrong_Tdelay"() -> (w1444:u16)
              n789 = local read "LC_Wrong_Trial"() -> (w1443:u16)
              n790 = local read "LC_Reward_Probability"() -> (w1459:u16)
              n791 = local read "LC_Reward_Block"() -> (w1465:u16)
              n792 = local read "LC_Reward_Tdelay"() -> (w1457:u16)
              n793 = local read "LC_Reward_OnOff"() -> (w1463:bool)
              n794 = local read "LC_Reward_Trial"() -> (w1455:u16)
              n795 = Boolean To (0,1)(Boolean=w1448) -> (0, 1=w1449:i16)
              n796 = Boolean To (0,1)(Boolean=w1463) -> (0, 1=w1462:i16)
              n797 = To Unsigned Word Integer(number=w1449) -> (unsigned 16bit integer=w1446:u16)
              n798 = To Unsigned Word Integer(number=w1462) -> (unsigned 16bit integer=w1461:u16)
              n799 = Replace Array Subset(array=w1467, new element #1=w1465, index #1=w1466, new element #2=w1461, index #2=w1464, new element #3=w1459, index #3=w1460, new element #4=w1457, index #4=w1458, new element #5=w1455, index #5=w1456, new element #6=w1447, index #6=w1454, new element #7=w1446, index #7=w1453, new element #8=w1445, index #8=w1452, new element #9=w1444, index #9=w1451, new element #10=w1443, index #10=w1450) -> (w1468:u16[])
            }
            frame "setSettings_Audio" {
              # "amp_L"
              # "amp_R"
              # "freq_L"
              # "freq_R"
              n800 = call "myRIO_BRig_RT_dataExp_Audio_amp__L.vi"() -> ("output_Audio_amp__L"=w1493:i32)  [unwired: 11 in]
              n801 = call "myRIO_BRig_RT_dataExp_Audio_amp__R.vi"() -> ("output_Audio_amp__R"=w1492:i32)  [unwired: 11 in]
              n802 = call "myRIO_BRig_RT_dataExp_Audio_freq__L.vi"() -> ("output_Audio_freq__L"=w1491:i32)  [unwired: 11 in]
              n803 = call "myRIO_BRig_RT_dataExp_Audio_freq__R.vi"() -> ("output_Audio_freq__R"=w1490:i32)  [unwired: 11 in]
              n804 = Index Array(array=w1489, index #1=w1493, index #2=w1492, index #3=w1491, index #4=w1490) -> (element #1=w1488:u16, element #2=w1487:u16, element #3=w1480:u16, element #4=w1478:u16)
              n805 = To Unsigned Byte Integer(number=w1480) -> (unsigned 8bit integer=w1479:u8)
              n806 = To Unsigned Byte Integer(number=w1478) -> (unsigned 8bit integer=w1477:u8)
            }
            frame "setSettings_Laser" {
              (unwired) u32 0 ("tDelay_laser_rew")
              # "Wrong tDelay"
              # "Reward tDelay"
              n807 = call "myRIO_BRig_RT_dataLC_Reward_Tdelay.vi"() -> ("output_Reward_Tdelay"=w1520:i32)  [unwired: 11 in]
              n808 = call "myRIO_BRig_RT_dataLC_Wrong_Tdelay.vi"() -> ("output_Wrong_Tdelay"=w1521:i32)  [unwired: 11 in]
              n809 = Index Array(array=w1517, index #1=w1520, index #2=w1521) -> (element #1=w1519:u16, element #2=w1518:u16)
              n810 = call "myRIO_BRig_RT__calc_Tvalley.vi"("input_peakWidth"="laser_Tpeak", "input_freq"="laser_Freq") -> ("output_Tvalley"=w1527:dbl)  [unwired: 9 in]
              n811 = To Double Precision Float(number=w1519) -> (double precision float=w1514:dbl)
              n812 = To Double Precision Float(number=w1518) -> (double precision float=w1511:dbl)
              n813 = Multiply(x="f_millisec2count", y="laser_Tpeak") -> (x*y=w1536:dbl)
              n814 = Multiply(x="f_millisec2count", y=w1527) -> (x*y=w1533:dbl)
              n815 = Multiply(x="f_millisec2count", y="laser_Tshutter") -> (x*y=w1531:dbl)
              n816 = Round Toward +Infinity(x="laser_Tshutter") -> (ceil(x): smallest int >= x=w1522:dbl)
              n817 = Multiply(x="f_millisec2count", y=w1514) -> (x*y=w1515:dbl)
              n818 = Multiply(x="f_millisec2count", y=w1511) -> (x*y=w1512:dbl)
              n819 = To Unsigned Word Integer(number="f_millisec2count") -> (unsigned 16bit integer=w1502:u16)
              n820 = Round Toward +Infinity(x=w1536) -> (ceil(x): smallest int >= x=w1537:dbl)
              n821 = Round Toward +Infinity(x=w1533) -> (ceil(x): smallest int >= x=w1534:dbl)
              n822 = Round Toward +Infinity(x=w1531) -> (ceil(x): smallest int >= x=w1526:dbl)
              n823 = Round Toward +Infinity(x=w1515) -> (ceil(x): smallest int >= x=w1516:dbl)
              n824 = Round Toward +Infinity(x=w1512) -> (ceil(x): smallest int >= x=w1513:dbl)
              n825 = To Unsigned Long Integer(number=w1537) -> (unsigned 32bit integer=w1535:u32)
              n826 = To Unsigned Long Integer(number=w1534) -> (unsigned 32bit integer=w1532:u32)
              n827 = To Unsigned Long Integer(number=w1526) -> (unsigned 32bit integer=w1530:u32)
              n828 = To Unsigned Word Integer(number=w1522) -> (unsigned 16bit integer=w1525:u16)
              n829 = To Unsigned Long Integer(number=w1516) -> (unsigned 32bit integer=w1510:u32)
              n830 = To Unsigned Long Integer(number=w1513) -> (unsigned 32bit integer=w1509:u32)
              n831 = Add(x="laser_duration", y=w1525) -> (x+y=w1506:u16)
              n832 = To Double Precision Float(number=w1506) -> (double precision float=w1505:dbl)
              n833 = Multiply(x=w1505, y="f_millisec2count") -> (x*y=w1507:dbl)
              n834 = call "myRIO_BRig_RT_dataCurrent_LaserPulse_duration.vi"() -> ("output_LaserPulse_duration"=w1538:i32)  [unwired: 11 in]
              n835 = Round Toward +Infinity(x=w1507) -> (ceil(x): smallest int >= x=w1508:dbl)
              n836 = To Unsigned Long Integer(number=w1508) -> (unsigned 32bit integer=w1504:u32)
              n837 = xnode "Read/Write Control"("FPGA VI Reference In"=w1540, "error in"=w1541, "laser_Npeak"=w1535, "laser_Nvalley"=w1532, "laser_Nshutter"=w1530, "laser_selRew_Ndelay"=w1510, "laser_selWro_NDelay"=w1509, "laser_selRew_Ntotal"=w1504, "laser_selWro_Ntotal"=w1504, "k1__counter_per_ms"=w1502) -> ("error out"=→"error out":errorcluster)  [unwired: 1 out]
              n838 = Replace Array Subset(array=w1517, new element=w1506, index=w1538) -> (w1539:u16[])
            }
            frame "initBlock" {
              n839 = call "myRIO_Brig_RT__Case_Exp_State_initBlock.vi"("input_spout"=w1584, "input_dataExp"=w1582, "input_dataCurrent"=w1583) -> ("output_spout"=w1561:enum16{"Left", "Right"}, "output_state"=w1585:T2, "output_dataExp"=w1581:u16[], "output_dataCurrent"=w1567:u16[], "output_TpB_target"=→"TpB_target":u16)  [unwired: 4 in]
              "cSpout" <- w1561
              n840 = call "myRIO_BRig_RT_dataCurrent_iBlock.vi"() -> ("output_iBlock"=w1566:i32)  [unwired: 11 in]
              n841 = Index Array(array=w1567, index=w1566) -> (element=→"iBlock":u16)
            }
            frame "initBlock2" {
              n842 = local write "nRewards_cur"(u16 0 ("nRewards_cur")) -> ()
              n843 = call "myRIO_BRig_RT__Case_Exp_State_initBlock2.vi"("input_spout"=w1593, "input_dataBlock"=w1594, "input_dataCurrent"=w1592) -> ("idxDataBlock"=w1589:i32, "output_dataBlock"=w1591:u16[][])  [unwired: 7 in]
            }
            frame "initTrial" {
              n844 = call "myRIO_Brig_RT__Case_Exp_State_initTrial.vi"("input_spout"=w1610, "input_dataExp"=w1627, "input_dataCurrent"=w1628) -> ("output_state"=w1629:T2, "output_dataExp"=w1626:u16[], "output_dataCurrent"=w1616:u16[])  [unwired: 6 in]
              n845 = call "myRIO_BRig_RT_dataCurrent_iTrial.vi"() -> ("output_iTrial"=w1615:i32)  [unwired: 11 in]
              n846 = call "myRIO_BRig_RT_dataCurrent_SolenoidReward.vi"() -> ("output_SolenoidReward"=w1609:i32)  [unwired: 11 in]
              n847 = Index Array(array=w1616, index #1=w1615, index #2=w1609) -> (element #1=→"iTrial":u16, element #2=w1608:u16)
              n848 = Not Equal To 0?(x=w1608) -> (x != 0?=→"SolenoidReward":bool)
            }
            frame "initTrial2" {
              # "trialUntilReward"
              n849 = call "myRIO_BRig_RT__Case_Exp_subState_LC__initTrial.vi"("input_dataTrial"=w1636, "input_spout"=w1645, "input_dataCurrent"=w1634, "input_dataLC"=w1633) -> ("output_LC_Wrong"=w1646:bool, "output_LC_led_Wrong"=w1638:bool, "output_LC_Reward"=w1647:bool, "output_LC_led_Reward"=w1637:bool, "output_dataTrial"=w1635:u16[][])  [unwired: 2 in]
              n850 = Equal?(x=w1645, y=enum16{"Left", "Right"}."Right") -> (x = y?=w1643:bool)
              n851 = call "myRIO_BRig_RT_dataExp_ItrialUntilReward.vi"() -> ("output_I_trialUntilReward"=w1641:i32)  [unwired: 11 in]
              n852 = Index Array(array=w1642, index=w1641) -> (element=w1640:u16)
              n853 = Not Equal To 0?(x=w1640) -> (x != 0?=w1639:bool)
              n854 = xnode "Read/Write Control"("FPGA VI Reference In"=w1660, "error in"=w1659, "SelectionState"=FALSE, "laserResponse_reward"=w1647, "laserResponse_wrong"=w1646, "laserResponse_reward_LED"=w1637, "laserResponse_wrong_LED"=w1638, "Left(F)_or_Right(T)"=w1643, "ignoreWrong"=w1639) -> ("error out"=→"error_initTrial":errorcluster)  [unwired: 1 out]
            }
            frame "initTrial3" {
              n855 = call "myRIO_BRig_RT__Case_Exp_State_initTrial_dataTrial.vi"("input_spout"=w1675, "input_dataCurrent"=w1676, "input_dataExp"=w1674, "input_dataTrial"=w1678) -> ("output_dataTrial"=w1677:u16[][], "output_laserPower"=w1671:u16)  [unwired: 6 in]
              n856 = To Double Precision Float(number=w1671) -> (double precision float=w1673:dbl)
              n857 = Divide(x=w1673, y=100.0 ("x")) -> (x/y=w1667:dbl)
              "output_PortA" <- w1667
              n858 = call "myRIO_Brig_RT__covert_Voltage_to_FPGAvalue.vi"("input_voltage"=w1667) -> ("output_PortC"=w1666:i16)  [unwired: 9 in, 1 out]
              n859 = xnode "Read/Write Control"("FPGA VI Reference In"=w1670, "error in"=w1669, "AnaOut_0"=w1666) -> ("error out"=→"error out 4":errorcluster)  [unwired: 1 out]
            }
            frame "initTrial4" {
              n860 = call "myRIO_BRig_RT_dataCurrent_idxDataTrial.vi"() -> ("output_idxDataTrial"=w1701:i32)  [unwired: 11 in]
              n861 = call "myRIO_BRig_RT_dataTrial_activeRecording.vi"() -> ("output_activeRecording"=w1698:i32)  [unwired: 11 in]
              n862 = Index Array(array=w1703, index=w1701) -> (element=w1700:u16)
              n863 = Boolean To (0,1)(Boolean="Recording") -> (0, 1=w1697:i16)
              n864 = To Long Integer(number=w1700) -> (32bit integer=w1699:i32)
              n865 = To Unsigned Word Integer(number=w1697) -> (unsigned 16bit integer=w1696:u16)
              n866 = Replace Array Subset(array=w1702, new element=w1696, index (row)=w1699, index (col)=w1698) -> (w1695:u16[][])
              n867 = local write "Recording_p2"("Recording") -> ()
            }
            frame "initTrial_LC_ENL1" {
              n868 = call "myRIO_BRig_RT__Case_Exp_State_initTrial_LC_ENL1__v2.vi"("input_dataTrial"=w1727, "input_spout"=w1732, "input_dataBlock"=w1725, "input_dataLC"=w1733, "input_dataCurrent"=w1729) -> ("output_LC__ENL1"=w1731:bool, "output_LC_led__ENL1"=w1730:bool, "output_dataTrial"=w1726:u16[][], "output_dataCurrent"=w1728:u16[])  [unwired: 3 in]
            }
            frame "initTrial_LC_Cue1" {
              n869 = local write "Recording_p2"(FALSE ("Recording_p2")) -> ()
              n870 = call "myRIO_BRig_RT__Case_Exp_State_initTrial_LC_Cue1__v2.vi"("input_dataTrial"=w1755, "input_spout"=w1758, "input_dataBlock"=w1753, "input_dataLC"=w1759, "input_dataCurrent"=w1757) -> ("output_LC__Cue1"=w1751:bool, "output_LC_led__Cue1"=w1752:bool, "output_dataTrial"=w1754:u16[][], "output_dataCurrent"=w1756:u16[])  [unwired: 3 in]
            }
            frame "ENL1_pre" {
              # "ENL1_n"
              # "Tcycle"
              # "counter"
              n871 = call "myRIO_BRig_RT_dataCurrent_Tcycle_generic.vi"() -> ("output_Tcycle_generic"=w1805:i32)  [unwired: 11 in]
              n872 = call "myRIO_BRig_RT_dataCurrent_count_generic.vi"() -> ("output_count_generic"=w1807:i32)  [unwired: 11 in]
              n873 = call "myRIO_BRig_RT_dataCurrent_ENL.vi"() -> ("output_ENL"=w1804:i32)  [unwired: 11 in]
              n874 = call "myRIO_BRig_RT_dataCurrent_ENL1_n.vi"() -> ("output_ENL1_n"=w1776:i32)  [unwired: 11 in]
              n875 = Index Array(array=w1798, index #1=w1804, index #2=w1776) -> (element #1=w1803:u16, element #2=w1775:u16)
              n876 = Increment(x=w1775) -> (x+1=w1774:u16)
              n877 = Replace Array Subset(array=w1798, new element #1=u16 0 ("new element/subarray"), index #1=w1807, new element #2=w1803, index #2=w1805, new element #3=w1774, index #3=w1776) -> (w1802:u16[])
              n878 = Select(t=myRIO_BRig_RT__Case_Exp_stateList."ENL1Penalty_pre" ("Enum"), s=w1786, f=myRIO_BRig_RT__Case_Exp_stateList."ENL1" ("Enum")) -> (s? t:f=w1783:T2)
            }
            frame "ENL1" {
              n879 = call "myRIO_BRig_RT__Case_Exp_State_ENL1__v2.vi"("input_LC"=w1814, "I_lick"=w1818, "input_LC_led"=w1815, "input_laserOccurred"=w1810, "input_state"=w1824, "input_dataCurrent"=w1823) -> ("output_trigger_laser_led"=w1813:bool, "output_state"=w1821:T2, "output_dataCurrent"=w1822:u16[], "output_trigger_laser"=w1812:bool)  [unwired: 2 in]
              n880 = Or(x=w1813, y=w1810) -> (x .or. y?=w1816:bool)
            }
            frame "ENL1Penalty_pre" {
              # "Tcycle"
              # "counter"
              n881 = call "myRIO_BRig_RT_dataCurrent_Tcycle_generic.vi"() -> ("output_Tcycle_generic"=w1864:i32)  [unwired: 11 in]
              n882 = call "myRIO_BRig_RT_dataCurrent_count_generic.vi"() -> ("output_count_generic"=w1866:i32)  [unwired: 11 in]
              n883 = call "myRIO_BRig_RT_dataExp_ENL_penalty.vi"() -> ("output_ENL_penalty"=w1859:i32)  [unwired: 11 in]
              n884 = Index Array(array=w1860, index=w1859) -> (element=w1863:u16)
              n885 = Replace Array Subset(array=w1861, new element #1=u16 0 ("new element/subarray"), index #1=w1866, new element #2=w1863, index #2=w1864) -> (w1862:u16[])
            }
            frame "ENL1Penalty" {
              n886 = call "myRIO_BRig_RT__Case_Exp_State_ENL1Penalty.vi"("input_state"=w1889, "input_dataCurrent"=w1893) -> ("output_state"=w1890:T2, "output_dataCurrent"=w1892:u16[])  [unwired: 8 in]
            }
            frame "ENL2_pre" {
            }
            frame "ENL2" {
            }
            frame "ENL2Penalty_pre" {
            }
            frame "ENL2Penalty" {
            }
            frame "Cue1_pre" {
              # "Cue1_n"
              # "Tcycle_Cue1"
              # "0 = L, 1 = R, 2 = both"
              # "sp_R"
              # "sp_L"
              # "Tcycle"
              # "counter"
              n887 = Equal?(x=w2004, y=enum16{"Left", "Right"}."Left") -> (x = y?=w2003:bool)
              n888 = call "myRIO_BRig_RT_dataExp_Audio_sp__L.vi"() -> ("output_Audio_sp__L"=w2002:i32)  [unwired: 11 in]
              n889 = call "myRIO_BRig_RT_dataExp_Audio_sp__R.vi"() -> ("output_Audio_sp__R"=w2001:i32)  [unwired: 11 in]
              n890 = call "myRIO_BRig_RT_dataCurrent_Tcycle_generic.vi"() -> ("output_Tcycle_generic"=w2014:i32)  [unwired: 11 in]
              n891 = call "myRIO_BRig_RT_dataCurrent_count_generic.vi"() -> ("output_count_generic"=w2016:i32)  [unwired: 11 in]
              n892 = Select(t=w2002, s=w2003, f=w2001) -> (s? t:f=w2000:i32)
              n893 = call "myRIO_BRig_RT_dataCurrent_Cue1_n.vi"() -> ("output_Cue1_n"=w1978:i32)  [unwired: 11 in]
              n894 = call "myRIO_BRig_RT_dataCurrent_Tcycle_cue.vi"() -> ("output_Tcycle_cue"=w1987:i32)  [unwired: 11 in]
              n895 = Index Array(array=w2006, index=w2000) -> (element=w1998:u16)
              n896 = Index Array(array=w1988, index #1=w1987, index #2=w1978) -> (element #1=w1989:u16, element #2=w1980:u16)
              n897 = Increment(x=w1980) -> (x+1=w1979:u16)
              n898 = Not Equal To 0?(x=w1998) -> (x != 0?=w1996:bool)
              n899 = Not Equal?(x=w1998, y=u16 1) -> (x != y?=w1997:bool)
              n900 = Replace Array Subset(array=w1988, new element #1=u16 0 ("new element/subarray"), index #1=w2016, new element #2=w1989, index #2=w2014, new element #3=w1979, index #3=w1978) -> (w2013:u16[])
              n901 = Select(t=myRIO_BRig_RT__Case_Exp_stateList."Cue1Penalty_pre" ("Enum"), s=w1984, f=myRIO_BRig_RT__Case_Exp_stateList."Cue1" ("Enum")) -> (s? t:f=w1985:T2)
            }
            frame "Cue1" {
              n902 = call "myRIO_BRig_RT__Case_Exp_State_Cue1__v2.vi"("input_LC"=w2026, "I_lick"=w2029, "input_LC_led"=w2027, "input_laserOccurred"=w2021, "input_state"=w2031, "input_dataCurrent"=w2049) -> ("output_trigger_laser_led"=w2024:bool, "output_state"=w2030:T2, "output_dataCurrent"=w2048:u16[], "output_trigger_laser"=w2025:bool)  [unwired: 2 in]
              n903 = Or(x=w2024, y=w2021) -> (x .or. y?=w2023:bool)
              n904 = Equal?(x=myRIO_BRig_RT__Case_Exp_stateList."Selection_pre", y=w2030) -> (x = y?=w2034:bool)
              n905 = xnode "Read/Write Control"("FPGA VI Reference In"=w2033, "error in"=w2032, "SelectionState"=w2034) -> ()  [unwired: 2 out]
            }
            frame "Cue1Penalty_pre" {
              # "Tcycle"
              # "counter"
              n906 = call "myRIO_BRig_RT_dataCurrent_Tcycle_generic.vi"() -> ("output_Tcycle_generic"=w2080:i32)  [unwired: 11 in]
              n907 = call "myRIO_BRig_RT_dataCurrent_count_generic.vi"() -> ("output_count_generic"=w2082:i32)  [unwired: 11 in]
              n908 = call "myRIO_BRig_RT_dataExp_Tcycle_CuePenalty.vi"() -> ("output_Tcycle_CuePenalty"=w2079:i32)  [unwired: 11 in]
              n909 = Index Array(array=w2074, index=w2079) -> (element=w2078:u16)
              n910 = Replace Array Subset(array=w2076, new element #1=u16 0 ("new element/subarray"), index #1=w2082, new element #2=w2078, index #2=w2080) -> (w2075:u16[])
            }
            frame "Cue1Penalty" {
              # "reset laserOccurred"
              n911 = call "myRIO_BRig_RT__Case_Exp_State_Cue1Penalty.vi"("input_state"=w2106, "input_dataCurrent"=w2107) -> ("output_state"=w2104:T2, "output_dataCurrent"=w2105:u16[])  [unwired: 8 in]
            }
            frame "Cue2_pre" {
              n912 = call "myRIO_BRig_RT__Case_Exp_subState_LC__Cue2.vi"("input_spout"=w2124, "input_dataCurrent"=w2125, "input_dataLC"=w2123) -> ()  [unwired: 6 in, 2 out]
            }
            frame "Cue2" {
            }
            frame "Cue2Penalty_pre" {
            }
            frame "Cue2Penalty" {
            }
            frame "Selection_pre" {
              # "Tcycle"
              # "counter"
              n913 = xnode "Read/Write Control"("FPGA VI Reference In"=w2196, "error in"=w2197) -> ("error out"=→"error_Selection_pre":errorcluster, "SelectReward"=w2189:bool, "SelectWrong"=w2191:bool)  [unwired: 1 out]
              n914 = call "myRIO_BRig_RT_dataCurrent_Tcycle_generic.vi"() -> ("output_Tcycle_generic"=w2218:i32)  [unwired: 11 in]
              n915 = call "myRIO_BRig_RT_dataCurrent_count_generic.vi"() -> ("output_count_generic"=w2220:i32)  [unwired: 11 in]
              n916 = call "myRIO_BRig_RT_dataExp_Tcycle_Selection.vi"() -> ("output_Tcycle_Selection"=w2217:i32)  [unwired: 11 in]
              n917 = Index Array(array=w2214, index=w2217) -> (element=w2216:u16)
              n918 = Replace Array Subset(array=w2212, new element #1=u16 0 ("new element/subarray"), index #1=w2220, new element #2=w2216, index #2=w2218) -> (w2215:u16[])
              n919 = Or(x=w2189, y=w2191) -> (x .or. y?=w2190:bool)
              n920 = Select(t=myRIO_BRig_RT__Case_Exp_stateList."SelectReward_pre" ("Enum"), s=w2189, f=myRIO_BRig_RT__Case_Exp_stateList."SelectWrong_pre" ("Enum")) -> (s? t:f=w2195:T2)
              n921 = Select(t=w2195, s=w2190, f=myRIO_BRig_RT__Case_Exp_stateList."Selection" ("Enum")) -> (s? t:f=w2192:T2)
            }
            frame "Selection" {
              # "counter\nSelection"
              # "increment"
              # "get Tcycle"
              # "get count"
              n922 = xnode "Read/Write Control"("FPGA VI Reference In"=w2245, "error in"=w2244) -> ("error out"=→"error_Selection":errorcluster, "SelectReward"=w2241:bool, "SelectWrong"=w2242:bool)  [unwired: 1 out]
              n923 = call "myRIO_BRig_RT_dataCurrent_Tcycle_generic.vi"() -> ("output_Tcycle_generic"=w2238:i32)  [unwired: 11 in]
              n924 = call "myRIO_BRig_RT_dataCurrent_count_generic.vi"() -> ("output_count_generic"=w2231:i32)  [unwired: 11 in]
              n925 = Index Array(array=w2239, index #1=w2238, index #2=w2231) -> (element #1=w2230:u16, element #2=w2237:u16)
              n926 = call "myRIO_BRig_RT__increment_u16.vi"() -> ("output_increment__u16"=w2236:u16)  [unwired: 11 in]
              n927 = Add(x=w2237, y=w2236) -> (x+y=w2232:u16)
              n928 = Greater?(x=w2230, y=w2232) -> (0:w2224:bool)
              n929 = Select(t=w2235, s=w2224, f=myRIO_BRig_RT__Case_Exp_stateList."SelectTimeout_pre" ("Enum")) -> (s? t:f=w2225:T2)
              n930 = Select(t=w2232, s=w2224, f=w2230) -> (s? t:f=w2228:u16)
              n931 = call "myRIO_BRig_RT_dataCurrent_count_selection.vi"() -> ("output_count_generic"=w2229:i32)  [unwired: 11 in]
              n932 = Select(t=myRIO_BRig_RT__Case_Exp_stateList."SelectReward_pre" ("Enum"), s=w2241, f=myRIO_BRig_RT__Case_Exp_stateList."SelectWrong_pre" ("Enum")) -> (s? t:f=w2240:T2)
              n933 = Replace Array Subset(array=w2239, new element #1=w2228, index #1=w2231, new element #2=w2228, index #2=w2229) -> (w2234:u16[])
              n934 = Or(x=w2241, y=w2242) -> (x .or. y?=w2223:bool)
              n935 = Select(t=w2240, s=w2223, f=w2225) -> (s? t:f=w2243:T2)
            }
            frame "SelectReward_pre" {
              # "iState"
              # "Tcycle\nReward"
              # "nRewTrials"
              # "Tcycle\nGeneric"
              # "counter"
              n936 = call "myRIO_BRig_RT_dataCurrent_nRewTrials.vi"() -> ("output_nRewTrials"=w2277:i32)  [unwired: 11 in]
              n937 = Equal?(x=w2286, y=enum16{"Left", "Right"}."Left") -> (x = y?=w2287:bool)
              n938 = Index Array(array=w2278, index=w2277) -> (element=w2276:u16)
              n939 = call "myRIO_BRig_RT_dataExp_Tcycle_Reward__L.vi"() -> ("output_Tcycle_Reward__L"=w2290:i32)  [unwired: 11 in]
              n940 = call "myRIO_BRig_RT_dataExp_Tcycle_Reward__R.vi"() -> ("output_Tcycle_Reward__R"=w2291:i32)  [unwired: 11 in]
              n941 = Increment(x=w2276) -> (x+1=w2275:u16)
              n942 = Select(t=w2290, s=w2287, f=w2291) -> (s? t:f=w2289:i32)
              n943 = call "myRIO_BRig_RT__Case_Exp_subState_LC__Reward.vi"("input_spout"=w2286, "input_dataCurrent"=w2278, "input_dataLC"=w2285) -> ()  [unwired: 6 in, 2 out]
              n944 = call "myRIO_BRig_RT_dataCurrent_count_generic.vi"() -> ("output_count_generic"=w2280:i32)  [unwired: 11 in]
              n945 = call "myRIO_BRig_RT_dataCurrent_Tcycle_generic.vi"() -> ("output_Tcycle_generic"=w2281:i32)  [unwired: 11 in]
              n946 = Index Array(array=w2292, index=w2289) -> (element=w2282:u16)
              n947 = call "myRIO_BRig_RT_dataCurrent_iState.vi"() -> ("output_iState"=w2270:i32)  [unwired: 11 in]
              n948 = Replace Array Subset(array=w2278, new element #1=w2275, index #1=w2277, new element #2=u16 0 ("new element/subarray"), index #2=w2280, new element #3=w2282, index #3=w2281, new element #4=u16 1 ("new element/subarray"), index #4=w2270) -> (w2293:u16[])
            }
            frame "SelectReward" {
              n949 = call "myRIO_BRig_RT__Case_Exp_State_Reward.vi"("input_dataCurrent"=w2314, "input_state"=w2311, "input_spout"=w2309) -> ("output_dataCurrent"=w2313:u16[], "output_state"=w2312:T2, "output__L"=w2307:bool, "output__R"=w2308:bool)  [unwired: 9 in]
            }
            frame "SelectRewardPost_pre" {
              # "nRewards"
              # "nRewTrials"
              # "Tcycle"
              # "counter"
              n950 = call "myRIO_BRig_RT_dataBlock_nRewards__L.vi"() -> ("output_nRewards__L"=w2330:i32)  [unwired: 11 in]
              n951 = call "myRIO_BRig_RT_dataBlock_nRewards__R.vi"() -> ("output_nRewards__R"=w2329:i32)  [unwired: 11 in]
              n952 = call "myRIO_BRig_RT_dataCurrent_Tcycle_generic.vi"() -> ("output_Tcycle_generic"=w2349:i32)  [unwired: 11 in]
              n953 = call "myRIO_BRig_RT_dataCurrent_count_generic.vi"() -> ("output_count_generic"=w2351:i32)  [unwired: 11 in]
              n954 = case shown="\"Left\", Default" w2323 {
                tunnel: w2335 -> [w2356 w2360]
                tunnel: [w2355 w2360] -> w2334
                tunnel: [w2357 w2358] -> w2333
                tunnel: w2332 -> [w2357 w2359]
                frame "Left", Default {
                  n955 = Increment(x=w2356) -> (x+1=w2355:u16)
                }
                frame "Right" {
                  n956 = Increment(x=w2359) -> (x+1=w2358:u16)
                }
              }
              "nRewards_Left" <- w2334
              "nRewards_Right" <- w2333
              n957 = Equal?(x=w2323, y=enum16{"Left", "Right"}."Left") -> (x = y?=w2322:bool)
              n958 = Select(t=w2330, s=w2322, f=w2329) -> (s? t:f=w2328:i32)
              n959 = call "myRIO_BRig_RT_dataExp_Tcycle_RewardPost.vi"() -> ("output_Tcycle_RewardPost"=w2345:i32)  [unwired: 11 in]
              n960 = call "myRIO_BRig_RT_dataCurrent_nRewTrials.vi"() -> ("output_nRewTrials"=w2331:i32)  [unwired: 11 in]
              n961 = Index Array(array=w2346, index=w2345) -> (element=w2348:u16)
              n962 = Index Array(array=w2325, index=w2331) -> (element=w2320:u16)
              n963 = Replace Array Subset(array=w2325, new element #1=u16 0 ("new element/subarray"), index #1=w2351, new element #2=w2348, index #2=w2349) -> (w2347:u16[])
              n964 = Replace Array Subset(array=w2327, new element=w2320, index (row)=w2321, index (col)=w2328) -> (w2326:u16[][])
              n965 = local write "nRewards_cur"(w2320) -> ()
            }
            frame "SelectRewardPost" {
              n966 = call "myRIO_BRig_RT__Case_Exp_State_RewardPost.vi"("input_state"=w2375, "input_dataCurrent"=w2378) -> ("output_state"=w2376:T2, "output_dataCurrent"=w2377:u16[])  [unwired: 8 in]
            }
            frame "SelectWrong_pre" {
              # "iState"
              # "Tcycle"
              # "counter"
              n967 = call "myRIO_BRig_RT_dataCurrent_Tcycle_generic.vi"() -> ("output_Tcycle_generic"=w2403:i32)  [unwired: 11 in]
              n968 = call "myRIO_BRig_RT_dataCurrent_count_generic.vi"() -> ("output_count_generic"=w2405:i32)  [unwired: 11 in]
              n969 = call "myRIO_BRig_RT_dataExp_Tcycle_Wrong.vi"() -> ("output_Tcycle_Wrong"=w2401:i32)  [unwired: 11 in]
              n970 = call "myRIO_BRig_RT__Case_Exp_subState_LC__Wrong.vi"("input_spout"=w2397, "input_dataCurrent"=w2398, "input_dataLC"=w2395) -> ()  [unwired: 6 in, 2 out]
              n971 = Index Array(array=w2399, index=w2401) -> (element=w2402:u16)
              n972 = call "myRIO_BRig_RT_dataCurrent_iState.vi"() -> ("output_iState"=w2389:i32)  [unwired: 11 in]
              n973 = Replace Array Subset(array=w2398, new element #1=u16 0 ("new element/subarray"), index #1=w2405, new element #2=w2402, index #2=w2403, new element #3=u16 2 ("new element/subarray"), index #3=w2389) -> (w2400:u16[])
            }
            frame "SelectWrong" {
              n974 = call "myRIO_BRig_RT__Case_Exp_State_Wrong.vi"("input_state"=w2419, "input_dataCurrent"=w2428) -> ("output_state"=w2416:T2, "output_dataCurrent"=w2427:u16[])  [unwired: 8 in]
              n975 = Not Equal?(x=w2419, y=w2416) -> (x != y?=w2418:bool)
              n976 = Select(t=myRIO_BRig_RT__Case_Exp_stateList."SelectWrong_post" ("Enum"), s=w2418, f=w2416) -> (s? t:f=w2415:T2)
            }
            frame "SelectWrong_post" {
            }
            frame "SelectTimeout_pre" {
              # "iState"
              # "Tcycle"
              # "counter"
              n977 = xnode "Read/Write Control"("FPGA VI Reference In"=w2455, "error in"=w2454, "SelectionState"=FALSE) -> ("error out"=→"error out 3":errorcluster)  [unwired: 1 out]
              n978 = call "myRIO_BRig_RT_dataCurrent_Tcycle_generic.vi"() -> ("output_Tcycle_generic"=w2477:i32)  [unwired: 11 in]
              n979 = call "myRIO_BRig_RT_dataCurrent_count_generic.vi"() -> ("output_count_generic"=w2475:i32)  [unwired: 11 in]
              n980 = call "myRIO_BRig_RT_dataExp_Tcycle_Timeout.vi"() -> ("output_Tcycle_Timeout"=w2479:i32)  [unwired: 11 in]
              n981 = call "myRIO_BRig_RT__Case_Exp_subState_LC__Timeout.vi"("input_spout"=w2470, "input_dataCurrent"=w2471, "input_dataLC"=w2469) -> ()  [unwired: 6 in, 2 out]
              n982 = Index Array(array=w2473, index=w2479) -> (element=w2478:u16)
              n983 = call "myRIO_BRig_RT_dataCurrent_iState.vi"() -> ("output_iState"=w2463:i32)  [unwired: 11 in]
              n984 = Replace Array Subset(array=w2471, new element #1=u16 0 ("new element/subarray"), index #1=w2475, new element #2=w2478, index #2=w2477, new element #3=u16 3 ("new element/subarray"), index #3=w2463) -> (w2474:u16[])
            }
            frame "SelectTimeout" {
              n985 = call "myRIO_BRig_RT__Case_Exp_State_Timeout.vi"("input_dataLC"=w2498, "input_LC"=w2499, "input_state"=w2489, "input_dataCurrent"=w2504) -> ("output_state"=w2490:T2, "output_dataCurrent"=w2503:u16[])  [unwired: 5 in, 1 out]
              n986 = Not Equal?(x=w2489, y=w2490) -> (x != y?=w2493:bool)
              n987 = Select(t=myRIO_BRig_RT__Case_Exp_stateList."SelectTimeout_post" ("Enum"), s=w2493, f=w2490) -> (s? t:f=w2491:T2)
            }
            frame "SelectTimeout_post" {
            }
            frame "endTrial1" {
              # "Update dataBlock"
              n988 = call "myRIO_BRig_RT__Case_Exp_State_endTrial1.vi"("input_spout"=w2537, "input_dataBlock"=w2536, "input_dataCurrent"=w2534) -> ("output_dataBlock"=w2535:u16[][], "output_dataCurrent"=w2533:u16[])  [unwired: 7 in]
            }
            frame "endTrial2" {
              # "update dataTrial"
              n989 = call "myRIO_BRig_RT__Case_Exp_State_endTrial2.vi"("input_spout"=w2556, "input_dataTrial"=w2560, "input_dataCurrent"=w2558) -> ("output_dataTrial"=w2559:u16[][], "output_dataCurrent"=w2557:u16[])  [unwired: 7 in]
            }
            frame "endTrial3" {
              w2586 = myRIO_BRig_RT__Case_Exp_stateList."endBlock" ("Enum")
              # "nRewTrials"
              # "iTrial"
              # "I_blockUntilReward"
              # "TPB"
              # "end block?"
              n990 = local read "STOP_endTrial"() -> (w2584:bool)
              n991 = local read "STOP_abort"() -> (w2583:bool)
              n992 = xnode "Read/Write Control"("FPGA VI Reference In"=w2572, "error in"=w2571, "SelectionState"=FALSE) -> ("error out"=→"error out 2":errorcluster)  [unwired: 1 out]
              n993 = local read "START"() -> (w2581:bool)
              n994 = call "myRIO_BRig_RT_dataExp_IblockUntilReward.vi"() -> ("output_I_blockUntilReward"=w2593:i32)  [unwired: 11 in]
              n995 = Index Array(array=w2577, index=w2593) -> (element=w2573:u16)
              n996 = Not(x=w2581) -> (.not. x?=w2582:bool)
              n997 = Not Equal To 0?(x=w2573) -> (x != 0?=w2591:bool)
              n998 = Compound Arithmetic op=OR(w2584, w2582, w2583) -> (w2585:bool)
              n999 = call "myRIO_BRig_RT_dataCurrent_nRewTrials.vi"() -> ("output_nRewTrials"=w2589:i32)  [unwired: 11 in]
              n1000 = call "myRIO_BRig_RT_dataCurrent_iTrial.vi"() -> ("output_iTrial"=w2590:i32)  [unwired: 11 in]
              n1001 = Select(t=w2589, s=w2591, f=w2590) -> (s? t:f=w2588:i32)
              n1002 = call "myRIO_BRig_RT_dataCurrent_TpB.vi"() -> ("output_TpB"=w2592:i32)  [unwired: 11 in]
              n1003 = Index Array(array=w2578, index #1=w2592, index #2=w2588) -> (element #1=w2579:u16, element #2=w2580:u16)
              n1004 = Less Or Equal?(x=w2579, y=w2580) -> (x <= y?=w2576:bool)
              n1005 = Select(t=w2586, s=w2576, f=myRIO_BRig_RT__Case_Exp_stateList."empty_endTrial1" ("Enum")) -> (s? t:f=w2587:T2)
              n1006 = Select(t=w2586, s=w2585, f=w2587) -> (s? t:f=w2574:T2)
            }
            frame "endBlock" {
              # "R"
              # "L"
              # "idxDataBlock"
              n1007 = Equal?(x=w2617, y=enum16{"Left", "Right"}."Left") -> (x = y?=w2616:bool)
              n1008 = call "myRIO_BRig_RT_dataCurrent_idxDataBlockL.vi"() -> ("output_idxDataBlock__L"=w2620:i32)  [unwired: 11 in]
              n1009 = call "myRIO_BRig_RT_dataCurrent_idxDataBlockR.vi"() -> ("output_idxDataBlock__R"=w2619:i32)  [unwired: 11 in]
              n1010 = Increment(x=w2611) -> (x+1=w2610:i32)
              n1011 = Select(t=w2620, s=w2616, f=w2619) -> (s? t:f=w2614:i32)
              n1012 = To Unsigned Word Integer(number=w2610) -> (unsigned 16bit integer=w2612:u16)
              n1013 = local read "START"() -> (w2640:bool)
              n1014 = local read "STOP_endBlock"() -> (w2635:bool)
              n1015 = local read "STOP_endTrial"() -> (w2638:bool)
              n1016 = local read "STOP_abort"() -> (w2637:bool)
              n1017 = Replace Array Subset(array=w2615, new element=w2612, index=w2614) -> (w2613:u16[])
              n1018 = Not(x=w2640) -> (.not. x?=w2639:bool)
              n1019 = Compound Arithmetic op=OR(w2639, w2635, w2638, w2637) -> (w2636:bool)
              n1020 = Select(t=myRIO_BRig_RT__Case_Exp_stateList."endExp" ("Enum"), s=w2636, f=myRIO_BRig_RT__Case_Exp_stateList."empty_endBlock1" ("Enum")) -> (s? t:f=w2644:T2)
            }
            frame "endExp" {
            }
            frame "commConnect" {
              n1021 = call "myRIO_BRig_RT_comm_webdav_connect.vi"("input_password"="Host Password", "input_username"="Host UserName") -> ("output_Iconnected"=w2665:bool, "output_hSession"=w2683:T6)  [unwired: 7 in, 1 out]
              "Connected To Host?" <- w2665
              n1022 = case shown="False" w2665 {
                frame False {
                  n1023 = One Button Dialog(message="Connection Failed!\nData not being saved!") -> ()  [unwired: 1 in, 1 out]
                }
                frame True {
                }
              }
            }
            frame "commUpload_pre" {
              n1024 = Select(t=myRIO_BRig_RT__Case_Exp_stateList."commUpload_dataBlock" ("Enum"), s=w2690, f=myRIO_BRig_RT__Case_Exp_stateList."endTrial3") -> (s? t:f=w2688:T2)
            }
            frame "commUpload_dataBlock" {
              n1025 = call "myRIO_BRig_RT_comm_webdav_uploadFile__data.vi"("input_fileName_prefix"=w2711, "input_fileName"="dataBlock" ("input_filename"), "input_hSession"=w2713) -> ()  [unwired: 8 in, 1 out]
            }
            frame "commUpload_dataCurrent" {
              n1026 = call "myRIO_BRig_RT_comm_webdav_uploadFile__data.vi"("input_fileName_prefix"=w2732, "input_fileName"="dataCurrent" ("input_filename"), "input_hSession"=w2734) -> ()  [unwired: 8 in, 1 out]
            }
            frame "commUpload_dataExp" {
              n1027 = call "myRIO_BRig_RT_comm_webdav_uploadFile__data.vi"("input_fileName_prefix"=w2753, "input_fileName"="dataExp" ("input_filename"), "input_hSession"=w2755) -> ()  [unwired: 8 in, 1 out]
            }
            frame "commUpload_dataLC" {
              n1028 = call "myRIO_BRig_RT_comm_webdav_uploadFile__data.vi"("input_fileName_prefix"=w2774, "input_fileName"="dataLC" ("input_filename"), "input_hSession"=w2776) -> ()  [unwired: 8 in, 1 out]
            }
            frame "commUpload_dataTrial" {
              n1029 = call "myRIO_BRig_RT_comm_webdav_uploadFile__data.vi"("input_fileName_prefix"=w2798, "input_fileName"="dataTrial" ("input_filename"), "input_hSession"=w2800) -> ()  [unwired: 8 in, 1 out]
            }
            frame "saveData_dataBlock" {
              # "idxDataBlockR"
              # "idxDataBlockL"
              n1030 = call "myRIO_BRig_RT_dataCurrent_idxDataBlockL.vi"() -> ("output_idxDataBlock__L"=w2824:i32)  [unwired: 11 in]
              n1031 = call "myRIO_BRig_RT_dataCurrent_idxDataBlockR.vi"() -> ("output_idxDataBlock__R"=w2825:i32)  [unwired: 11 in]
              n1032 = Index Array(array=w2826, index #1=w2824, index #2=w2825) -> (element #1=w2823:u16, element #2=w2822:u16)
              n1033 = Greater?(x=w2823, y=w2822) -> (0:w2821:bool)
              n1034 = Select(t=w2823, s=w2821, f=w2822) -> (s? t:f=w2819:u16)
              n1035 = Increment(x=w2819) -> (x+1=w2818:u16)
              n1036 = To Long Integer(number=w2818) -> (32bit integer=w2817:i32)
              n1037 = Array Subset(array=w2820, length (row)=w2817) -> (w2816:u16[][])  [unwired: 3 in]
              n1038 = call "myRIO_BRig_RT_comm_webdav_saveArrayToFile__2D_u16.vi"("Array"=w2816, "input_filename"="dataBlock") -> ()  [unwired: 10 in]
            }
            frame "saveData_dataCurrent" {
              n1039 = call "myRIO_BRig_RT_comm_webdav_saveArrayToFile__1D_u16.vi"("Array"=w2845, "input_filename"="dataCurrent") -> ()  [unwired: 10 in]
            }
            frame "saveData_dataExp" {
              # "runTime"
              n1040 = Get Date/Time In Seconds() -> (seconds since 1Jan1904=w2873:timestamp)
              n1041 = To Double Precision Float(number=w2873) -> (double precision float=w2872:dbl)
              n1042 = call "myRIO_BRig_RT_dataExp_runTime_seconds.vi"() -> ("output_RunTime_minutes"=w2871:i32)  [unwired: 11 in]
              n1043 = Subtract(x=w2872, y=w2870) -> (x-y=w2867:dbl)
              n1044 = To Unsigned Word Integer(number=w2867) -> (unsigned 16bit integer=w2866:u16)
              n1045 = Replace Array Subset(array=w2865, new element=w2866, index=w2871) -> (w2868:u16[])
              n1046 = call "myRIO_BRig_RT_comm_webdav_saveArrayToFile__1D_u16.vi"("Array"=w2868, "input_filename"="dataExp") -> ()  [unwired: 10 in]
            }
            frame "saveData_dataLC" {
              n1047 = call "myRIO_BRig_RT_comm_webdav_saveArrayToFile__1D_u16.vi"("Array"=w2892, "input_filename"="dataLC") -> ()  [unwired: 10 in]
            }
            frame "saveData_dataTrial" {
              # "idxTrial"
              n1048 = call "myRIO_BRig_RT_dataCurrent_idxDataTrial.vi"() -> ("output_idxDataTrial"=w2917:i32)  [unwired: 11 in]
              n1049 = Index Array(array=w2918, index=w2917) -> (element=w2914:u16)
              n1050 = Increment(x=w2914) -> (x+1=w2913:u16)
              n1051 = To Long Integer(number=w2913) -> (32bit integer=w2912:i32)
              n1052 = Array Subset(array=w2915, length (row)=w2912) -> (w2916:u16[][])  [unwired: 3 in]
              n1053 = call "myRIO_BRig_RT_comm_webdav_saveArrayToFile__2D_u16.vi"("Array"=w2916, "input_filename"="dataTrial") -> ()  [unwired: 10 in]
            }
            frame "empty_endBlock1" {
            }
            frame "empty_endBlock2" {
            }
            frame "empty_endTrial1" {
            }
            frame "empty_endTrial2" {
            }
            frame "empty_endTrial3" {
            }
            frame "empty_endTrial4" {
            }
            frame "empty_endTrial5" {
            }
          }
          n1054 = case shown="True" w1066 {
            tunnel: w1062 -> [w1089 w1097]
            tunnel: w1065 -> [_ w1093]
            tunnel: w1064 -> [_ w1092]
            tunnel: w1063 -> [_ w1091]
            tunnel: w1032 -> [_ w1090]
            tunnel: [w1089 w1096] -> w1061
            tunnel: w1060 -> [w1088 w1095]
            tunnel: [w1088 w1094] -> w1059
            frame False {
            }
            frame True {
              n1055 = call "myRIO_BRig_RT__Case_Exp__recordLick.vi"("intput_state__trialEnd"=w1090, "intput_state__trialStart"=w1091, "input_lick__R"=w1092, "input_lick__L"=w1093, "input_dataCurrent"=w1095, "input_dataLick"=w1097) -> ("output_dataCurrent"=w1094:u16[], "output_dataLick"=w1096:u16[][])  [unwired: 4 in]
            }
          }
          n1056 = Or(x=w1034, y=w1035) -> (x .or. y?=w1021:bool)
          n1057 = Or(x=w1038, y=w1018) -> (x .or. y?=w1007:bool)
          n1058 = Or(x=w1017, y=w1039) -> (x .or. y?=w1033:bool)
          n1059 = Or(x=w1037, y=w1036) -> (x .or. y?=w1022:bool)
          n1060 = Or(x=w1067, y="STOP_abort") -> (x .or. y?=w1069:bool)
          n1061 = Or(x=w996, y=w997) -> (x .or. y?=w994:bool)
          n1062 = Or(x=w998, y=w997) -> (x .or. y?=w995:bool)
          n1063 = xnode "Read/Write Control"("FPGA VI Reference In"=w1009, "error in"=w1008, "A1_SR"=w1022, "A3_SL"=w1021, "A6_Act"="Recording_p2", "audioTrigger_L"=w1007, "audioAmp_L"=w1048, "audioFreq_L_kHz"=w1016, "audioTrigger_R"=w1033, "audioAmp_R"=w1049, "audioFreq_R_kHz"=w1050, "laserledMTrig"=w994, "laserMTrig"=w995) -> ("FPGA VI Reference Out"=w1058:refnum<k20>, "error out"=w1057:errorcluster)
          n1064 = node-c288() -> ()  [unwired: 1 in, 1 out]
          "cState" <- w1063
        }
        n1065 = node-c288(w952) -> ()  [unwired: 1 out]
        n1066 = flat-sequence {
          tunnel: w948 -> [w986]
          tunnel: w947 -> [w985]
          tunnel: [w984] -> w940
          tunnel: [w983] -> w939
          tunnel: [w989] -> w941
          tunnel: [w990] -> w946
          tunnel: w940 -> [w990]
          tunnel: w939 -> [w989]
          frame #0 {
            w980 = u8 0
            w981 = u16 0 ("AudioLeft_phase_inc")
            w982 = FALSE
            n1067 = xnode "Read/Write Control"("FPGA VI Reference In"=w986, "error in"=w985, "Counts_Reset"=TRUE, "audioTrigger_L"=w982, "audioFreq_L_kHz"=w980, "audioAmp_L"=w981, "audioTrigger_R"=w982, "audioFreq_R_kHz"=w980, "audioAmp_R"=w981, "A3_SL"=w982, "A1_SR"=w982, "A6_Act"=w982) -> ("FPGA VI Reference Out"=w984:refnum<k20>, "error out"=w983:errorcluster)
          }
          frame #1 {
            w988 = FALSE ("START")
            n1068 = local write "START"(w988) -> ()
            n1069 = local write "STOP_endTrial"(w988) -> ()
            n1070 = local write "STOP_endBlock"(w988) -> ()
          }
        }
        n1071 = stacked-sequence {
          tunnel: w924 -> [w960 _]
          tunnel: w922 -> [w961 _]
          tunnel: w921 -> [_ w966]
          tunnel: w920 -> [_ w965]
          tunnel: w919 -> [_ w964]
          tunnel: w918 -> [w954 _]
          frame #0 {
            n1072 = call "myRIO_BRig_RT_dataCurrent_idxDataLick.vi"() -> ("output_idxDataLick"=w955:i32)  [unwired: 11 in]
            n1073 = Index Array(array=w954, index=w955) -> (element=w957:u16)
            n1074 = Increment(x=w957) -> (x+1=w958:u16)
            n1075 = call "myRIO_BRig_RT_comm_webdav_saveArrayToFile__1D_u16.vi"("Array"=w961, "input_filename"="dataMTrig") -> ()  [unwired: 10 in]
            n1076 = To Long Integer(number=w958) -> (32bit integer=w956:i32)
            n1077 = Array Subset(array=w960, length (row)=w956) -> (w959:u16[][])  [unwired: 3 in]
            n1078 = call "myRIO_BRig_RT_comm_webdav_saveArrayToFile__2D_u16.vi"("Array"=w959, "input_filename"="dataLick") -> ()  [unwired: 10 in]
          }
          frame #1 {
            n1079 = case shown="True" w966 {
              tunnel: w965 -> [_ w968]
              tunnel: w964 -> [_ w967]
              frame False {
              }
              frame True {
                n1080 = stacked-sequence {
                  tunnel: w968 -> [w970 w977 w979]
                  tunnel: w967 -> [w971 w976 _]
                  frame #0 {
                    n1081 = call "myRIO_BRig_RT_comm_webdav_uploadFile__announce.vi"("input_addText"=TRUE, "input_fileName_prefix"=w971, "intput_fileName"="curExp_end", "intput_hSession"=w970) -> ("output_Isuccess"=w969:bool)  [unwired: 6 in, 1 out]
                    n1082 = case shown="True" w969 {
                      frame False {
                        n1083 = One Button Dialog(message="!!! Warning !!! Your data is located at C:\\BehaviorRig\\commTransfer") -> ()  [unwired: 1 in, 1 out]
                      }
                      frame True {
                        n1084 = Wait (ms)(milliseconds to wait=u32 20) -> ()  [unwired: 1 out]
                      }
                    }
                  }
                  frame #1 {
                    n1085 = call "myRIO_BRig_RT__endExp_sendData.vi"("input_fileName_prefix"=w976, "input_hSession"=w977) -> ()  [unwired: 8 in, 2 out]
                  }
                  frame #2 {
                    n1086 = local write "Connected To Host?"(FALSE ("Connected To Host?")) -> ()
                    n1087 = call <vilib>:"Close Session.vi"("session handle"=w979) -> ()  [unwired: 14 in, 1 out]
                  }
                }
              }
            }
          }
        }
      }
    }
    n1088 = local read "STOP_abort"() -> (w30:bool)
  }
  n1089 = xnode "Read/Write Control"("FPGA VI Reference In"=w8, "error in"=w7, "FPGA_Stop"=TRUE) -> ("FPGA VI Reference Out"=w13:refnum<k20>, "error out"=w14:errorcluster)
  n1090 = xnode "Close FPGA VI Reference"("FPGA VI Reference In"=w13, "error in"=w14) -> ("error out"=w12:errorcluster)
  n1091 = call <vilib>:"Reset myRIO.vi"("error in (no error)"=w12) -> ()  [unwired: 10 in, 1 out]
